vi "myRIO_BRig_RT_v0,72__PortC.vi"() -> ()   [LabVIEW 2014]
uses:
  <vilib>/Platform/TimedLoop/XDataNode/XDataNode.xnode
  <vilib>/Platform/TimedLoop/XDataNode/nitl_modes.ctl
  <vilib>/Platform/TimedLoop/XDataNode/XDNodeRunTimeDep.lvlib
  <vilib>/Platform/TimedLoop/XDataNode/wakeup.ctl
  <vilib>/Platform/TimedLoop/XDataNode/timing_clust.ctl
  <vilib>/rvi/interface/nirviReadWriteControl/nirviReadWriteControl.xnode
  <vilib>/rvi/interface/Simulation/niFpgaSimulationCallBeginRW.vi
  <vilib>/rvi/errors/niLvFpgaAdjustHostInterfaceError.vi
  <vilib>/rvi/interface/nirviCloseFPGA/nirviCloseFPGA.xnode
  <vilib>/myRIO/Instrument Drivers/Utilities/Utilities.lvlib
  <vilib>/rvi/interface/nirviOpenFPGA/nirviOpenFPGA.xnode
  myRIO_BRig_RT__Case_Exp_stateList.ctl
  <vilib>/WebDAVClient/Advanced/SessionHandle.ctl
  <vilib>/WebDAVClient/NI_WebDAV.lvlib
  myRIO_BRig_RT__Case_NonExp_stateList.ctl
  NiFpgaLv.dll
  <vilib>/Utility/error.llb/Error Cluster From Error Code.vi
  myRIO_BRig_FPGA_v3,60__PortC__build.lvbitx
  myRIO_BRig_FPGA_v3,60__PortC.vi
  <vilib>/FPGAPlugInAG/myRIO-1900/niLvFpga_Open_myRIO-1900.vi
  <vilib>/rvi/interface/common/dynamic/niFpgaDynamicAddResources.vi
  <vilib>/FPGAPlugInAG/Dynamic/niLvFpga_Close_Dynamic.vi
panel:
  in  "LC_Sel_All_Count":u16
  in  "LC_Sel_First_Count":u16
  in  "LC_Sel_All_Probability":u16
  in  "LC_Sel_All_Block":u16(slide) max=2 step=1 scale=0.0..2.0
  in  "LC_Sel_All_OnOff":bool
  in  "LC_Sel_First_Probability":u16
  in  "LC_Sel_First_Block":u16(slide) max=2 step=1 scale=0.0..2.0
  in  "LC_Sel_First_OnOff":bool
  in  "LC_Sel_All_Tdelay":u16
  in  "LC_Sel_First_Tdelay":u16
  out "I_connect_TCP":bool
  out "tempAI0":i16
  out "error out 5":errorcluster
  in  "get_countPerMS":bool
  in  "count_warmup_R_reset":bool
  in  "count_warmup_L_reset":bool
  out "count_warmup_R":u16
  out "count_warmup_L":u16
  out "SolenoidReward":bool
  in  "SolenoidProbability_L":u16=50 caption="Reward Time [ms]" min=1 max=1000 step=1
  in  "SolenoidProbability_R":u16=50 caption="Reward Time [ms]" min=1 max=1000 step=1
  out "output_PortA":dbl caption="LaserPower"
  out "error out 4":errorcluster
  in  "laser_power_step":dbl
  in  "laser_power_max":dbl
  in  "Recording":bool
  out "error out 3":errorcluster
  out "error out 2":errorcluster
  in  "laser_power_min":dbl
  in  "f_millisec2count":dbl=159.0
  in  "laser_Tshutter":dbl=2.0
  in  "laser_Freq":dbl=10.0
  in  "laser_Tpeak":dbl=2.0
  in  "laser_duration":u16
  out "error out":errorcluster
  in  "LC_Cue1_All_Count":u16
  in  "LC_Cue1_First_Count":u16
  in  "LC_Cue1_All_delayOpt":bool
  in  "LC_ENL1_All_delayOpt":bool
  in  "LC_ENL1_All_Count":u16
  in  "LC_ENL1_First_Count":u16
  in  "LC_Cue1_First_delayOpt":bool
  in  "LC_ENL1_First_delayOpt":bool
  in  "Tcycle_Cue_max":u16=1000 caption="Max" min=5 max=5000 step=5
  in  "Tcycle_Cue_min":u16=1000 caption="Min" min=5 max=5000 step=5
  in  "SendData":bool
  out "cSpout":enum16{"Left", "Right"}(ring) caption="Left or Right Spout"
  out "A4":u32 caption="LickCounter_Right"
  out "A2":u32 caption="LickCounter_Left"
  in  "laserResponse_wrong_LED":bool
  out "error_initTrial":errorcluster
  out "error_Selection_pre":errorcluster
  out "error_Selection":errorcluster
  out "SelectWrong":bool
  out "SelectReward":bool
  in  "Left(F)_or_Right(T)":bool
  in  "ignoreWrong":bool
  in  "SelectionState":bool
  in  "laserResponse_wrong":bool
  in  "laserResponse_reward":bool
  in  "laserResponse_reward_LED":bool
  out "nRewards_Right":u16 caption="# Rewards Total (Right)"
  out "nRewards_Left":u16 caption="# Rewards Total (Left)"
  out "nRewards_cur":u16 caption="# Rewards in Current Block"
  out "TpB_target":u16 caption="Target Trials Per Block"
  out "cState_NonExp":T1 caption="WarmUp State"
  out "iBlock":u16 caption="Current Block"
  out "cState":T2 caption="Experimental State"
  out "iTrial":u16 caption="Current Trial"
  in  "warmupType":u8(slide) max=2 step=1 scale=0.0..2.0
  in  "TestConnection":bool
  in  "warmup":bool caption="WarmUp"
  in  "Data Set Prefix":string="Exp1_TM2"
  out "Connected To Host?":bool
  in  "Host Password":string="sabalab"
  in  "Host UserName":string="Test2"
  in  "sp_RightSpout":u16(slide)=2 max=2 step=1 scale=0.0..2.0
  in  "sp_LeftSpout":u16(slide)=2 max=2 step=1 scale=0.0..2.0
  in  "BUR_max":u16 caption="Count Reward Structure  (0 = off)"
  in  "LC_Wrong_Probability":u16
  in  "LC_Wrong_Trial":u16(slide) max=2 step=1 scale=0.0..2.0
  in  "LC_Wrong_Block":u16(slide) max=2 step=1 scale=0.0..2.0
  in  "LC_Wrong_OnOff":bool
  in  "LC_Reward_Probability":u16
  in  "LC_Reward_Trial":u16(slide) max=2 step=1 scale=0.0..2.0
  in  "LC_Reward_Block":u16(slide) max=2 step=1 scale=0.0..2.0
  in  "LC_Reward_OnOff":bool
  in  "LC_Cue1_All_Probability":u16
  in  "LC_Cue1_All_Block":u16(slide) max=2 step=1 scale=0.0..2.0
  in  "LC_Cue1_All_OnOff":bool
  in  "LC_Cue1_First_Probability":u16
  in  "LC_Cue1_First_Block":u16(slide) max=2 step=1 scale=0.0..2.0
  in  "LC_Cue1_First_OnOff":bool
  in  "LC_ENL1_All_Probability":u16 max=100 step=1
  in  "LC_ENL1_All_Block":u16(slide) max=2 step=1 scale=0.0..2.0
  in  "LC_ENL1_All_OnOff":bool
  in  "LC_ENL1_First_Probability":u16 max=100 step=1
  in  "LC_ENL1_First_Block":u16(slide) max=2 step=1 scale=0.0..2.0
  in  "Tcycle_Timeout":u16=1000 caption="Timeout Time [ms]" min=10 max=10000 step=1
  in  "Tcycle_Wrong":u16=1000 caption="Wrong Time [ms]" min=10 max=10000 step=1
  in  "Tcycle_Selection":u16=1000 caption="Answer Time [ms]" min=1 max=10000 step=1
  in  "Tcycle_RewardPost":u16=1000 caption="Consumption Time [ms]" min=250 max=10000 step=250
  in  "Tcycle_Reward_L":u16=500 caption="Reward Time [ms]" min=1 max=1000 step=1
  in  "Tcycle_Reward_R":u16=500 caption="Reward Time [ms]" min=1 max=1000 step=1
  in  "TpB_Max_R":u16=4 caption="Max TrialsPerBlock" min=1 max=12 step=1
  in  "TpB_Min_R":u16=4 caption="Min TrialsPerBlock" min=1 max=12 step=1
  in  "TpB_Max_L":u16=4 caption="Max TrialsPerBlock" min=1 max=12 step=1
  in  "TpB_Min_L":u16=4 caption="Min TrialsPerBlock" min=1 max=12 step=1
  in  "BUR_min":u16 caption="Count Reward Structure\n(0 = off)"
  in  "TrialUntilReward":bool caption="Ignore Wrong Selection"
  in  "CueCycles":u16=1 caption="Cue Structure" min=1 max=1 step=1
  in  "MTrig_Laser_Tcycle":u16=10 caption="Time [ms]"
  in  "MTrig_Laser_trig":bool
  in  "MTrig_Audio_trig__R":bool caption="Trigger Audio"
  in  "MTrig_Audio_trig__L":bool caption="Trigger Audio"
  in  "RewCalib_Trig_R":bool caption="Calibrate_R"
  in  "RewCalib_Trig_L":bool caption="Calibrate_L"
  in  "MTrig_Solenoid_Tcycle__R":u16=300 caption="Time [ms]"
  in  "MTrig_Solenoid_Tcycle__L":u16=300 caption="Time [ms]"
  in  "MTrig_Solenoid_trig__R":bool caption="Solenoid"
  in  "MTrig_Solenoid_trig__L":bool caption="Solenoid"
  in  "STOP_abort":bool caption="Stop LabView\n(Stops myRio and FPGA)"
  in  "STOP_endBlock":bool caption="Stop Experiment\n@ End of Block"
  in  "STOP_endTrial":bool caption="Stop Experiment\n@ End of Trial"
  in  "START":bool caption="Start Experiment"
  in  "Tcycle_CuePenalty":u16=1000 caption="Penalty" min=1 max=10000 step=1
  in  "Audio_Amp__R":u16=100 caption="Amp"
  in  "Audio_Freq__R":u8=5 caption="Freq [kHz]" max=14 step=1
  in  "Audio_Amp__L":u16=100 caption="Amp"
  in  "Audio_Freq__L":u8=5 caption="Freq [kHz]" max=14 step=1
  in  "LC_Wrong_Tdelay":u16
  in  "LC_Cue1_All_Tdelay":u16
  in  "LC_ENL1_All_Tdelay":u16
  in  "LC_Reward_Tdelay":u16
  in  "LC_Cue1_First_Tdelay":u16
  in  "LC_ENL1_First_Tdelay":u16
  in  "LC_ENL1_First_OnOff":bool
  in  "Tcycle_ENLPenalty":u16=100 caption="Penalty" min=10 max=10000 step=10
  in  "Tcycle_ENL_max":u16=1000 caption="Max" min=250 max=10000 step=250
  in  "Tcycle_ENL_min":u16=1000 caption="Min" min=250 max=10000 step=250
  # "Experimental Run"
  # "Experiment Task Structure"
  # "Current State"
  # "Timing [ms]"
  # "Global Parameters\n \n   WarmUp State                                            Lick Counter"
  # "Min            Max            Penalty"
  # "(1) = Switching\n(2) = Two Choice"
  # "Enforced\nNonLick"
  # "Left                    Right"
  # "Cue"
  # "Experimental State"
  # "Communication (Host PC)"
  # "WarmUp"
  # "Selection\n \n \nReward\n    Dispense\n    Time\n \n    Dispense\n    Probability\n \n    Consumption\n    Time\n \nWrong Choice\n \n \nTimeout Penalty"
  # "Trial Parameters\n \n   Left/Right        Give Reward?        Laser Power [V]"
  # "Left                  Right"
  # "Min"
  # "Max"
  # "Block                   Trial            Target Trials       # Rewards \n                                                            Per Block             Current"
  # "Trial Per Block Structure \n               Left                        Right"
  # "Min"
  # "# Rewards Total\n                                                                  Left                    Right"
  # "Recording Rig"
  # "FPGA Conv."
  # "Cue then reward (no lick)\n \nLeft                    Right"
  # "Max"
  # "FPGA count per ms"
  # "Laser Control\n\n                               On/Off      Block        Probability [%]   Delay [ms]                              Count"
  # "Manual Control"
  # "Enforced\nNonLick\n      1"
  # "Solenoid\n \nLeft              Right"
  # "Speaker\n \nLeft                    Right"
  # "Laser"
  # "from end"
  # "Switch\nTrial"
  # "from start"
  # "from end"
  # "NonSwitch\nTrials"
  # "Time\n[ms]"
  # "Time\n[ms]"
  # "from start"
  # "Time = Cue Min"
  # "Cue 1"
  # "Power = Min"
  # "from end"
  # "Switch\nTrial"
  # "from start"
  # "Speaker Parameters"
  # "Laser Parameters"
  # "Left                  Right"
  # "from end"
  # "Frequency\n[Hz]"
  # "NonSwitch\nTrials"
  # "Frequency\n[kHz]"
  # "from start"
  # "Timing [ms]\n Duration     Peak Width   Shutter"
  # "Selection"
  # "Amp\n(0 - 32,000)"
  # "Switch\nTrial"
  # "Laser Power [V]\nMin          Max              Step"
  # "Speaker\nPattern\nDuring Cue"
  # "NonSwitch\nTrials"
  # "Selection Reward"
  # "Selection Wrong"
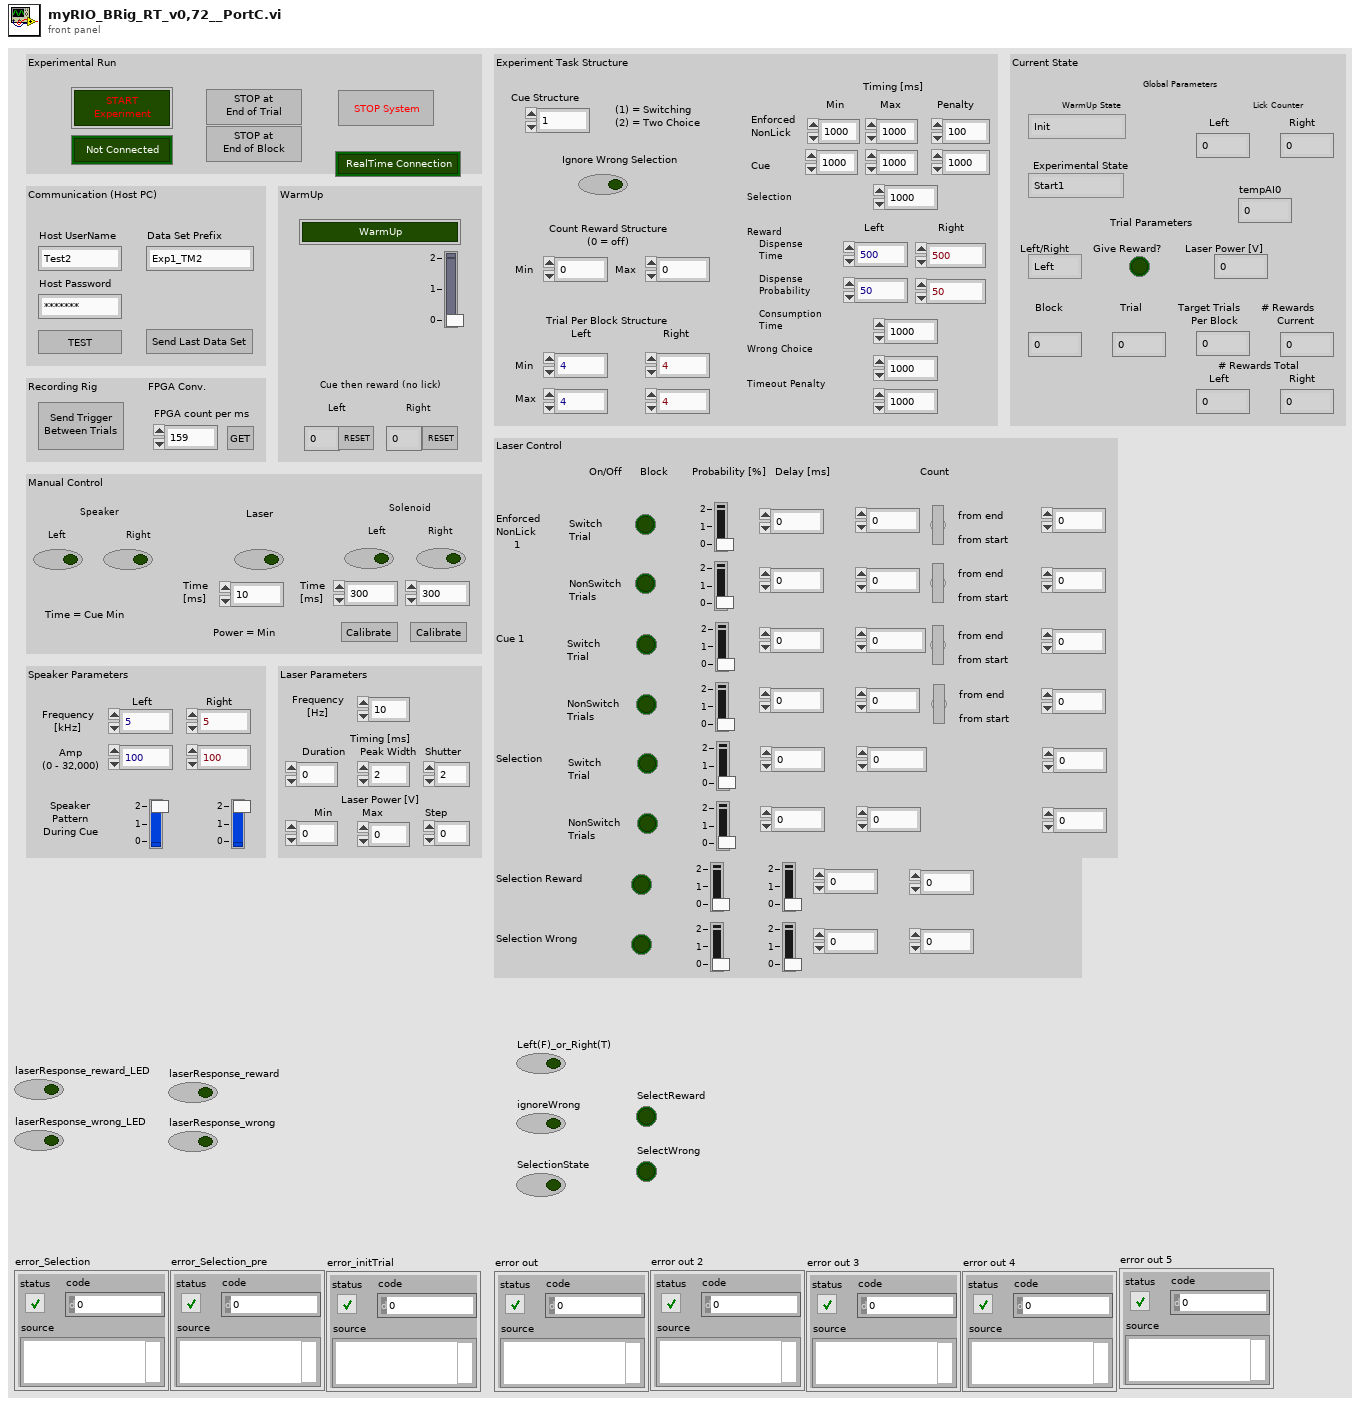
[diagram p1: front panel]
types:
  T1 = typedef "myRIO_BRig_RT__Case_NonExp_stateList.ctl" = enum16{"Init", "UploadSettings_pre", "UploadSettings_Read_dataExp", "UploadSettings_dataExp_1", "UploadSettings_Read_dataLC", "UploadSettings_dataLC_1", "UploadSettings_dataLC_2", "UploadSettings_Read_dataMTrig", "UploadSettings_dataMTrig_1", "UploadSettings_post", "Idle_pre", "IdleEmpty", "IdleEmpty2", "IdleEmpty3", "IdleEmpty4", "Idle", "Idle_2", "Idle_3", "Idle_4", "Idle_post", "Cue_pre__pre", "Cue_pre", "Cue", "Cue_post", "RewardCalibration_pre", "DispenseWater_pre__pre", "DispenseWater_pre", "DispenseWater", "DispenseWater_post", "TestConnection", "SendData", "Get_FPGA_count_per_ms", "End"}
  T2 = typedef "myRIO_BRig_RT__Case_Exp_stateList.ctl" = enum16{"Start1", "Start2", "Start3", "saveSettings1", "saveSettings2", "saveSettings3", "saveSettings4_LC_ENL", "saveSettings5_LC_Cue", "saveSettings6_LC_Other", "setSettings_Audio", "setSettings_Laser", "initBlock_pre", "initBlock", "initBlock2", "initBlock_post", "initTrial_pre", "initTrial", "initTrial2", "initTrial3", "initTrial4", "initTrial_LC_ENL1", "initTrial_LC_Cue1", "initTrial_LC_Sel", "initTrial_post", "ENL1_pre", "ENL1", "ENL1_post", "ENL1Penalty_pre", "ENL1Penalty", "ENL2_pre", "ENL2", "ENL2Penalty_pre", "ENL2Penalty", "Cue1_pre", "Cue1", "Cue1_post", "Cue1Penalty_pre", "Cue1Penalty", "Cue2_pre", "Cue2", "Cue2Penalty_pre", "Cue2Penalty", "Selection_pre", "Selection", "Select_post", "SelectReward_pre", "SelectReward", "SelectRewardPost_pre", "SelectRewardPost", "SelectWrong_pre", "SelectWrong", "SelectWrong_post", "SelectTimeout_pre", "SelectTimeout", "SelectTimeout_post", "endTrial_pre", "endTrial1", "endTrial2", "endTrial3", "endTrial_post", "endBlock_pre", "endBlock", "endBlock_post", "endExp", "commConnect", "commUpload_pre", "commUpload_dataBlock", "commUpload_dataCurrent", "commUpload_dataExp", "commUpload_dataLC", "commUpload_dataTrial", "commUpload_post", "saveData_pre", "saveData_dataBlock", "saveData_dataCurrent", "saveData_dataExp", "saveData_dataLC", "saveData_dataTrial", "saveData_post", "empty_endBlock1", "empty_endBlock2", "empty_endTrial1", "empty_endTrial2", "empty_endTrial3", "empty_endTrial4", "empty_endTrial5"}
  T3 = typedef "XDNodeRunTimeDep.lvlib/timing_clust.ctl" = cluster{"Expected End [f-1]":u64, "Actual End [f-1]":u64, "Finished Late? [f-1]":bool, "Expected End [i-1]":u64, "Actual End [i-1]":u64, "Finished Late? [i-1]":bool, "Expected Start [i]":u64, "Actual Start [i]":u64, "Expected Start [f]":u64, "Actual Start [f]":u64, "Source Name":string, "Structure Name":string, "Period":i64, "Deadline":i64, "Offset":i64, "Start":i64, "Priority":i32, "Timeout":i32, "Mode":T4, "Wakeup Reason":T5, "Error":errorcluster, "Source Type":string, "Secondary Source Type":string, "Global End Time":u64, "Global Start Time":u64, "Frame Duration":u64, "Iteration Duration":u64, "Assigned CPU":i32, "I/O Scan Engine Mode":u32}
  T4 = typedef "XDNodeRunTimeDep.lvlib/nitl_modes.ctl" = enum32{"No Change", "Process missed periods, maintain original phase", "Discard missed periods, maintain original phase", "Process missed periods, ignore original phase", "Discard missed periods, ignore original phase"}
  T5 = typedef "XDNodeRunTimeDep.lvlib/wakeup.ctl" = enum32{"Normal", "Aborted", "Asynchronous wakeup", "Timing source error", "Timed loop error", "Timeout"}
  T6 = typedef "NI_WebDAV.lvlib/SessionHandle.ctl" = refnum<k1>
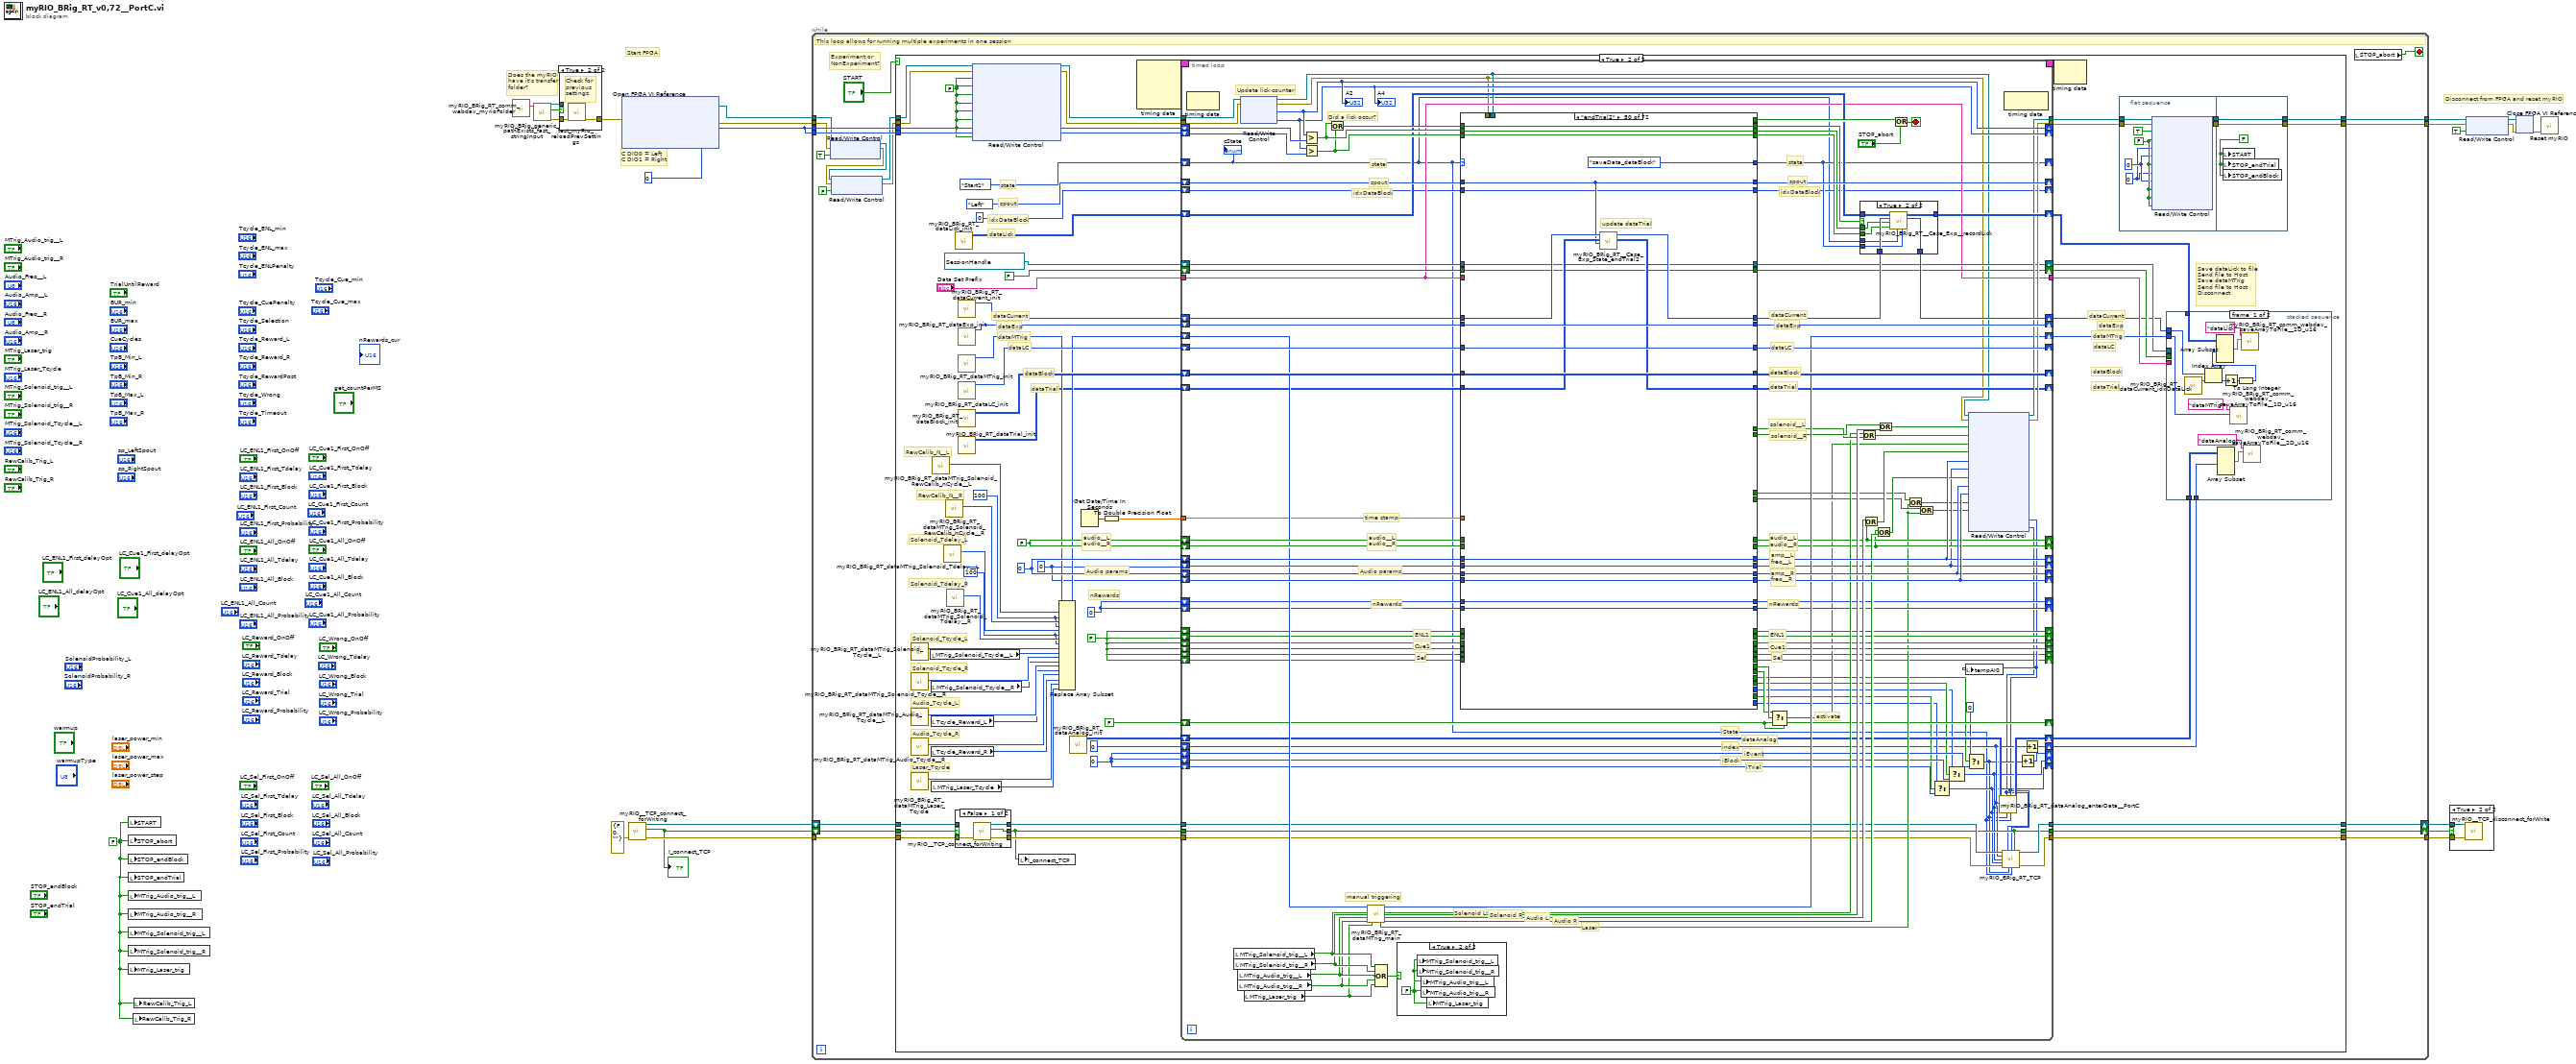
[diagram p0: block diagram]
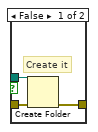
[diagram p3: hidden frame]
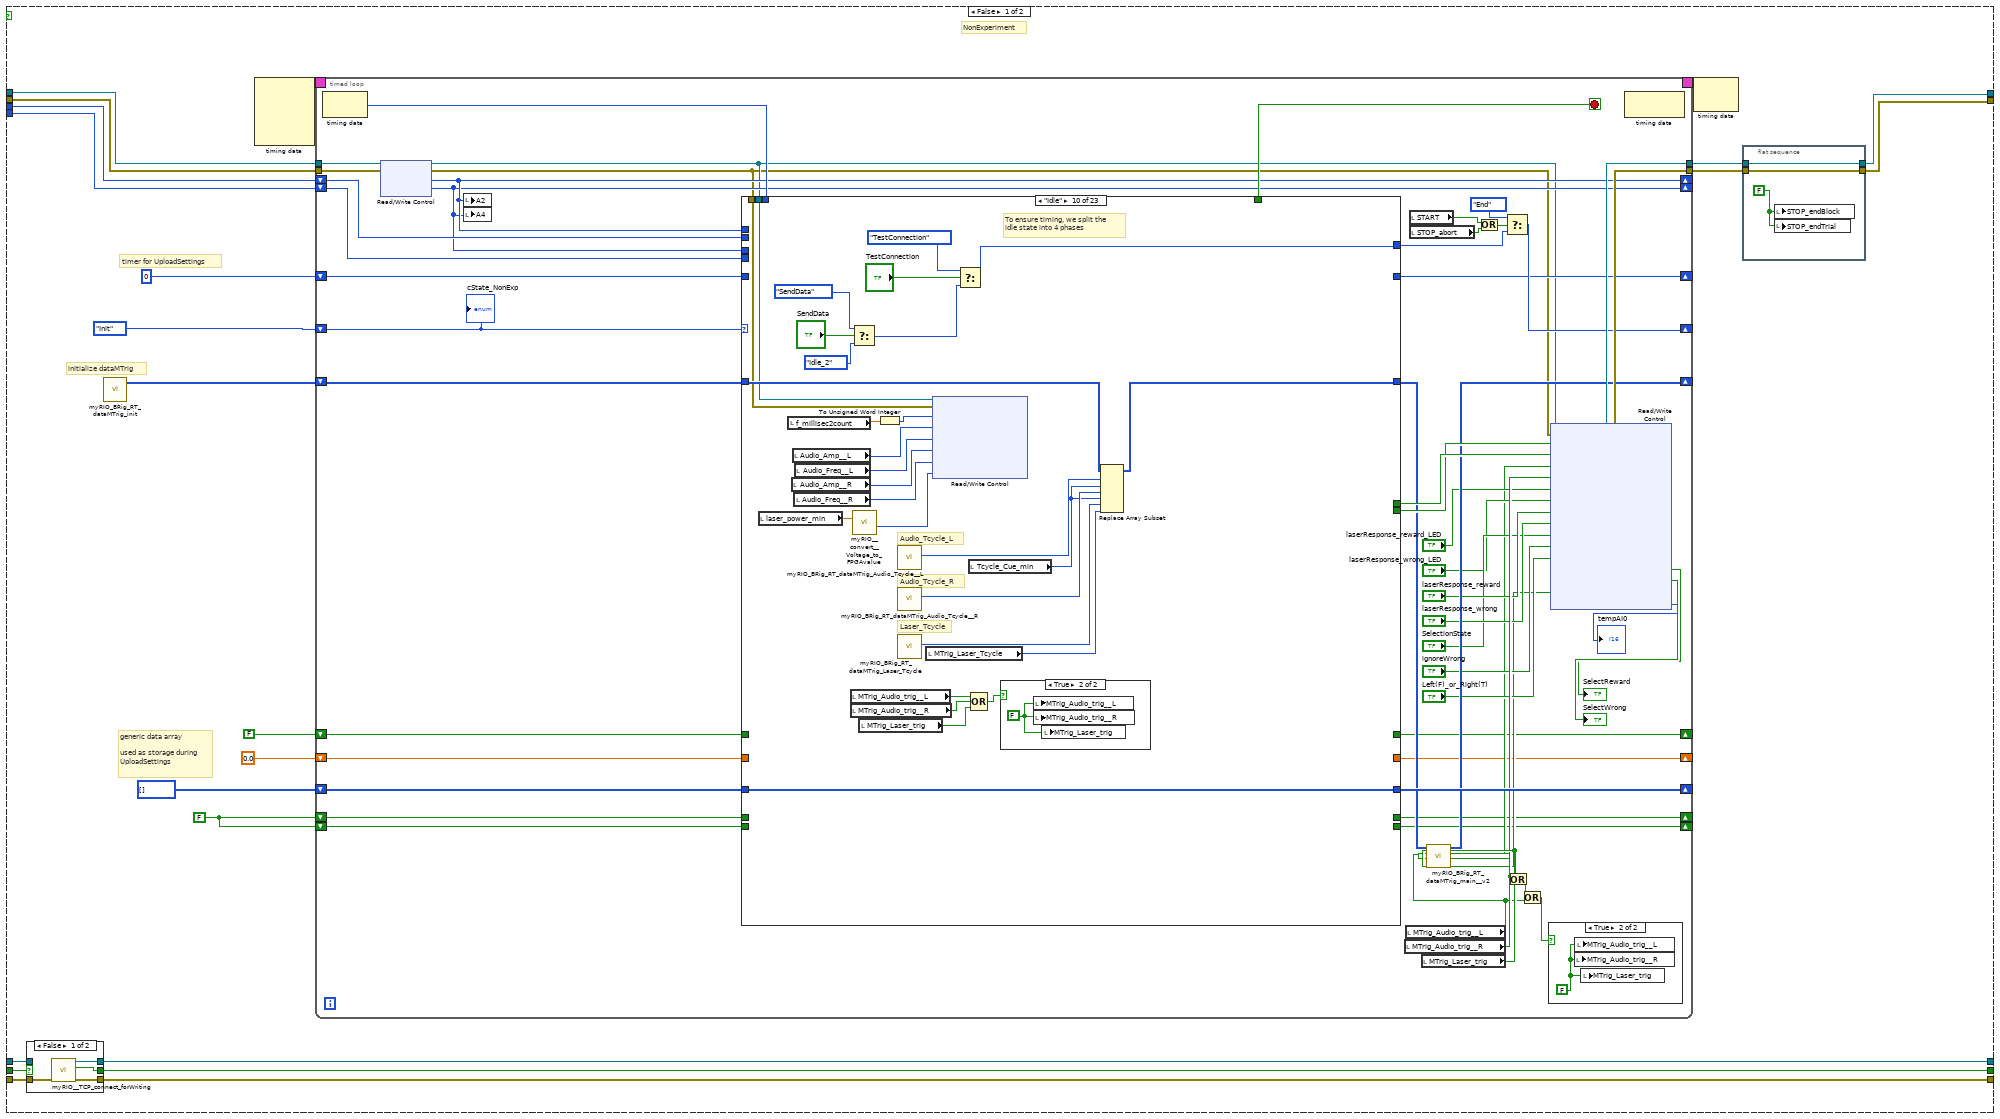
[diagram p4: hidden frame]
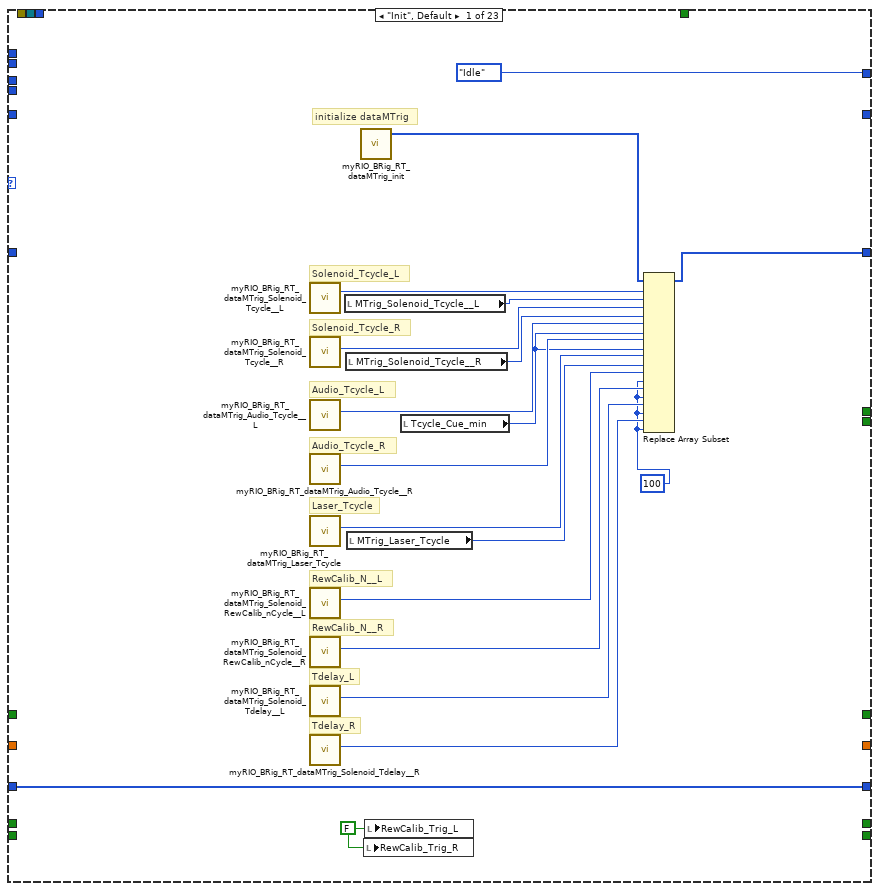
[diagram p7: hidden frame]
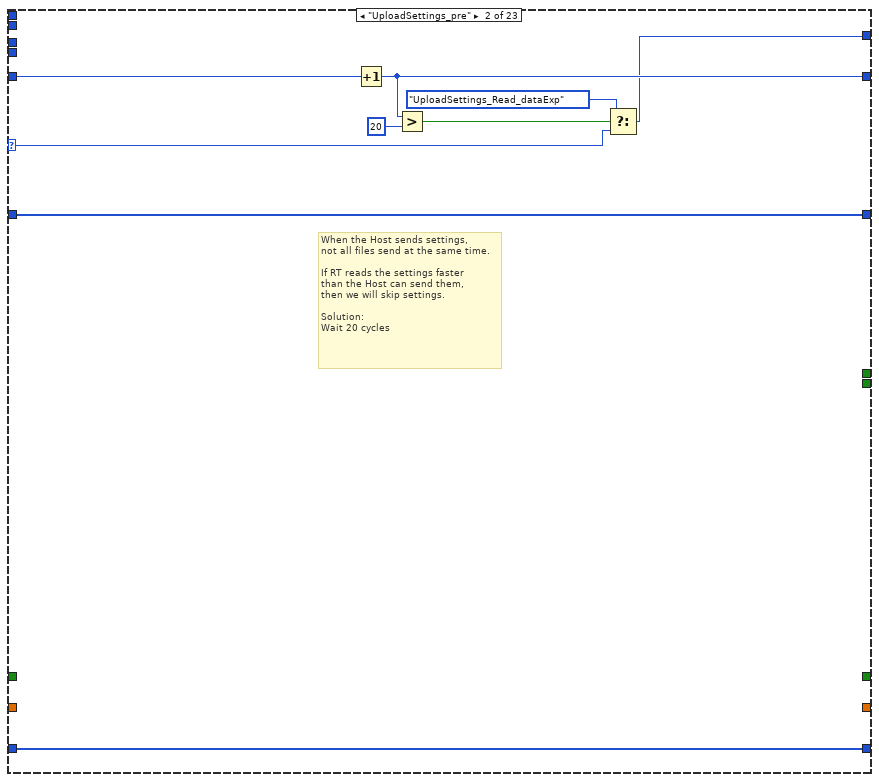
[diagram p8: hidden frame]
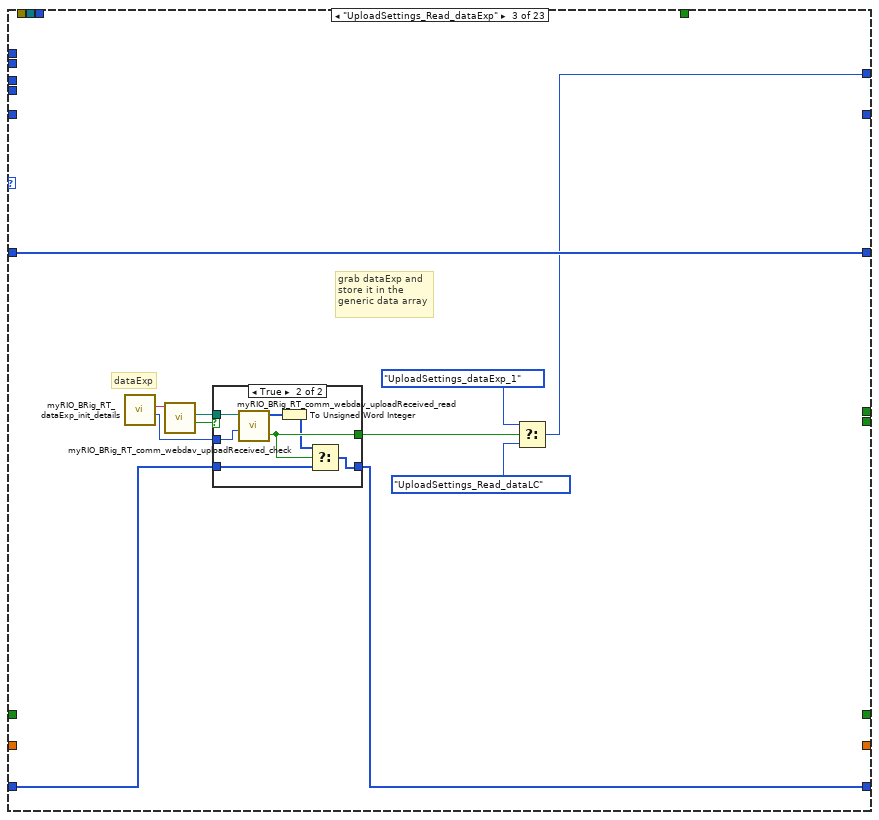
[diagram p9: hidden frame]
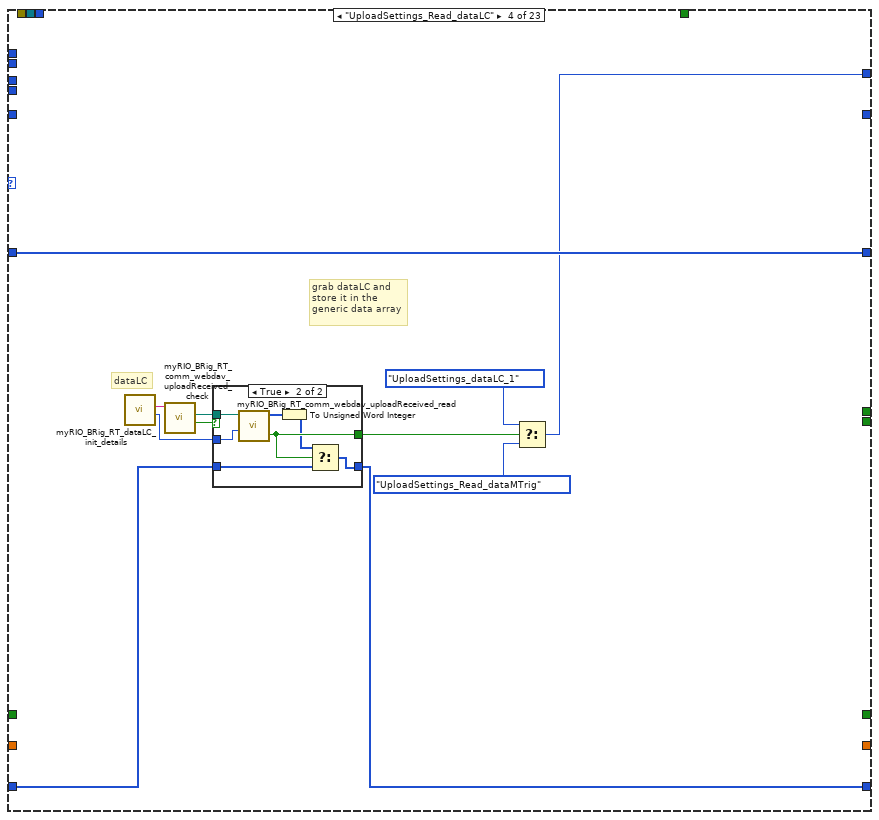
[diagram p11: hidden frame]
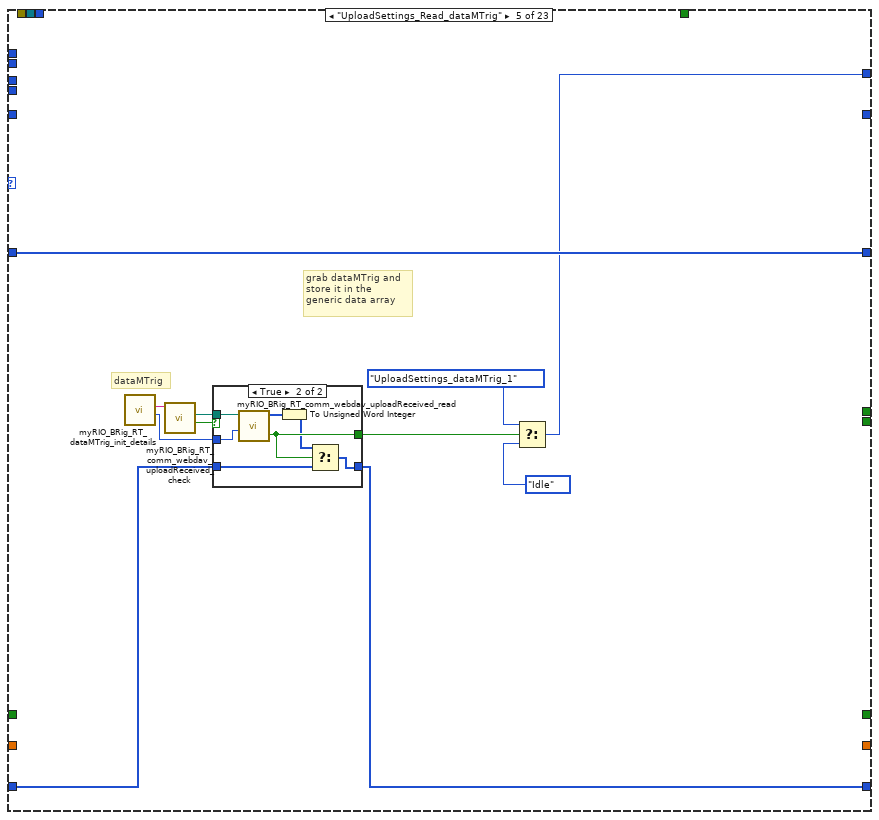
[diagram p13: hidden frame]
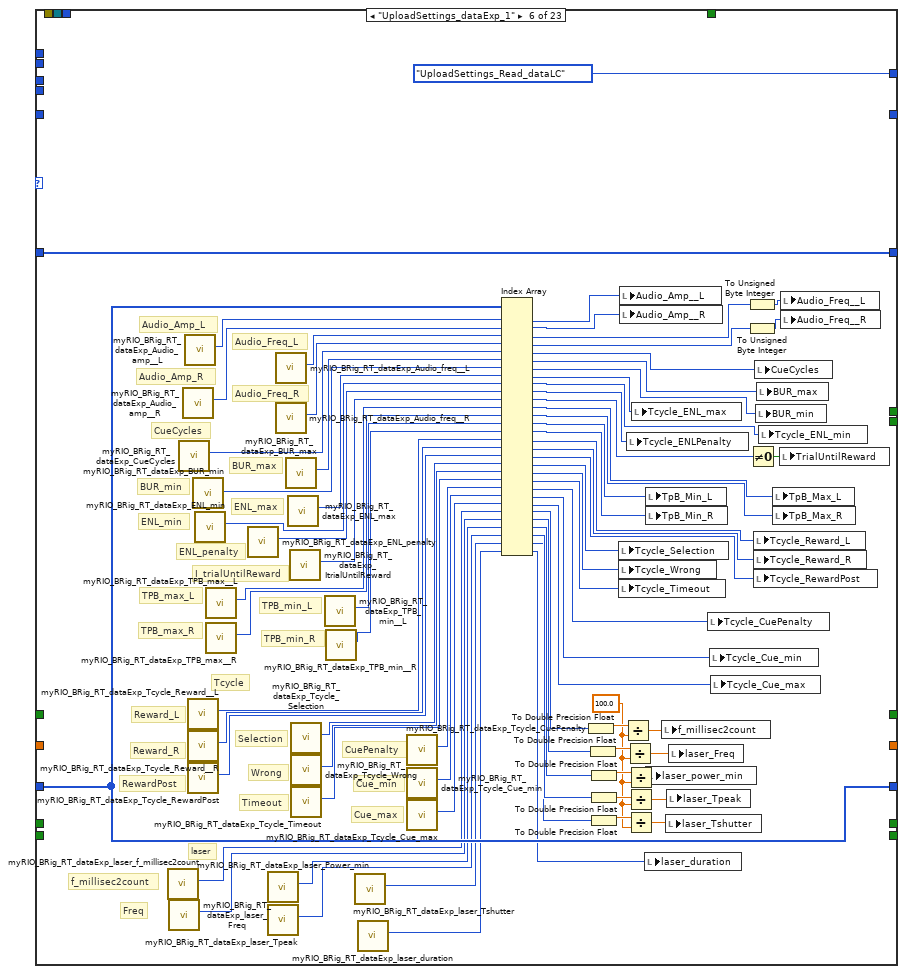
[diagram p15: hidden frame]
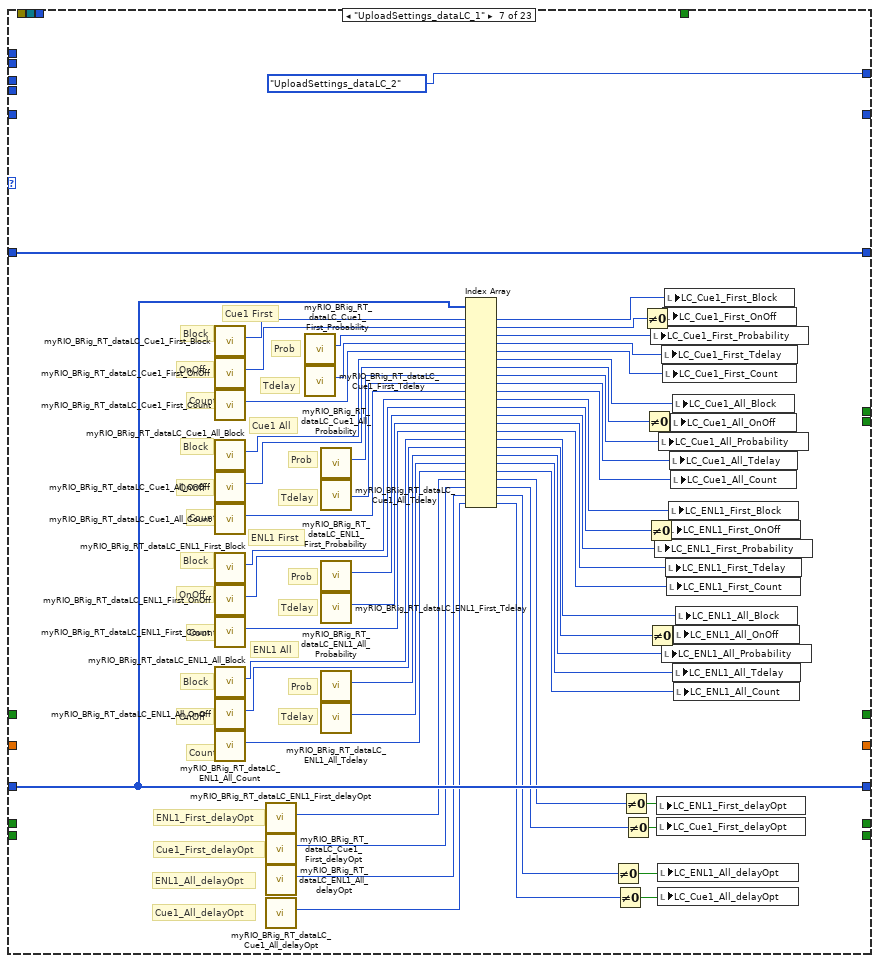
[diagram p16: hidden frame]
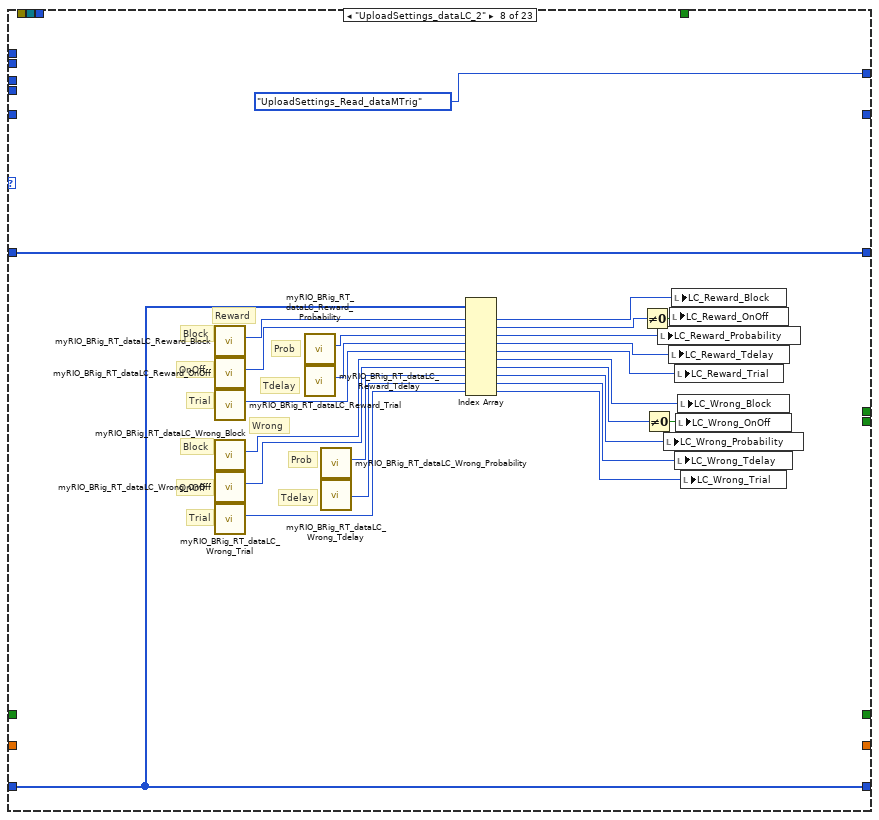
[diagram p17: hidden frame]
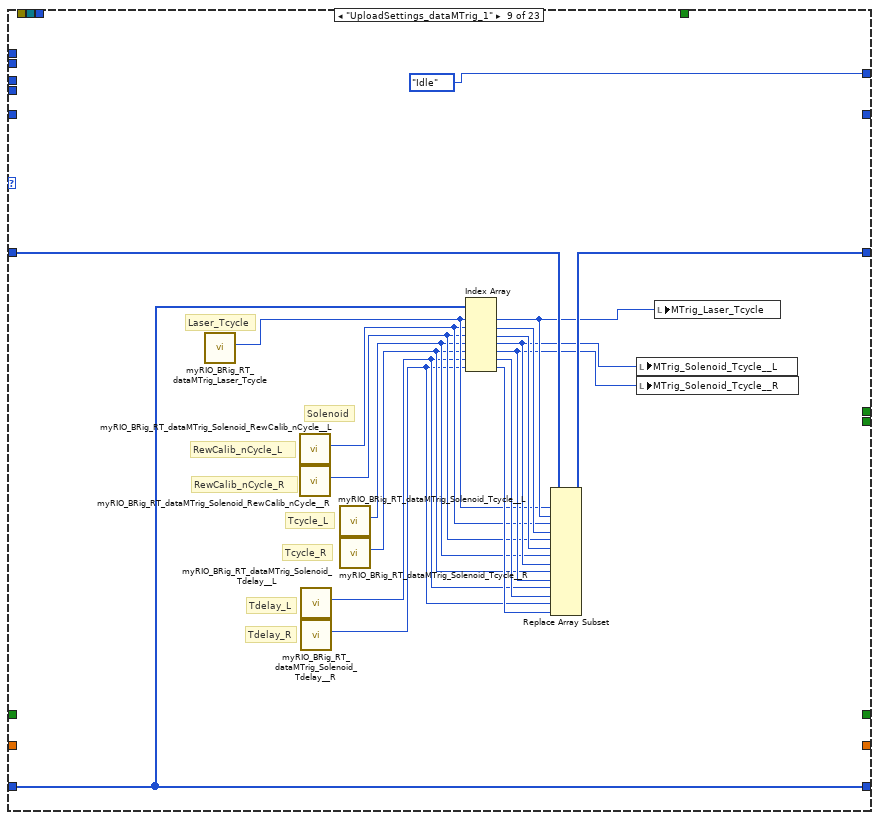
[diagram p18: hidden frame]
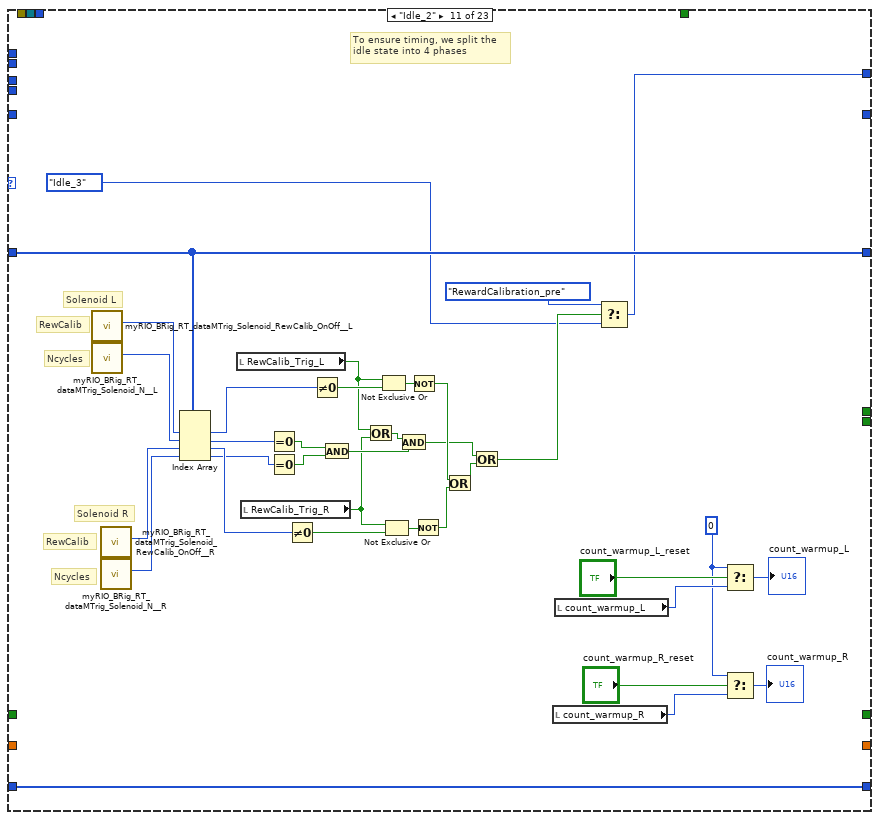
[diagram p20: hidden frame]
diagram:
  w16 = u32 0
  w13 = FALSE
  # "Does the myRIO\nhave it's transfer\nfolder?"
  # "C DIO0 = Left\nC DIO1 = Right"
  # "Start FPGA"
  # "Disconnect from FPGA and reset myRIO"
  n1 = local write "START"(w13) -> ()
  n2 = local write "STOP_abort"(w13) -> ()
  n3 = local write "STOP_endBlock"(w13) -> ()
  n4 = local write "STOP_endTrial"(w13) -> ()
  n5 = local write "MTrig_Audio_trig__L"(w13) -> ()
  n6 = local write "MTrig_Audio_trig__R"(w13) -> ()
  n7 = local write "MTrig_Solenoid_trig__L"(w13) -> ()
  n8 = local write "MTrig_Solenoid_trig__R"(w13) -> ()
  n9 = local write "MTrig_Laser_trig"(w13) -> ()
  n10 = local write "RewCalib_Trig_R"(w13) -> ()
  n11 = local write "RewCalib_Trig_L"(w13) -> ()
  n12 = call "myRIO_BRig_RT_comm_webdav_myrioFolder.vi"() -> ("output_myrioFolder"=w12:string)  [unwired: 11 in]
  n13 = call "myRIO_BRig_generic_pathExists_fast_stringInput.vi"("input_filePath"=w12) -> ("output_error"=w11:errorcluster, "output_Iexist"=w10:bool, "output_filePath"=w9:path)  [unwired: 8 in]
  n14 = case shown="True" w10 {
    tunnel: w9 -> [w25 _]
    tunnel: w11 -> [w24 w27]
    tunnel: [w23 w26] -> w7
    frame False {
      # "Create it"
      n15 = Create Folder(path (use dialog)=w25, error in=w24) -> (error out=w23:errorcluster)  [unwired: 1 in, 2 out]
    }
    frame True {
      # "Check for\nprevious\nsettings"
      n16 = call "test_myRio_reloadPrevSettings.vi"("input_error"=w27) -> ("output_error"=w26:errorcluster)  [unwired: 10 in]
    }
  }
  n17 = xnode "Open FPGA VI Reference"("error in"=w7) -> ("FPGA VI Reference Out"=w18:refnum<k20>, "error out"=w17:errorcluster)  [unwired: 1 in]
  n18 = call "myRIO__TCP_connect_forWriting.vi"("input_error"=errorcluster {"status"=FALSE, "code"=0, "source"=""}) -> ("output_error"=w5:errorcluster, "output_connected"=w4:bool, "output_hTCP"=w8:refnum<k5>)  [unwired: 8 in]
  "I_connect_TCP" <- w4
  n19 = while {
    tunnel: w18 -> [w37]
    tunnel: w17 -> [w42]
    tunnel: w16 -> [w45]
    tunnel: w16 -> [w44]
    tunnel: [w35] -> w15
    tunnel: [w34] -> w14
    shift-right: [w31] -> w3
    shift-left: w4 -> [w32]
    tunnel: w5 -> [w30]
    shift-right: [w29] -> w2
    shift-left: w8 -> [w33]
    tunnel: [w28] -> w1
    stop <- w43 stop-if-true
    # "Experiment or\nNonExperiment?"
    # "This loop allows for running multiple experiments in one session"
    n20 = xnode "Read/Write Control"("FPGA VI Reference In"=w37, "error in"=w42, "Counts_Reset"=TRUE) -> ("FPGA VI Reference Out"=w39:refnum<k20>, "error out"=w40:errorcluster)
    n21 = xnode "Read/Write Control"("FPGA VI Reference In"=w39, "error in"=w40, "Counts_Reset"=FALSE) -> ("FPGA VI Reference Out"=w36:refnum<k20>, "error out"=w38:errorcluster)
    n22 = case shown="True" "START" {
      tunnel: w45 -> [w66 w992]
      tunnel: w44 -> [w65 w991]
      tunnel: w38 -> [w63 w942]
      tunnel: w36 -> [w64 w941]
      tunnel: [w61 w988] -> w35
      tunnel: [w59 w983] -> w34
      tunnel: w33 -> [w52 w927]
      tunnel: [w50 w932] -> w29
      tunnel: w32 -> [w51 w930]
      tunnel: [w49 w931] -> w31
      tunnel: w30 -> [w53 w929]
      tunnel: [w48 w925] -> w28
      frame False {
        w56 = FALSE
        # "generic data array\n\nused as storage during\nUploadSettings"
        # "timer for UploadSettings"
        # "initialize dataMTrig"
        # "NonExperiment"
        n23 = case shown="False" w51 {
          selector: w51 -> [_ w75]
          tunnel: w53 -> [w72 w77]
          tunnel: [w73 w77] -> w48
          tunnel: w52 -> [_ w76]
          tunnel: [w74 w76] -> w50
          tunnel: [w71 w75] -> w49
          frame False {
            n24 = call "myRIO__TCP_connect_forWriting.vi"("input_error"=w72) -> ("output_error"=w73:errorcluster, "output_connected"=w71:bool, "output_hTCP"=w74:refnum<k5>)  [unwired: 8 in]
          }
          frame True {
          }
        }
        n25 = call "myRIO_BRig_RT_dataMTrig_init.vi"() -> ("output_dataMTrig"=w67:u16[])  [unwired: 5 in]
        n26 = node-c288() -> (w70:T3)  [unwired: 4 in]
        n27 = timed-loop {
          timing: w70 -> [_]
          timing-out: [_] -> w69
          shift-right: [w121] -> _
          shift-left: w67 -> [w133]
          shift-right: [w110] -> _
          shift-left: myRIO_BRig_RT__Case_NonExp_stateList."Init" ("Enum") -> [w127]
          shift-right: [w94] -> _
          shift-left: w66 -> [w95]
          shift-right: [w92] -> _
          shift-left: w65 -> [w93]
          tunnel: [w129] -> w62
          tunnel: [w128] -> w60
          tunnel: w63 -> [w131]
          tunnel: w64 -> [w130]
          shift-right: [w126] -> _
          shift-left: u16[] [] ("output_data") -> [w125]
          shift-right: [w96] -> _
          shift-left: u16 0 ("Audio_Amp__L") -> [w97]
          shift-right: [w89] -> _
          shift-left: w56 -> [w91]
          shift-right: [w88] -> _
          shift-left: w56 -> [w90]
          shift-right: [w84] -> _
          shift-left: FALSE -> [w85]
          shift-right: [w82] -> _
          shift-left: 0.0 -> [w83]
          stop <- w134 stop-if-true
          n28 = node-c288() -> (w132:i64)  [unwired: 1 in]
          n29 = xnode "Read/Write Control"("FPGA VI Reference In"=w130, "error in"=w131) -> ("FPGA VI Reference Out"=w87:refnum<k20>, "error out"=w86:errorcluster, "A2_LickL"=w94:u32, "A4_LickR"=w92:u32)
          n30 = local write "A2"(w94) -> ()
          n31 = local write "A4"(w92) -> ()
          n32 = case shown="\"Idle\"" w127 {
            selector: w127 -> [_ w159 _ _ _ _ _ _ _ _ _ _ _ _ w590 _ _ w798 _ _ _ w873 w917]
            tunnel: [myRIO_BRig_RT__Case_NonExp_stateList."Idle" ("Enum") w157 w164 w183 w202 myRIO_BRig_RT__Case_NonExp_stateList."UploadSettings_Read_dataLC" ("Enum") myRIO_BRig_RT__Case_NonExp_stateList."UploadSettings_dataLC_2" ("Enum") myRIO_BRig_RT__Case_NonExp_stateList."UploadSettings_Read_dataMTrig" ("f") myRIO_BRig_RT__Case_NonExp_stateList."Idle" ("Enum") w421 w438 w477 w558 myRIO_BRig_RT__Case_NonExp_stateList."Cue" ("t") w585 myRIO_BRig_RT__Case_NonExp_stateList."DispenseWater_pre" ("Enum") w743 w796 w819 myRIO_BRig_RT__Case_NonExp_stateList."Idle" ("Enum") myRIO_BRig_RT__Case_NonExp_stateList."Idle" ("Enum") w872 w917] -> w111
            tunnel: [w146 w156 w174 w193 w212 w297 w356 w381 w397 w425 w453 w482 w556 w574 w591 w653 w780 w803 w830 w865 w871 w884 w915] -> w122
            tunnel: [_ _ _ _ _ _ _ _ _ _ _ _ _ _ _ _ _ _ _ _ _ _ TRUE] -> w134
            tunnel: w133 -> [_ w156 w174 w193 w212 w297 w356 w381 w398 w424 w453 w483 w556 w575 w592 w639 w776 w804 w831 w865 w871 w884 w915]
            tunnel: w132 -> [_ _ _ _ _ _ _ _ _ _ _ _ _ _ _ _ _ w808 _ _ _ _ _]
            tunnel: [w139 w155 w165 w184 w203 w246 w312 w357 w382 w416 w437 w471 w555 w564 w599 w634 w728 w781 w812 w857 w869 w883 w914] -> w126
            tunnel: w125 -> [w139 w155 w166 w185 w204 w246 w312 w357 w382 w416 w437 w471 w555 w564 w599 w634 w728 w781 w812 w857 w869 w883 w914]
            tunnel: [_ _ _ _ _ _ _ _ _ _ _ _ _ _ _ _ _ w805 _ _ _ _ _] -> w124
            tunnel: [_ _ _ _ _ _ _ _ _ _ _ _ _ _ _ _ _ w787 _ _ _ _ _] -> w123
            tunnel: w97 -> [_ w163 _ _ _ _ _ _ _ _ _ _ _ _ _ _ _ _ _ _ _ _ _]
            tunnel: [_ w162 _ _ _ _ _ _ _ _ _ _ _ _ _ _ _ _ _ _ _ _ _] -> w96
            tunnel: w95 -> [_ _ _ _ _ _ _ _ _ _ _ _ _ _ w596 _ _ _ _ _ _ _ _]
            tunnel: w94 -> [_ _ _ _ _ _ _ _ _ _ _ _ _ _ w597 _ _ _ _ _ _ _ _]
            tunnel: w93 -> [_ _ _ _ _ _ _ _ _ _ _ _ _ _ w594 _ _ _ _ _ _ _ _]
            tunnel: w92 -> [_ _ _ _ _ _ _ _ _ _ _ _ _ _ w595 _ _ _ _ _ _ _ _]
            tunnel: w91 -> [_ _ _ _ _ _ _ _ _ _ _ _ _ _ w582 _ _ _ _ _ _ _ _]
            tunnel: w90 -> [_ _ _ _ _ _ _ _ _ _ _ _ _ _ w581 _ _ _ _ _ _ _ _]
            tunnel: [_ _ _ _ _ _ _ _ _ _ _ _ _ w563 w582 _ _ _ _ _ _ _ _] -> w89
            tunnel: [_ _ _ _ _ _ _ _ _ _ _ _ _ w562 w581 _ _ _ _ _ _ _ _] -> w88
            tunnel: w87 -> [_ _ _ _ _ _ _ _ _ w407 _ _ _ _ _ _ _ _ _ _ _ w878 _]
            tunnel: w86 -> [_ _ _ _ _ _ _ _ _ w406 _ _ _ _ _ _ _ _ _ _ _ w877 _]
            tunnel: w85 -> [_ _ _ _ _ _ _ _ _ _ _ _ _ _ _ _ _ _ _ _ _ w882 _]
            tunnel: [_ _ _ _ _ _ _ _ _ _ _ _ _ _ _ _ _ _ _ _ _ TRUE _] -> w84
            tunnel: w83 -> [_ _ _ _ _ _ _ _ _ _ _ _ _ _ _ _ _ _ _ _ _ w880 _]
            tunnel: [_ _ _ _ _ _ _ _ _ _ _ _ _ _ _ _ _ _ _ _ _ w879 _] -> w82
            frame "Init", Default {
              w140 = FALSE ("RewCalib_Trig_L")
              w136 = u16 100 ("new element/subarray")
              # "Tdelay_R"
              # "Tdelay_L"
              # "RewCalib_N__R"
              # "RewCalib_N__L"
              # "Solenoid_Tcycle_R"
              # "Solenoid_Tcycle_L"
              # "Laser_Tcycle"
              # "Audio_Tcycle_R"
              # "Audio_Tcycle_L"
              # "initialize dataMTrig"
              n33 = call "myRIO_BRig_RT_dataMTrig_Solenoid_Tcycle__L.vi"() -> ("output_Solenoid_Tcycle__L"=w148:i32)  [unwired: 11 in]
              n34 = call "myRIO_BRig_RT_dataMTrig_Solenoid_Tcycle__R.vi"() -> ("output_Solenoid_Tcycle__R"=w149:i32)  [unwired: 11 in]
              n35 = call "myRIO_BRig_RT_dataMTrig_Audio_Tcycle__L.vi"() -> ("output_Audio_Tcycle__L"=w150:i32)  [unwired: 11 in]
              n36 = call "myRIO_BRig_RT_dataMTrig_Audio_Tcycle__R.vi"() -> ("output_Audio_Tcycle__R"=w151:i32)  [unwired: 11 in]
              n37 = call "myRIO_BRig_RT_dataMTrig_Laser_Tcycle.vi"() -> ("output_Laser_Tcycle"=w152:i32)  [unwired: 11 in]
              n38 = call "myRIO_BRig_RT_dataMTrig_Solenoid_RewCalib_nCycle__L.vi"() -> ("output_Solenoid_RewCalib_nCycle__L"=w144:i32)  [unwired: 11 in]
              n39 = call "myRIO_BRig_RT_dataMTrig_Solenoid_RewCalib_nCycle__R.vi"() -> ("output_Solenoid_RewCalib_nCycle__R"=w143:i32)  [unwired: 11 in]
              n40 = call "myRIO_BRig_RT_dataMTrig_Solenoid_Tdelay__L.vi"() -> ("output_Solenoid_Tdelay__L"=w142:i32)  [unwired: 11 in]
              n41 = call "myRIO_BRig_RT_dataMTrig_Solenoid_Tdelay__R.vi"() -> ("output_Solenoid_Tdelay__R"=w141:i32)  [unwired: 11 in]
              n42 = local read "MTrig_Solenoid_Tcycle__L"() -> (w153:u16)
              n43 = local read "MTrig_Solenoid_Tcycle__R"() -> (w154:u16)
              n44 = local read "MTrig_Laser_Tcycle"() -> (w137:u16)
              n45 = call "myRIO_BRig_RT_dataMTrig_init.vi"() -> ("output_dataMTrig"=w147:u16[])  [unwired: 5 in]
              n46 = local write "RewCalib_Trig_R"(w140) -> ()
              n47 = local write "RewCalib_Trig_L"(w140) -> ()
              n48 = local read "Tcycle_Cue_min"() -> (w138:u16)
              n49 = Replace Array Subset(array=w147, new element #1=w153, index #1=w148, new element #2=w154, index #2=w149, new element #3=w138, index #3=w150, new element #4=w138, index #4=w151, new element #5=w137, index #5=w152, new element #6=w136, index #6=w144, new element #7=w136, index #7=w143, new element #8=w136, index #8=w142, new element #9=w136, index #9=w141) -> (w146:u16[])
            }
            frame "UploadSettings_pre" {
              # "When the Host sends settings,\nnot all files send at the same time.\n\nIf RT reads the settings faster\nthan the Host can send them,\nthen we will skip settings.\n\nSolution:\nWait 20 cycles"
              n50 = Increment(x=w163) -> (x+1=w162:u16)
              n51 = Greater?(x=w162, y=u16 20) -> (0:w160:bool)
              n52 = Select(t=myRIO_BRig_RT__Case_NonExp_stateList."UploadSettings_Read_dataExp", s=w160, f=w159) -> (s? t:f=w157:T1)
            }
            frame "UploadSettings_Read_dataExp" {
              # "grab dataExp and\nstore it in the\ngeneric data array"
              # "dataExp"
              n53 = call "myRIO_BRig_RT_dataExp_init_details.vi"() -> ("output_dataSize"=w170:i32, "output_dataName"=w173:string)  [unwired: 10 in]
              n54 = call "myRIO_BRig_RT_comm_webdav_uploadReceived_check.vi"("input_dataName"=w173) -> ("output_Iexist"=w172:bool, "output_dataPath"=w171:path)  [unwired: 9 in]
              n55 = case shown="True" w172 {
                tunnel: w171 -> [_ w182]
                tunnel: w170 -> [_ w181]
                tunnel: [_ w180] -> w169
                tunnel: w166 -> [w175 w179]
                tunnel: [w175 w176] -> w165
                frame False {
                }
                frame True {
                  n56 = call "myRIO_BRig_RT_comm_webdav_uploadReceived_read.vi"("input_dataSize"=w181, "input_filePath"=w182) -> ("output_Ivalid"=w180:bool, "output_data"=w178:i64[])  [unwired: 8 in]
                  n57 = To Unsigned Word Integer(number=w178) -> (unsigned 16bit integer=w177:u16[])
                  n58 = Select(t=w177, s=w180, f=w179) -> (s? t:f=w176:u16[])
                }
              }
              n59 = Select(t=myRIO_BRig_RT__Case_NonExp_stateList."UploadSettings_dataExp_1", s=w169, f=myRIO_BRig_RT__Case_NonExp_stateList."UploadSettings_Read_dataLC" ("t")) -> (s? t:f=w164:T1)
            }
            frame "UploadSettings_Read_dataLC" {
              # "grab dataLC and\nstore it in the\ngeneric data array"
              # "dataLC"
              n60 = call "myRIO_BRig_RT_dataLC_init_details.vi"() -> ("output_dataSize"=w189:i32, "output_dataName"=w192:string)  [unwired: 10 in]
              n61 = call "myRIO_BRig_RT_comm_webdav_uploadReceived_check.vi"("input_dataName"=w192) -> ("output_Iexist"=w191:bool, "output_dataPath"=w190:path)  [unwired: 9 in]
              n62 = case shown="True" w191 {
                tunnel: w190 -> [_ w201]
                tunnel: w189 -> [_ w200]
                tunnel: [_ w199] -> w188
                tunnel: w185 -> [w194 w198]
                tunnel: [w194 w195] -> w184
                frame False {
                }
                frame True {
                  n63 = call "myRIO_BRig_RT_comm_webdav_uploadReceived_read.vi"("input_dataSize"=w200, "input_filePath"=w201) -> ("output_Ivalid"=w199:bool, "output_data"=w197:i64[])  [unwired: 8 in]
                  n64 = To Unsigned Word Integer(number=w197) -> (unsigned 16bit integer=w196:u16[])
                  n65 = Select(t=w196, s=w199, f=w198) -> (s? t:f=w195:u16[])
                }
              }
              n66 = Select(t=myRIO_BRig_RT__Case_NonExp_stateList."UploadSettings_dataLC_1", s=w188, f=myRIO_BRig_RT__Case_NonExp_stateList."UploadSettings_Read_dataMTrig" ("t")) -> (s? t:f=w183:T1)
            }
            frame "UploadSettings_Read_dataMTrig" {
              # "grab dataMTrig and\nstore it in the\ngeneric data array"
              # "dataMTrig"
              n67 = call "myRIO_BRig_RT_dataMTrig_init_details.vi"() -> ("output_dataSize"=w208:i32, "output_dataName"=w211:string)  [unwired: 10 in]
              n68 = call "myRIO_BRig_RT_comm_webdav_uploadReceived_check.vi"("input_dataName"=w211) -> ("output_Iexist"=w210:bool, "output_dataPath"=w209:path)  [unwired: 9 in]
              n69 = case shown="True" w210 {
                tunnel: w209 -> [_ w220]
                tunnel: w208 -> [_ w219]
                tunnel: [_ w218] -> w207
                tunnel: w204 -> [w213 w217]
                tunnel: [w213 w214] -> w203
                frame False {
                }
                frame True {
                  n70 = call "myRIO_BRig_RT_comm_webdav_uploadReceived_read.vi"("input_dataSize"=w219, "input_filePath"=w220) -> ("output_Ivalid"=w218:bool, "output_data"=w216:i64[])  [unwired: 8 in]
                  n71 = To Unsigned Word Integer(number=w216) -> (unsigned 16bit integer=w215:u16[])
                  n72 = Select(t=w215, s=w218, f=w217) -> (s? t:f=w214:u16[])
                }
              }
              n73 = Select(t=myRIO_BRig_RT__Case_NonExp_stateList."UploadSettings_dataMTrig_1", s=w207, f=myRIO_BRig_RT__Case_NonExp_stateList."Idle" ("t")) -> (s? t:f=w202:T1)
            }
            frame "UploadSettings_dataExp_1" {
              w229 = 100.0 ("y")
              # "Freq"
              # "f_millisec2count"
              # "laser"
              # "Cue_max"
              # "Cue_min"
              # "CuePenalty"
              # "Timeout"
              # "Wrong"
              # "Selection"
              # "RewardPost"
              # "Reward_R"
              # "Reward_L"
              # "Tcycle"
              # "TPB_min_R"
              # "TPB_min_L"
              # "TPB_max_R"
              # "TPB_max_L"
              # "I_trialUntilReward"
              # "ENL_penalty"
              # "ENL_min"
              # "ENL_max"
              # "BUR_max"
              # "BUR_min"
              # "CueCycles"
              # "Audio_Freq_R"
              # "Audio_Freq_L"
              # "Audio_Amp_R"
              # "Audio_Amp_L"
              n74 = call "myRIO_BRig_RT_dataExp_laser_f_millisec2count.vi"() -> ("output_laser_f_millisec2count"=w243:i32)  [unwired: 11 in]
              n75 = call "myRIO_BRig_RT_dataExp_laser_Freq.vi"() -> ("output_laser_Freq"=w242:i32)  [unwired: 11 in]
              n76 = call "myRIO_BRig_RT_dataExp_CueCycles.vi"() -> ("output_CueCycles"=w289:i32)  [unwired: 11 in]
              n77 = call "myRIO_BRig_RT_dataExp_Audio_amp__R.vi"() -> ("output_Audio_amp__R"=w293:i32)  [unwired: 11 in]
              n78 = call "myRIO_BRig_RT_dataExp_Audio_amp__L.vi"() -> ("output_Audio_amp__L"=w295:i32)  [unwired: 11 in]
              n79 = call "myRIO_BRig_RT_dataExp_Tcycle_Reward__L.vi"() -> ("output_Tcycle_Reward__L"=w266:i32)  [unwired: 11 in]
              n80 = call "myRIO_BRig_RT_dataExp_Tcycle_Reward__R.vi"() -> ("output_Tcycle_Reward__R"=w265:i32)  [unwired: 11 in]
              n81 = call "myRIO_BRig_RT_dataExp_Tcycle_RewardPost.vi"() -> ("output_Tcycle_RewardPost"=w264:i32)  [unwired: 11 in]
              n82 = call "myRIO_BRig_RT_dataExp_BUR_min.vi"() -> ("output_BUR_min"=w286:i32)  [unwired: 11 in]
              n83 = call "myRIO_BRig_RT_dataExp_ENL_min.vi"() -> ("output_ENL_min"=w282:i32)  [unwired: 11 in]
              n84 = call "myRIO_BRig_RT_dataExp_TPB_max__L.vi"() -> ("output_TPB_max__L"=w274:i32)  [unwired: 11 in]
              n85 = call "myRIO_BRig_RT_dataExp_TPB_max__R.vi"() -> ("output_TPB_max__R"=w273:i32)  [unwired: 11 in]
              n86 = call "myRIO_BRig_RT_dataExp_ENL_penalty.vi"() -> ("output_ENL_penalty"=w281:i32)  [unwired: 11 in]
              n87 = call "myRIO_BRig_RT_dataExp_laser_Power_min.vi"() -> ("output_laser_Power_min"=w241:i32)  [unwired: 11 in]
              n88 = call "myRIO_BRig_RT_dataExp_laser_Tpeak.vi"() -> ("output_laser_Tpeak"=w240:i32)  [unwired: 11 in]
              n89 = call "myRIO_BRig_RT_dataExp_Audio_freq__L.vi"() -> ("output_Audio_freq__L"=w291:i32)  [unwired: 11 in]
              n90 = call "myRIO_BRig_RT_dataExp_Audio_freq__R.vi"() -> ("output_Audio_freq__R"=w290:i32)  [unwired: 11 in]
              n91 = call "myRIO_BRig_RT_dataExp_BUR_max.vi"() -> ("output_BUR_max"=w287:i32)  [unwired: 11 in]
              n92 = call "myRIO_BRig_RT_dataExp_ENL_max.vi"() -> ("output_ENL_max"=w283:i32)  [unwired: 11 in]
              n93 = call "myRIO_BRig_RT_dataExp_ItrialUntilReward.vi"() -> ("output_I_trialUntilReward"=w277:i32)  [unwired: 11 in]
              n94 = call "myRIO_BRig_RT_dataExp_Tcycle_Selection.vi"() -> ("output_Tcycle_Selection"=w263:i32)  [unwired: 11 in]
              n95 = call "myRIO_BRig_RT_dataExp_Tcycle_Wrong.vi"() -> ("output_Tcycle_Wrong"=w262:i32)  [unwired: 11 in]
              n96 = call "myRIO_BRig_RT_dataExp_Tcycle_Timeout.vi"() -> ("output_Tcycle_Timeout"=w261:i32)  [unwired: 11 in]
              n97 = call "myRIO_BRig_RT_dataExp_TPB_min__L.vi"() -> ("output_TPB_min__L"=w272:i32)  [unwired: 11 in]
              n98 = call "myRIO_BRig_RT_dataExp_TPB_min__R.vi"() -> ("output_TPB_min__R"=w271:i32)  [unwired: 11 in]
              n99 = call "myRIO_BRig_RT_dataExp_laser_Tshutter.vi"() -> ("output_laser_Tshutter"=w239:i32)  [unwired: 11 in]
              n100 = call "myRIO_BRig_RT_dataExp_laser_duration.vi"() -> ("output_laser_duration"=w238:i32)  [unwired: 11 in]
              n101 = call "myRIO_BRig_RT_dataExp_Tcycle_CuePenalty.vi"() -> ("output_Tcycle_CuePenalty"=w254:i32)  [unwired: 11 in]
              n102 = call "myRIO_BRig_RT_dataExp_Tcycle_Cue_min.vi"() -> ("output_Tcycle_Cue_min"=w253:i32)  [unwired: 11 in]
              n103 = call "myRIO_BRig_RT_dataExp_Tcycle_Cue_max.vi"() -> ("output_Tcycle_Cue_max"=w252:i32)  [unwired: 11 in]
              n104 = Index Array(array=w246, index #1=w295, index #2=w293, index #3=w291, index #4=w290, index #5=w289, index #6=w287, index #7=w286, index #8=w283, index #9=w282, index #10=w281, index #11=w277, index #12=w274, index #13=w273, index #14=w272, index #15=w271, index #16=w266, index #17=w265, index #18=w264, index #19=w263, index #20=w262, index #21=w261, index #22=w254, index #23=w253, index #24=w252, index #25=w243, index #26=w242, index #27=w241, index #28=w240, index #29=w239, index #30=w238) -> (element #1=w294:u16, element #2=w292:u16, element #3=w249:u16, element #4=w248:u16, element #5=w288:u16, element #6=w285:u16, element #7=w284:u16, element #8=w280:u16, element #9=w279:u16, element #10=w278:u16, element #11=w275:u16, element #12=w270:u16, element #13=w269:u16, element #14=w268:u16, element #15=w267:u16, element #16=w260:u16, element #17=w259:u16, element #18=w258:u16, element #19=w257:u16, element #20=w256:u16, element #21=w255:u16, element #22=w251:u16, element #23=w245:u16, element #24=w244:u16, element #25=w237:u16, element #26=w228:u16, element #27=w227:u16, element #28=w226:u16, element #29=w225:u16, element #30=w221:u16)
              n105 = To Double Precision Float(number=w237) -> (double precision float=w236:dbl)
              n106 = To Double Precision Float(number=w228) -> (double precision float=w234:dbl)
              n107 = To Double Precision Float(number=w227) -> (double precision float=w232:dbl)
              n108 = To Double Precision Float(number=w226) -> (double precision float=w231:dbl)
              n109 = To Double Precision Float(number=w225) -> (double precision float=w230:dbl)
              n110 = local write "Tcycle_Selection"(w257) -> ()
              n111 = local write "Tcycle_Wrong"(w256) -> ()
              n112 = local write "Tcycle_Timeout"(w255) -> ()
              n113 = local write "Audio_Amp__L"(w294) -> ()
              n114 = local write "Audio_Amp__R"(w292) -> ()
              n115 = Divide(x=w236, y=w229) -> (x/y=w235:dbl)
              n116 = Divide(x=w234, y=w229) -> (x/y=w233:dbl)
              n117 = Divide(x=w232, y=w229) -> (x/y=w224:dbl)
              n118 = Divide(x=w231, y=w229) -> (x/y=w223:dbl)
              n119 = Divide(x=w230, y=w229) -> (x/y=w222:dbl)
              n120 = local write "Tcycle_ENLPenalty"(w278) -> ()
              n121 = local write "Tcycle_ENL_max"(w280) -> ()
              n122 = local write "laser_duration"(w221) -> ()
              n123 = local write "TpB_Min_L"(w268) -> ()
              n124 = local write "TpB_Min_R"(w267) -> ()
              n125 = local write "laser_power_min"(w224) -> ()
              n126 = local write "f_millisec2count"(w235) -> ()
              n127 = local write "laser_Tshutter"(w222) -> ()
              n128 = local write "laser_Tpeak"(w223) -> ()
              n129 = local write "laser_Freq"(w233) -> ()
              n130 = local write "Tcycle_CuePenalty"(w251) -> ()
              n131 = local write "Tcycle_Cue_min"(w245) -> ()
              n132 = local write "Tcycle_Cue_max"(w244) -> ()
              n133 = To Unsigned Byte Integer(number=w249) -> (unsigned 8bit integer=w250:u8)
              n134 = To Unsigned Byte Integer(number=w248) -> (unsigned 8bit integer=w247:u8)
              n135 = Not Equal To 0?(x=w275) -> (x != 0?=w276:bool)
              n136 = local write "Tcycle_Reward_L"(w260) -> ()
              n137 = local write "Tcycle_Reward_R"(w259) -> ()
              n138 = local write "Tcycle_RewardPost"(w258) -> ()
              n139 = local write "CueCycles"(w288) -> ()
              n140 = local write "BUR_min"(w284) -> ()
              n141 = local write "BUR_max"(w285) -> ()
              n142 = local write "Tcycle_ENL_min"(w279) -> ()
              n143 = local write "TpB_Max_L"(w270) -> ()
              n144 = local write "TpB_Max_R"(w269) -> ()
              n145 = local write "TrialUntilReward"(w276) -> ()
              n146 = local write "Audio_Freq__L"(w250) -> ()
              n147 = local write "Audio_Freq__R"(w247) -> ()
            }
            frame "UploadSettings_dataLC_1" {
              # "Cue1_All_delayOpt"
              # "ENL1_All_delayOpt"
              # "Cue1_First_delayOpt"
              # "ENL1_First_delayOpt"
              # "ENL1 First"
              # "Cue1 All"
              # "Cue1 First"
              # "Count"
              # "Tdelay"
              # "Prob"
              # "OnOff"
              # "Block"
              # "ENL1 All"
              # "Count"
              # "Tdelay"
              # "Prob"
              # "OnOff"
              # "Block"
              # "Count"
              # "Tdelay"
              # "Prob"
              # "Block"
              # "OnOff"
              # "Count"
              # "Tdelay"
              # "Prob"
              # "OnOff"
              # "Block"
              n148 = call "myRIO_BRig_RT_dataLC_Cue1_First_Block.vi"() -> ("output_Cue1_First_Block"=w354:i32)  [unwired: 11 in]
              n149 = call "myRIO_BRig_RT_dataLC_Cue1_First_OnOff.vi"() -> ("output_Cue1_First_OnOff"=w352:i32)  [unwired: 11 in]
              n150 = call "myRIO_BRig_RT_dataLC_Cue1_First_Count.vi"() -> ("output_Cue1_First_Count"=w349:i32)  [unwired: 11 in]
              n151 = call "myRIO_BRig_RT_dataLC_Cue1_All_Block.vi"() -> ("output_Cue1_All_Block"=w336:i32)  [unwired: 11 in]
              n152 = call "myRIO_BRig_RT_dataLC_Cue1_All_OnOff.vi"() -> ("output_Cue1_All_OnOff"=w335:i32)  [unwired: 11 in]
              n153 = call "myRIO_BRig_RT_dataLC_Cue1_All_Count.vi"() -> ("output_Cue1_All_Count"=w346:i32)  [unwired: 11 in]
              n154 = call "myRIO_BRig_RT_dataLC_ENL1_First_Block.vi"() -> ("output_ENL1_First_Block"=w334:i32)  [unwired: 11 in]
              n155 = call "myRIO_BRig_RT_dataLC_ENL1_First_OnOff.vi"() -> ("output_ENL1_First_OnOff"=w345:i32)  [unwired: 11 in]
              n156 = call "myRIO_BRig_RT_dataLC_ENL1_First_Count.vi"() -> ("output_ENL1_First_Count"=w342:i32)  [unwired: 11 in]
              n157 = call "myRIO_BRig_RT_dataLC_ENL1_All_Block.vi"() -> ("output_ENL1_All_Block"=w341:i32)  [unwired: 11 in]
              n158 = call "myRIO_BRig_RT_dataLC_ENL1_All_OnOff.vi"() -> ("output_ENL1_All_OnOff"=w340:i32)  [unwired: 11 in]
              n159 = call "myRIO_BRig_RT_dataLC_ENL1_All_Count.vi"() -> ("output_ENL1_All_Count"=w337:i32)  [unwired: 11 in]
              n160 = call "myRIO_BRig_RT_dataLC_ENL1_First_delayOpt.vi"() -> ("output_ENL1_First_delayOpt"=w311:i32)  [unwired: 11 in]
              n161 = call "myRIO_BRig_RT_dataLC_Cue1_First_delayOpt.vi"() -> ("output_Cue1_First_delayOpt"=w310:i32)  [unwired: 11 in]
              n162 = call "myRIO_BRig_RT_dataLC_ENL1_All_delayOpt.vi"() -> ("output_ENL1_All_delayOpt"=w303:i32)  [unwired: 11 in]
              n163 = call "myRIO_BRig_RT_dataLC_Cue1_All_delayOpt.vi"() -> ("output_Cue1_All_delayOpt"=w302:i32)  [unwired: 11 in]
              n164 = call "myRIO_BRig_RT_dataLC_Cue1_First_Probability.vi"() -> ("output_Cue1_First_Probability"=w351:i32)  [unwired: 11 in]
              n165 = call "myRIO_BRig_RT_dataLC_Cue1_First_Tdelay.vi"() -> ("output_Cue1_First_Tdelay"=w350:i32)  [unwired: 11 in]
              n166 = call "myRIO_BRig_RT_dataLC_Cue1_All_Probability.vi"() -> ("output_Cue1_All_Probability"=w348:i32)  [unwired: 11 in]
              n167 = call "myRIO_BRig_RT_dataLC_Cue1_All_Tdelay.vi"() -> ("output_Cue1_All_Tdelay"=w347:i32)  [unwired: 11 in]
              n168 = call "myRIO_BRig_RT_dataLC_ENL1_First_Probability.vi"() -> ("output_ENL1_First_Probability"=w344:i32)  [unwired: 11 in]
              n169 = call "myRIO_BRig_RT_dataLC_ENL1_First_Tdelay.vi"() -> ("output_ENL1_First_Tdelay"=w343:i32)  [unwired: 11 in]
              n170 = call "myRIO_BRig_RT_dataLC_ENL1_All_Probability.vi"() -> ("output_ENL1_All_Probability"=w339:i32)  [unwired: 11 in]
              n171 = call "myRIO_BRig_RT_dataLC_ENL1_All_Tdelay.vi"() -> ("output_ENL1_All_Tdelay"=w338:i32)  [unwired: 11 in]
              n172 = Index Array(array=w312, index #1=w354, index #2=w352, index #3=w351, index #4=w350, index #5=w349, index #6=w336, index #7=w335, index #8=w348, index #9=w347, index #10=w346, index #11=w334, index #12=w345, index #13=w344, index #14=w343, index #15=w342, index #16=w341, index #17=w340, index #18=w339, index #19=w338, index #20=w337, index #21=w311, index #22=w310, index #23=w303, index #24=w302) -> (element #1=w353:u16, element #2=w332:u16, element #3=w331:u16, element #4=w330:u16, element #5=w329:u16, element #6=w325:u16, element #7=w324:u16, element #8=w323:u16, element #9=w322:u16, element #10=w321:u16, element #11=w320:u16, element #12=w319:u16, element #13=w318:u16, element #14=w317:u16, element #15=w304:u16, element #16=w316:u16, element #17=w315:u16, element #18=w314:u16, element #19=w313:u16, element #20=w305:u16, element #21=w308:u16, element #22=w306:u16, element #23=w299:u16, element #24=w298:u16)
              n173 = Not Equal To 0?(x=w299) -> (x != 0?=w301:bool)
              n174 = Not Equal To 0?(x=w298) -> (x != 0?=w300:bool)
              n175 = Not Equal To 0?(x=w308) -> (x != 0?=w309:bool)
              n176 = Not Equal To 0?(x=w306) -> (x != 0?=w307:bool)
              n177 = Not Equal To 0?(x=w332) -> (x != 0?=w333:bool)
              n178 = Not Equal To 0?(x=w324) -> (x != 0?=w328:bool)
              n179 = Not Equal To 0?(x=w319) -> (x != 0?=w327:bool)
              n180 = Not Equal To 0?(x=w315) -> (x != 0?=w326:bool)
              n181 = local write "LC_Cue1_First_Probability"(w331) -> ()
              n182 = local write "LC_ENL1_First_Probability"(w318) -> ()
              n183 = local write "LC_ENL1_First_delayOpt"(w309) -> ()
              n184 = local write "LC_Cue1_First_delayOpt"(w307) -> ()
              n185 = local write "LC_ENL1_All_delayOpt"(w301) -> ()
              n186 = local write "LC_Cue1_All_delayOpt"(w300) -> ()
              n187 = local write "LC_Cue1_All_Probability"(w323) -> ()
              n188 = local write "LC_Cue1_First_Tdelay"(w330) -> ()
              n189 = local write "LC_ENL1_All_Probability"(w314) -> ()
              n190 = local write "LC_Cue1_First_OnOff"(w333) -> ()
              n191 = local write "LC_Cue1_First_Count"(w329) -> ()
              n192 = local write "LC_Cue1_First_Block"(w353) -> ()
              n193 = local write "LC_ENL1_First_Tdelay"(w317) -> ()
              n194 = local write "LC_ENL1_First_OnOff"(w327) -> ()
              n195 = local write "LC_ENL1_First_Count"(w304) -> ()
              n196 = local write "LC_ENL1_First_Block"(w320) -> ()
              n197 = local write "LC_Cue1_All_Tdelay"(w322) -> ()
              n198 = local write "LC_Cue1_All_OnOff"(w328) -> ()
              n199 = local write "LC_Cue1_All_Count"(w321) -> ()
              n200 = local write "LC_Cue1_All_Block"(w325) -> ()
              n201 = local write "LC_ENL1_All_Tdelay"(w313) -> ()
              n202 = local write "LC_ENL1_All_OnOff"(w326) -> ()
              n203 = local write "LC_ENL1_All_Count"(w305) -> ()
              n204 = local write "LC_ENL1_All_Block"(w316) -> ()
            }
            frame "UploadSettings_dataLC_2" {
              # "Wrong"
              # "Reward"
              # "Trial"
              # "Tdelay"
              # "Prob"
              # "Block"
              # "OnOff"
              # "Trial"
              # "Tdelay"
              # "Prob"
              # "OnOff"
              # "Block"
              n205 = call "myRIO_BRig_RT_dataLC_Reward_Block.vi"() -> ("output_Reward_Block"=w379:i32)  [unwired: 11 in]
              n206 = call "myRIO_BRig_RT_dataLC_Reward_OnOff.vi"() -> ("output_Reward_OnOff"=w377:i32)  [unwired: 11 in]
              n207 = call "myRIO_BRig_RT_dataLC_Reward_Trial.vi"() -> ("output_Reward_Trial"=w374:i32)  [unwired: 11 in]
              n208 = call "myRIO_BRig_RT_dataLC_Wrong_Block.vi"() -> ("output_Wrong_Block"=w370:i32)  [unwired: 11 in]
              n209 = call "myRIO_BRig_RT_dataLC_Wrong_OnOff.vi"() -> ("output_Wrong_OnOff"=w369:i32)  [unwired: 11 in]
              n210 = call "myRIO_BRig_RT_dataLC_Wrong_Trial.vi"() -> ("output_Wrong_Trial"=w371:i32)  [unwired: 11 in]
              n211 = call "myRIO_BRig_RT_dataLC_Reward_Probability.vi"() -> ("output_Reward_Probability"=w376:i32)  [unwired: 11 in]
              n212 = call "myRIO_BRig_RT_dataLC_Reward_Tdelay.vi"() -> ("output_Reward_Tdelay"=w375:i32)  [unwired: 11 in]
              n213 = call "myRIO_BRig_RT_dataLC_Wrong_Probability.vi"() -> ("output_Wrong_Probability"=w373:i32)  [unwired: 11 in]
              n214 = call "myRIO_BRig_RT_dataLC_Wrong_Tdelay.vi"() -> ("output_Wrong_Tdelay"=w372:i32)  [unwired: 11 in]
              n215 = Index Array(array=w357, index #1=w379, index #2=w377, index #3=w376, index #4=w375, index #5=w374, index #6=w370, index #7=w369, index #8=w373, index #9=w372, index #10=w371) -> (element #1=w378:u16, element #2=w367:u16, element #3=w366:u16, element #4=w365:u16, element #5=w364:u16, element #6=w362:u16, element #7=w361:u16, element #8=w360:u16, element #9=w359:u16, element #10=w358:u16)
              n216 = Not Equal To 0?(x=w367) -> (x != 0?=w368:bool)
              n217 = Not Equal To 0?(x=w361) -> (x != 0?=w363:bool)
              n218 = local write "LC_Reward_Probability"(w366) -> ()
              n219 = local write "LC_Wrong_Probability"(w360) -> ()
              n220 = local write "LC_Reward_Tdelay"(w365) -> ()
              n221 = local write "LC_Reward_OnOff"(w368) -> ()
              n222 = local write "LC_Reward_Block"(w378) -> ()
              n223 = local write "LC_Reward_Trial"(w364) -> ()
              n224 = local write "LC_Wrong_Tdelay"(w359) -> ()
              n225 = local write "LC_Wrong_OnOff"(w363) -> ()
              n226 = local write "LC_Wrong_Block"(w362) -> ()
              n227 = local write "LC_Wrong_Trial"(w358) -> ()
            }
            frame "UploadSettings_dataMTrig_1" {
              # "Tdelay_R"
              # "Tdelay_L"
              # "Tcycle_R"
              # "Tcycle_L"
              # "RewCalib_nCycle_R"
              # "RewCalib_nCycle_L"
              # "Solenoid"
              # "Laser_Tcycle"
              n228 = call "myRIO_BRig_RT_dataMTrig_Laser_Tcycle.vi"() -> ("output_Laser_Tcycle"=w389:i32)  [unwired: 11 in]
              n229 = call "myRIO_BRig_RT_dataMTrig_Solenoid_RewCalib_nCycle__L.vi"() -> ("output_Solenoid_RewCalib_nCycle__L"=w388:i32)  [unwired: 11 in]
              n230 = call "myRIO_BRig_RT_dataMTrig_Solenoid_RewCalib_nCycle__R.vi"() -> ("output_Solenoid_RewCalib_nCycle__R"=w387:i32)  [unwired: 11 in]
              n231 = call "myRIO_BRig_RT_dataMTrig_Solenoid_Tdelay__L.vi"() -> ("output_Solenoid_Tdelay__L"=w384:i32)  [unwired: 11 in]
              n232 = call "myRIO_BRig_RT_dataMTrig_Solenoid_Tdelay__R.vi"() -> ("output_Solenoid_Tdelay__R"=w383:i32)  [unwired: 11 in]
              n233 = call "myRIO_BRig_RT_dataMTrig_Solenoid_Tcycle__L.vi"() -> ("output_Solenoid_Tcycle__L"=w386:i32)  [unwired: 11 in]
              n234 = call "myRIO_BRig_RT_dataMTrig_Solenoid_Tcycle__R.vi"() -> ("output_Solenoid_Tcycle__R"=w385:i32)  [unwired: 11 in]
              n235 = Index Array(array=w382, index #1=w389, index #2=w388, index #3=w387, index #4=w386, index #5=w385, index #6=w384, index #7=w383) -> (element #1=w396:u16, element #2=w395:u16, element #3=w394:u16, element #4=w393:u16, element #5=w392:u16, element #6=w391:u16, element #7=w390:u16)
              n236 = Replace Array Subset(array=w398, new element #1=w396, index #1=w389, new element #2=w395, index #2=w388, new element #3=w394, index #3=w387, new element #4=w393, index #4=w386, new element #5=w392, index #5=w385, new element #6=w391, index #6=w384, new element #7=w390, index #7=w383) -> (w397:u16[])
              n237 = local write "MTrig_Solenoid_Tcycle__L"(w393) -> ()
              n238 = local write "MTrig_Solenoid_Tcycle__R"(w392) -> ()
              n239 = local write "MTrig_Laser_Tcycle"(w396) -> ()
            }
            frame "Idle" {
              # "To ensure timing, we split the\nidle state into 4 phases"
              # "Laser_Tcycle"
              # "Audio_Tcycle_R"
              # "Audio_Tcycle_L"
              n240 = local read "laser_power_min"() -> (w401:dbl)
              n241 = local read "f_millisec2count"() -> (w409:dbl)
              n242 = local read "Audio_Amp__R"() -> (w403:u16)
              n243 = local read "Audio_Amp__L"() -> (w405:u16)
              n244 = local read "Audio_Freq__R"() -> (w402:u8)
              n245 = local read "Audio_Freq__L"() -> (w404:u8)
              n246 = local read "MTrig_Audio_trig__L"() -> (w417:bool)
              n247 = local read "MTrig_Audio_trig__R"() -> (w419:bool)
              n248 = Select(t=myRIO_BRig_RT__Case_NonExp_stateList."SendData" ("Enum"), s="SendData", f=myRIO_BRig_RT__Case_NonExp_stateList."Idle_2" ("Enum")) -> (s? t:f=w412:T1)
              n249 = call "myRIO__convert__Voltage_to_FPGAvalue.vi"("input_voltage"=w401) -> ("output_PortC"=w400:i16)  [unwired: 9 in, 1 out]
              n250 = local read "MTrig_Laser_trig"() -> (w418:bool)
              n251 = To Unsigned Word Integer(number=w409) -> (unsigned 16bit integer=w408:u16)
              n252 = call "myRIO_BRig_RT_dataMTrig_Audio_Tcycle__L.vi"() -> ("output_Audio_Tcycle__L"=w428:i32)  [unwired: 11 in]
              n253 = call "myRIO_BRig_RT_dataMTrig_Audio_Tcycle__R.vi"() -> ("output_Audio_Tcycle__R"=w427:i32)  [unwired: 11 in]
              n254 = call "myRIO_BRig_RT_dataMTrig_Laser_Tcycle.vi"() -> ("output_Laser_Tcycle"=w426:i32)  [unwired: 11 in]
              n255 = local read "MTrig_Laser_Tcycle"() -> (w410:u16)
              n256 = xnode "Read/Write Control"("FPGA VI Reference In"=w407, "error in"=w406, "k1__counter_per_ms"=w408, "audioAmp_L"=w405, "audioFreq_L_kHz"=w404, "audioAmp_R"=w403, "audioFreq_R_kHz"=w402, "AnaOut_0"=w400) -> ()  [unwired: 2 out]
              n257 = Select(t=myRIO_BRig_RT__Case_NonExp_stateList."TestConnection" ("Enum"), s="TestConnection", f=w412) -> (s? t:f=w421:T1)
              n258 = local read "Tcycle_Cue_min"() -> (w411:u16)
              n259 = Compound Arithmetic op=OR(w417, w419, w418) -> (w420:bool)
              n260 = case shown="True" w420 {
                frame False {
                }
                frame True {
                  w429 = FALSE
                  n261 = local write "MTrig_Audio_trig__L"(w429) -> ()
                  n262 = local write "MTrig_Audio_trig__R"(w429) -> ()
                  n263 = local write "MTrig_Laser_trig"(w429) -> ()
                }
              }
              n264 = Replace Array Subset(array=w424, new element #1=w411, index #1=w428, new element #2=w411, index #2=w427, new element #3=w410, index #3=w426) -> (w425:u16[])
            }
            frame "Idle_2" {
              w431 = u16 0 ("t")
              # "To ensure timing, we split the\nidle state into 4 phases"
              # "Ncycles"
              # "Ncycles"
              # "RewCalib"
              # "RewCalib"
              # "Solenoid R"
              # "Solenoid L"
              n265 = call "myRIO_BRig_RT_dataMTrig_Solenoid_RewCalib_OnOff__L.vi"() -> ("output_Solenoid_RewCalib_OnOff__L"=w462:i32)  [unwired: 11 in]
              n266 = call "myRIO_BRig_RT_dataMTrig_Solenoid_N__L.vi"() -> ("output_Solenoid_N__L"=w450:i32)  [unwired: 11 in]
              n267 = call "myRIO_BRig_RT_dataMTrig_Solenoid_RewCalib_OnOff__R.vi"() -> ("output_Solenoid_RewCalib_OnOff__R"=w447:i32)  [unwired: 11 in]
              n268 = call "myRIO_BRig_RT_dataMTrig_Solenoid_N__R.vi"() -> ("output_Solenoid_N__R"=w446:i32)  [unwired: 11 in]
              n269 = Index Array(array=w453, index #1=w462, index #2=w450, index #3=w447, index #4=w446) -> (element #1=w449:u16, element #2=w444:u16, element #3=w445:u16, element #4=w443:u16)
              n270 = local read "RewCalib_Trig_L"() -> (w442:bool)
              n271 = local read "RewCalib_Trig_R"() -> (w441:bool)
              n272 = Equal To 0?(x=w444) -> (x = 0?=w452:bool)
              n273 = Equal To 0?(x=w443) -> (x = 0?=w451:bool)
              n274 = Not Equal To 0?(x=w445) -> (x != 0?=w463:bool)
              n275 = Not Equal To 0?(x=w449) -> (x != 0?=w464:bool)
              n276 = And(x=w452, y=w451) -> (x .and. y?=w456:bool)
              n277 = Or(x=w442, y=w441) -> (x .or. y?=w457:bool)
              n278 = Not Exclusive Or(1:w464, 2:w442) -> (0:w459:bool)
              n279 = Not Exclusive Or(1:w463, 2:w441) -> (0:w461:bool)
              n280 = And(x=w457, y=w456) -> (x .and. y?=w439:bool)
              n281 = Not(x=w459) -> (.not. x?=w458:bool)
              n282 = Not(x=w461) -> (.not. x?=w460:bool)
              n283 = Or(x=w458, y=w460) -> (x .or. y?=w440:bool)
              n284 = Or(x=w439, y=w440) -> (x .or. y?=w455:bool)
              n285 = local read "count_warmup_R"() -> (w430:u16)
              n286 = local read "count_warmup_L"() -> (w435:u16)
              n287 = Select(t=myRIO_BRig_RT__Case_NonExp_stateList."RewardCalibration_pre" ("Enum"), s=w455, f=myRIO_BRig_RT__Case_NonExp_stateList."Idle_3" ("Enum")) -> (s? t:f=w438:T1)
              n288 = Select(t=w431, s="count_warmup_L_reset", f=w435) -> (s? t:f=→"count_warmup_L":u16)
              n289 = Select(t=w431, s="count_warmup_R_reset", f=w430) -> (s? t:f=→"count_warmup_R":u16)
            }
            frame "Idle_3" {
              w487 = u8 0 ("f")
              # "To ensure timing, we split the\nidle state into 4 phases"
              n290 = local read "MTrig_Solenoid_trig__L"() -> (w478:bool)
              n291 = local read "MTrig_Solenoid_trig__R"() -> (w488:bool)
              n292 = local read "warmupType"() -> (w470:u8)
              n293 = local read "warmup"() -> (w480:bool)
              n294 = Not Equal To 0?(x=w470) -> (x != 0?=w469:bool)
              n295 = Not(x=w469) -> (.not. x?=w481:bool)
              n296 = Select(t=u8 1, s=w478, f=w487) -> (s? t:f=w486:u8)
              n297 = Select(t=u8 2, s=w488, f=w487) -> (s? t:f=w485:u8)
              n298 = And(x=w480, y=w481) -> (x .and. y?=w479:bool)
              n299 = And(x=w480, y=w469) -> (x .and. y?=w474:bool)
              n300 = Add(x=w486, y=w485) -> (x+y=w484:u8)
              n301 = case shown="3" w484 {
                tunnel: w483 -> [w491 w495 w513 w531]
                tunnel: [w491 w494 w512 w530] -> w482
                tunnel: w479 -> [_ w493 w511 w529]
                tunnel: [_ TRUE TRUE TRUE] -> w476
                frame 0, Default {
                }
                frame 1 {
                  n302 = case shown="True" w493 {
                    tunnel: w495 -> [w504 w509]
                    tunnel: [w503 w508] -> w494
                    frame True {
                      # "Audio_L"
                      # "Solenoid_L"
                      n303 = call "myRIO_BRig_RT_dataMTrig_Solenoid_N__L.vi"() -> ("output_Solenoid_N__L"=w500:i32)  [unwired: 11 in]
                      n304 = call "myRIO_BRig_RT_dataMTrig_Audio_N__L.vi"() -> ("output_Audio_N__L"=w498:i32)  [unwired: 11 in]
                      n305 = Index Array(array=w504, index #1=w500, index #2=w498) -> (element #1=w502:u16, element #2=w501:u16)
                      n306 = Increment(x=w502) -> (x+1=w499:u16)
                      n307 = Increment(x=w501) -> (x+1=w497:u16)
                      n308 = Replace Array Subset(array=w504, new element #1=w499, index #1=w500, new element #2=w497, index #2=w498) -> (w503:u16[])
                    }
                    frame False {
                      # "Solenoid_L"
                      n309 = call "myRIO_BRig_RT_dataMTrig_Solenoid_N__L.vi"() -> ("output_Solenoid_N__L"=w506:i32)  [unwired: 11 in]
                      n310 = Index Array(array=w509, index=w506) -> (element=w507:u16)
                      n311 = Increment(x=w507) -> (x+1=w505:u16)
                      n312 = Replace Array Subset(array=w509, new element=w505, index=w506) -> (w508:u16[])
                    }
                  }
                  n313 = local write "MTrig_Solenoid_trig__L"(FALSE) -> ()
                }
                frame 2 {
                  n314 = case shown="True" w511 {
                    tunnel: w513 -> [w522 w527]
                    tunnel: [w521 w526] -> w512
                    frame True {
                      # "Audio_R"
                      # "Solenoid_R"
                      n315 = call "myRIO_BRig_RT_dataMTrig_Solenoid_N__R.vi"() -> ("output_Solenoid_N__R"=w518:i32)  [unwired: 11 in]
                      n316 = call "myRIO_BRig_RT_dataMTrig_Audio_N__R.vi"() -> ("output_Audio_N__R"=w517:i32)  [unwired: 11 in]
                      n317 = Index Array(array=w522, index #1=w518, index #2=w517) -> (element #1=w520:u16, element #2=w519:u16)
                      n318 = Increment(x=w519) -> (x+1=w515:u16)
                      n319 = Increment(x=w520) -> (x+1=w516:u16)
                      n320 = Replace Array Subset(array=w522, new element #1=w516, index #1=w518, new element #2=w515, index #2=w517) -> (w521:u16[])
                    }
                    frame False {
                      # "Solenoid_R"
                      n321 = call "myRIO_BRig_RT_dataMTrig_Solenoid_N__R.vi"() -> ("output_Solenoid_N__R"=w523:i32)  [unwired: 11 in]
                      n322 = Index Array(array=w527, index=w523) -> (element=w525:u16)
                      n323 = Increment(x=w525) -> (x+1=w524:u16)
                      n324 = Replace Array Subset(array=w527, new element=w524, index=w523) -> (w526:u16[])
                    }
                  }
                  n325 = local write "MTrig_Solenoid_trig__R"(FALSE) -> ()
                }
                frame 3 {
                  w532 = FALSE
                  n326 = case shown="True" w529 {
                    tunnel: w531 -> [w546 w554]
                    tunnel: [w545 w553] -> w530
                    frame True {
                      # "Audio_R"
                      # "Solenoid_R"
                      # "Audio_L"
                      # "Solenoid_L"
                      n327 = call "myRIO_BRig_RT_dataMTrig_Solenoid_N__L.vi"() -> ("output_Solenoid_N__L"=w540:i32)  [unwired: 11 in]
                      n328 = call "myRIO_BRig_RT_dataMTrig_Audio_N__L.vi"() -> ("output_Audio_N__L"=w538:i32)  [unwired: 11 in]
                      n329 = call "myRIO_BRig_RT_dataMTrig_Solenoid_N__R.vi"() -> ("output_Solenoid_N__R"=w536:i32)  [unwired: 11 in]
                      n330 = call "myRIO_BRig_RT_dataMTrig_Audio_N__R.vi"() -> ("output_Audio_N__R"=w535:i32)  [unwired: 11 in]
                      n331 = Index Array(array=w546, index #1=w540, index #2=w538, index #3=w536, index #4=w535) -> (element #1=w544:u16, element #2=w543:u16, element #3=w542:u16, element #4=w541:u16)
                      n332 = Increment(x=w541) -> (x+1=w533:u16)
                      n333 = Increment(x=w544) -> (x+1=w539:u16)
                      n334 = Increment(x=w543) -> (x+1=w537:u16)
                      n335 = Increment(x=w542) -> (x+1=w534:u16)
                      n336 = Replace Array Subset(array=w546, new element #1=w539, index #1=w540, new element #2=w537, index #2=w538, new element #3=w534, index #3=w536, new element #4=w533, index #4=w535) -> (w545:u16[])
                    }
                    frame False {
                      # "Solenoid_R"
                      # "Solenoid_L"
                      n337 = call "myRIO_BRig_RT_dataMTrig_Solenoid_N__L.vi"() -> ("output_Solenoid_N__L"=w550:i32)  [unwired: 11 in]
                      n338 = call "myRIO_BRig_RT_dataMTrig_Solenoid_N__R.vi"() -> ("output_Solenoid_N__R"=w547:i32)  [unwired: 11 in]
                      n339 = Index Array(array=w554, index #1=w550, index #2=w547) -> (element #1=w552:u16, element #2=w551:u16)
                      n340 = Increment(x=w552) -> (x+1=w549:u16)
                      n341 = Increment(x=w551) -> (x+1=w548:u16)
                      n342 = Replace Array Subset(array=w554, new element #1=w549, index #1=w550, new element #2=w548, index #2=w547) -> (w553:u16[])
                    }
                  }
                  n343 = local write "MTrig_Solenoid_trig__L"(w532) -> ()
                  n344 = local write "MTrig_Solenoid_trig__R"(w532) -> ()
                }
              }
              n345 = local read "get_countPerMS"() -> (w468:bool)
              n346 = Select(t=myRIO_BRig_RT__Case_NonExp_stateList."Get_FPGA_count_per_ms" ("Enum"), s=w468, f=myRIO_BRig_RT__Case_NonExp_stateList."Idle_4" ("Enum")) -> (s? t:f=w466:T1)
              n347 = Select(t=myRIO_BRig_RT__Case_NonExp_stateList."Cue_pre", s=w474, f=myRIO_BRig_RT__Case_NonExp_stateList."DispenseWater_pre" ("Enum")) -> (s? t:f=w472:T1)
              n348 = Select(t=w472, s=w476, f=w466) -> (s? t:f=w477:T1)
            }
            frame "Idle_4" {
              # "use dataMTrig as it is one of the last to transfer"
              # "To ensure timing, we split the\nidle state into 4 phases"
              n349 = call "myRIO_BRig_RT_comm_webdav_uploadReceived_check_v2,0.vi"("input_dataName"="dataMTrig") -> ("output_Iexist"=w560:bool)  [unwired: 9 in, 1 out]
              n350 = Select(t=myRIO_BRig_RT__Case_NonExp_stateList."UploadSettings_pre" ("Enum"), s=w560, f=myRIO_BRig_RT__Case_NonExp_stateList."Idle") -> (s? t:f=w558:T1)
            }
            frame "Cue_pre" {
              w570 = u16 1 ("t")
              w569 = u16 0 ("new element/subarray")
              w566 = u16 0 ("new element/subarray")
              # "Ncycle"
              # "count"
              # "Audio_R"
              # "Solenoid_R"
              # "Solenoid_L"
              # "Ncycle"
              # "count"
              # "Audio_L"
              n351 = call "myRIO_BRig_RT_dataMTrig_Solenoid_N__L.vi"() -> ("output_Solenoid_N__L"=w579:i32)  [unwired: 11 in]
              n352 = call "myRIO_BRig_RT_dataMTrig_Solenoid_N__R.vi"() -> ("output_Solenoid_N__R"=w578:i32)  [unwired: 11 in]
              n353 = Index Array(array=w575, index #1=w579, index #2=w578) -> (element #1=w577:u16, element #2=w576:u16)
              n354 = Not Equal To 0?(x=w576) -> (x != 0?=w562:bool)
              n355 = Not Equal To 0?(x=w577) -> (x != 0?=w563:bool)
              n356 = Select(t=w570, s=w563, f=w569) -> (s? t:f=w571:u16)
              n357 = Select(t=w570, s=w562, f=w569) -> (s? t:f=w565:u16)
              n358 = call "myRIO_BRig_RT_dataMTrig_Audio_c__L.vi"() -> ("output_Audio_c__L"=w573:i32)  [unwired: 11 in]
              n359 = call "myRIO_BRig_RT_dataMTrig_Audio_N__L.vi"() -> ("output_Audio_N__L"=w572:i32)  [unwired: 11 in]
              n360 = call "myRIO_BRig_RT_dataMTrig_Audio_c__R.vi"() -> ("output_Audio_c__R"=w568:i32)  [unwired: 11 in]
              n361 = call "myRIO_BRig_RT_dataMTrig_Audio_N__R.vi"() -> ("output_Audio_N__R"=w567:i32)  [unwired: 11 in]
              n362 = Replace Array Subset(array=w575, new element #1=w566, index #1=w573, new element #2=w571, index #2=w572, new element #3=w566, index #3=w568, new element #4=w565, index #4=w567) -> (w574:u16[])
            }
            frame "Cue" {
              # "lick did not occur or warmupType==1"
              # "lick occurred?"
              # "Ncycle"
              # "Audio_R"
              # "Ncycle"
              # "Audio_L"
              n363 = local read "warmupType"() -> (w589:u8)
              n364 = Greater?(x=w595, y=w594) -> (0:w598:bool)
              n365 = Greater?(x=w597, y=w596) -> (0:w593:bool)
              n366 = Or(x=w593, y=w598) -> (x .or. y?=w587:bool)
              n367 = Equal?(x=w589, y=u8 1) -> (x = y?=w583:bool)
              n368 = Not(x=w587) -> (.not. x?=w586:bool)
              n369 = call "myRIO_BRig_RT_dataMTrig_Audio_N__L.vi"() -> ("output_Audio_N__L"=w601:i32)  [unwired: 11 in]
              n370 = call "myRIO_BRig_RT_dataMTrig_Audio_N__R.vi"() -> ("output_Audio_N__R"=w600:i32)  [unwired: 11 in]
              n371 = Or(x=w586, y=w583) -> (x .or. y?=w584:bool)
              n372 = case shown="True" w584 {
                tunnel: w601 -> [w607 w625]
                tunnel: w600 -> [w606 w624]
                tunnel: w592 -> [w609 w619]
                tunnel: [w608 w619] -> w591
                tunnel: w590 -> [_ w617]
                tunnel: [myRIO_BRig_RT__Case_NonExp_stateList."Idle" ("t") w616] -> w585
                tunnel: w583 -> [_ w615]
                tunnel: w582 -> [_ w611]
                tunnel: w581 -> [_ w610]
                frame False {
                  w602 = u16 0 ("new element/subarray")
                  # "lick occurred and warmupType==2"
                  n373 = call "myRIO_BRig_RT_dataMTrig_Solenoid_N__R.vi"() -> ("output_Solenoid_N__R"=w603:i32)  [unwired: 11 in]
                  n374 = call "myRIO_BRig_RT_dataMTrig_Solenoid_N__L.vi"() -> ("output_Solenoid_N__L"=w604:i32)  [unwired: 11 in]
                  n375 = Replace Array Subset(array=w609, new element #1=w602, index #1=w607, new element #2=w602, index #2=w606, new element #3=w602, index #3=w604, new element #4=w602, index #4=w603) -> (w608:u16[])
                }
                frame True {
                  n376 = Not(x=w615) -> (.not. x?=w614:bool)
                  n377 = Index Array(array=w619, index #1=w625, index #2=w624) -> (element #1=w623:u16, element #2=w622:u16)
                  n378 = Equal To 0?(x=w623) -> (x = 0?=w621:bool)
                  n379 = Equal To 0?(x=w622) -> (x = 0?=w620:bool)
                  n380 = And(x=w621, y=w620) -> (x .and. y?=w613:bool)
                  n381 = And(x=w613, y=w614) -> (x .and. y?=w612:bool)
                  n382 = case shown="True" w612 {
                    tunnel: w611 -> [_ w633]
                    tunnel: w610 -> [_ w628]
                    frame False {
                    }
                    frame True {
                      n383 = local read "count_warmup_R"() -> (w626:u16)
                      n384 = local read "count_warmup_L"() -> (w631:u16)
                      n385 = Increment(x=w626) -> (x+1=w629:u16)
                      n386 = Increment(x=w631) -> (x+1=w632:u16)
                      n387 = Select(t=w629, s=w628, f=w626) -> (s? t:f=w627:u16)
                      n388 = Select(t=w632, s=w633, f=w631) -> (s? t:f=w630:u16)
                      n389 = local write "count_warmup_R"(w627) -> ()
                      n390 = local write "count_warmup_L"(w630) -> ()
                    }
                  }
                  n391 = Select(t=myRIO_BRig_RT__Case_NonExp_stateList."DispenseWater_pre", s=w613, f=w617) -> (s? t:f=w616:T1)
                }
              }
            }
            frame "RewardCalibration_pre" {
              (unwired) FALSE
              w635 = FALSE
              w646 = u8 0
              w662 = u8 0
              # "Are we starting a RewardCalibration?\nOr are we stopping a RewardCalibration?\nOr is a RewardCalibration over?"
              # "RewCalib\nOnOff"
              # "N"
              # "Solenoid R"
              # "RewCalib\nOnOff"
              # "N"
              # "Solenoid L"
              n392 = local read "RewCalib_Trig_L"() -> (w669:bool)
              n393 = local read "RewCalib_Trig_R"() -> (w638:bool)
              n394 = call "myRIO_BRig_RT_dataMTrig_Solenoid_N__R.vi"() -> ("output_Solenoid_N__R"=w640:i32)  [unwired: 11 in]
              n395 = call "myRIO_BRig_RT_dataMTrig_Solenoid_RewCalib_OnOff__R.vi"() -> ("output_Solenoid_RewCalib_OnOff__R"=w637:i32)  [unwired: 11 in]
              n396 = call "myRIO_BRig_RT_dataMTrig_Solenoid_N__L.vi"() -> ("output_Solenoid_N__L"=w655:i32)  [unwired: 11 in]
              n397 = call "myRIO_BRig_RT_dataMTrig_Solenoid_RewCalib_OnOff__L.vi"() -> ("output_Solenoid_RewCalib_OnOff__L"=w656:i32)  [unwired: 11 in]
              n398 = Index Array(array=w639, index #1=w640, index #2=w637) -> (element #1=w650:u16, element #2=w645:u16)
              n399 = Index Array(array=w639, index #1=w655, index #2=w656) -> (element #1=w666:u16, element #2=w661:u16)
              n400 = Equal To 0?(x=w650) -> (x = 0?=w651:bool)
              n401 = Not Equal To 0?(x=w645) -> (x != 0?=w648:bool)
              n402 = Equal To 0?(x=w666) -> (x = 0?=w667:bool)
              n403 = Not Equal To 0?(x=w661) -> (x != 0?=w664:bool)
              n404 = local write "MTrig_Solenoid_trig__L"(w635) -> ()
              n405 = local write "MTrig_Solenoid_trig__R"(w635) -> ()
              n406 = Select(t=u8 1, s=w638, f=w646) -> (s? t:f=w642:u8)
              n407 = Select(t=u8 1, s=w669, f=w662) -> (s? t:f=w658:u8)
              n408 = Select(t=u8 2, s=w651, f=w646) -> (s? t:f=w643:u8)
              n409 = Select(t=u8 4, s=w648, f=w646) -> (s? t:f=w644:u8)
              n410 = Select(t=u8 2, s=w667, f=w662) -> (s? t:f=w659:u8)
              n411 = Select(t=u8 4, s=w664, f=w662) -> (s? t:f=w660:u8)
              n412 = Compound Arithmetic op=ADD(w642, w643, w644) -> (w641:u8)
              n413 = Compound Arithmetic op=ADD(w658, w659, w660) -> (w657:u8)
              n414 = case shown="7" w657 {
                tunnel: w639 -> [w699 w704 w706 w711 w716 w718 w721 w726]
                tunnel: [w699 w705 w706 w712 w717 w718 w722 w727] -> w654
                tunnel: w656 -> [_ w702 _ w709 w714 _ w720 w725]
                tunnel: w655 -> [_ w703 _ w710 w715 _ _ _]
                frame 0, Default {
                }
                frame 1 {
                  n415 = Replace Array Subset(array=w704, new element #1=u16 100 ("new element/subarray"), index #1=w703, new element #2=u16 1 ("new element/subarray"), index #2=w702) -> (w705:u16[])
                }
                frame 2 {
                }
                frame 3 {
                  n416 = Replace Array Subset(array=w711, new element #1=u16 100 ("new element/subarray"), index #1=w710, new element #2=u16 1 ("new element/subarray"), index #2=w709) -> (w712:u16[])
                }
                frame 4 {
                  w713 = u16 0 ("new element/subarray")
                  n417 = Replace Array Subset(array=w716, new element #1=w713, index #1=w715, new element #2=w713, index #2=w714) -> (w717:u16[])
                }
                frame 5 {
                }
                frame 6 {
                  n418 = Replace Array Subset(array=w721, new element=u16 0 ("new element/subarray"), index=w720) -> (w722:u16[])
                }
                frame 7 {
                  n419 = local write "RewCalib_Trig_L"(FALSE ("RewCalib_Trig_L")) -> ()
                  n420 = Replace Array Subset(array=w726, new element=u16 0 ("new element/subarray"), index=w725) -> (w727:u16[])
                }
              }
              n421 = case shown="7" w641 {
                tunnel: w654 -> [w670 w675 w677 w682 w687 w689 w692 w697]
                tunnel: [w670 w676 w677 w683 w688 w689 w693 w698] -> w653
                tunnel: w637 -> [_ w673 _ w680 w685 _ w691 w696]
                tunnel: w640 -> [_ w674 _ w681 w686 _ _ _]
                frame 0, Default {
                }
                frame 1 {
                  n422 = Replace Array Subset(array=w675, new element #1=u16 100 ("new element/subarray"), index #1=w674, new element #2=u16 1 ("new element/subarray"), index #2=w673) -> (w676:u16[])
                }
                frame 2 {
                }
                frame 3 {
                  n423 = Replace Array Subset(array=w682, new element #1=u16 100 ("new element/subarray"), index #1=w681, new element #2=u16 1 ("new element/subarray"), index #2=w680) -> (w683:u16[])
                }
                frame 4 {
                  w684 = u16 0 ("new element/subarray")
                  n424 = Replace Array Subset(array=w687, new element #1=w684, index #1=w686, new element #2=w684, index #2=w685) -> (w688:u16[])
                }
                frame 5 {
                }
                frame 6 {
                  n425 = Replace Array Subset(array=w692, new element=u16 0 ("new element/subarray"), index=w691) -> (w693:u16[])
                }
                frame 7 {
                  n426 = local write "RewCalib_Trig_R"(FALSE ("RewCalib_Trig_L")) -> ()
                  n427 = Replace Array Subset(array=w697, new element=u16 0 ("new element/subarray"), index=w696) -> (w698:u16[])
                }
              }
            }
            frame "DispenseWater_pre" {
              w734 = u16 0 ("t")
              w777 = u16 0 ("new element/subarray")
              # "just trust me on this one"
              # "RewCalib\nOnOff"
              # "RewCalib\nOnOff"
              # "nCycle"
              # "Solenoid__R"
              # "Tdelay"
              # "delay"
              # "nCycle"
              # "Solenoid__L"
              # "Tdelay"
              # "delay"
              # "Solenoid__R"
              # "count"
              # "Solenoid_Tcycle_R"
              # "Solenoid_Tcycle_L"
              # "Solenoid__L"
              # "count"
              n428 = call "myRIO_BRig_RT_dataMTrig_Solenoid_RewCalib_OnOff__L.vi"() -> ("output_Solenoid_RewCalib_OnOff__L"=w741:i32)  [unwired: 11 in]
              n429 = call "myRIO_BRig_RT_dataMTrig_Solenoid_N__L.vi"() -> ("output_Solenoid_N__L"=w732:i32)  [unwired: 11 in]
              n430 = call "myRIO_BRig_RT_dataMTrig_Solenoid_delay__L.vi"() -> ("output_Solenoid_delay__L"=w775:i32)  [unwired: 11 in]
              n431 = call "myRIO_BRig_RT_dataMTrig_Solenoid_Tdelay__L.vi"() -> ("output_Solenoid_Tdelay__L"=w774:i32)  [unwired: 11 in]
              n432 = call "myRIO_BRig_RT_dataMTrig_Solenoid_N__R.vi"() -> ("output_Solenoid_N__R"=w730:i32)  [unwired: 11 in]
              n433 = call "myRIO_BRig_RT_dataMTrig_Solenoid_delay__R.vi"() -> ("output_Solenoid_delay__R"=w764:i32)  [unwired: 11 in]
              n434 = call "myRIO_BRig_RT_dataMTrig_Solenoid_Tdelay__R.vi"() -> ("output_Solenoid_Tdelay__R"=w763:i32)  [unwired: 11 in]
              n435 = call "myRIO_BRig_RT_dataMTrig_Solenoid_RewCalib_OnOff__R.vi"() -> ("output_Solenoid_RewCalib_OnOff__R"=w737:i32)  [unwired: 11 in]
              n436 = Index Array(array=w776, index #1=w732, index #2=w775, index #3=w774, index #4=w730, index #5=w764, index #6=w763, index #7=w741, index #8=w737) -> (element #1=w733:u16, element #2=w773:u16, element #3=w768:u16, element #4=w736:u16, element #5=w758:u16, element #6=w757:u16, element #7=w742:u16, element #8=w739:u16)
              n437 = Equal To 0?(x=w773) -> (x = 0?=w772:bool)
              n438 = Equal To 0?(x=w758) -> (x = 0?=w762:bool)
              n439 = local read "RewCalib_Trig_L"() -> (w753:bool)
              n440 = local read "RewCalib_Trig_R"() -> (w748:bool)
              n441 = Not Equal To 0?(x=w733) -> (x != 0?=w771:bool)
              n442 = Not Equal To 0?(x=w736) -> (x != 0?=w761:bool)
              n443 = local read "MTrig_Solenoid_Tcycle__L"() -> (w770:u16)
              n444 = local read "MTrig_Solenoid_Tcycle__R"() -> (w756:u16)
              n445 = Not Equal To 0?(x=w742) -> (x != 0?=w752:bool)
              n446 = Not Equal To 0?(x=w739) -> (x != 0?=w750:bool)
              n447 = Not(x=w753) -> (.not. x?=w751:bool)
              n448 = Not(x=w748) -> (.not. x?=w749:bool)
              n449 = And(x=w752, y=w751) -> (x .and. y?=w747:bool)
              n450 = And(x=w750, y=w749) -> (x .and. y?=w746:bool)
              n451 = call "myRIO_BRig_RT_dataMTrig_Solenoid_c__L.vi"() -> ("output_Solenoid_c__L"=w779:i32)  [unwired: 11 in]
              n452 = call "myRIO_BRig_RT_dataMTrig_Solenoid_c__R.vi"() -> ("output_Solenoid_c__R"=w778:i32)  [unwired: 11 in]
              n453 = Select(t=w770, s=w771, f=u16 0) -> (s? t:f=w767:u16)
              n454 = Or(x=w747, y=w746) -> (x .or. y?=w735:bool)
              n455 = Select(t=w756, s=w761, f=u16 0) -> (s? t:f=w759:u16)
              n456 = Select(t=w767, s=w772, f=w768) -> (s? t:f=w765:u16)
              n457 = Select(t=w759, s=w762, f=w757) -> (s? t:f=w754:u16)
              n458 = call "myRIO_BRig_RT_dataMTrig_Solenoid_Tcycle__L.vi"() -> ("output_Solenoid_Tcycle__L"=w766:i32)  [unwired: 11 in]
              n459 = call "myRIO_BRig_RT_dataMTrig_Solenoid_Tcycle__R.vi"() -> ("output_Solenoid_Tcycle__R"=w755:i32)  [unwired: 11 in]
              n460 = Select(t=w734, s=w735, f=w733) -> (s? t:f=w731:u16)
              n461 = Select(t=w734, s=w735, f=w736) -> (s? t:f=w729:u16)
              n462 = Select(t=myRIO_BRig_RT__Case_NonExp_stateList."Idle" ("Enum"), s=w735, f=myRIO_BRig_RT__Case_NonExp_stateList."DispenseWater" ("Enum")) -> (s? t:f=w743:T1)
              n463 = Select(t=w734, s=w735, f=w742) -> (s? t:f=w740:u16)
              n464 = Select(t=w734, s=w735, f=w739) -> (s? t:f=w738:u16)
              n465 = Replace Array Subset(array=w776, new element #1=w777, index #1=w779, new element #2=w777, index #2=w778, new element #3=w765, index #3=w766, new element #4=w754, index #4=w755, new element #5=w740, index #5=w741, new element #6=w738, index #6=w737, new element #7=w731, index #7=w732, new element #8=w729, index #8=w730) -> (w780:u16[])
            }
            frame "DispenseWater" {
              # "D"
              # "C"
              # "B"
              # "A"
              # "(A) Add COUNT and INCREMENT\n(B) Is (A) smaller than Tcycle?\n(C) Are we dispensing water or in the delay phase?\n(D) If (A) is smaller than Tcycle   AND   if we are dispensing water\n      then send TRUE to solenoid"
              # "delay"
              # "Tcycle"
              # "Solenoid__R"
              # "count"
              # "delay"
              # "Tcycle"
              # "Solenoid__L"
              # "count"
              n466 = To Unsigned Word Integer(number=w808) -> (unsigned 16bit integer=w790:u16)
              n467 = call "myRIO_BRig_RT_dataMTrig_Solenoid_delay__R.vi"() -> ("output_Solenoid_delay__R"=w794:i32)  [unwired: 11 in]
              n468 = call "myRIO_BRig_RT_dataMTrig_Solenoid_c__R.vi"() -> ("output_Solenoid_c__R"=w793:i32)  [unwired: 11 in]
              n469 = call "myRIO_BRig_RT_dataMTrig_Solenoid_Tcycle__R.vi"() -> ("output_Solenoid_Tcycle__R"=w795:i32)  [unwired: 11 in]
              n470 = call "myRIO_BRig_RT_dataMTrig_Solenoid_delay__L.vi"() -> ("output_Solenoid_delay__L"=w810:i32)  [unwired: 11 in]
              n471 = call "myRIO_BRig_RT_dataMTrig_Solenoid_c__L.vi"() -> ("output_Solenoid_c__L"=w802:i32)  [unwired: 11 in]
              n472 = call "myRIO_BRig_RT_dataMTrig_Solenoid_Tcycle__L.vi"() -> ("output_Solenoid_Tcycle__L"=w811:i32)  [unwired: 11 in]
              n473 = Index Array(array=w804, index #1=w802, index #2=w811, index #3=w810, index #4=w793, index #5=w795, index #6=w794) -> (element #1=w809:u16, element #2=w799:u16, element #3=w807:u16, element #4=w789:u16, element #5=w786:u16, element #6=w785:u16)
              n474 = Add(x=w809, y=w790) -> (x+y=w800:u16)
              n475 = Add(x=w789, y=w790) -> (x+y=w791:u16)
              n476 = Less?(x=w800, y=w799) -> (x < y?=w783:bool)
              n477 = Equal To 0?(x=w807) -> (x = 0?=w806:bool)
              n478 = Less?(x=w791, y=w786) -> (x < y?=w784:bool)
              n479 = Equal To 0?(x=w785) -> (x = 0?=w792:bool)
              n480 = And(x=w783, y=w806) -> (x .and. y?=w805:bool)
              n481 = Or(x=w783, y=w784) -> (x .or. y?=w782:bool)
              n482 = And(x=w784, y=w792) -> (x .and. y?=w787:bool)
              n483 = Select(t=w800, s=w783, f=w799) -> (s? t:f=w801:u16)
              n484 = Select(t=w791, s=w784, f=w786) -> (s? t:f=w788:u16)
              n485 = Replace Array Subset(array=w804, new element #1=w801, index #1=w802, new element #2=w788, index #2=w793) -> (w803:u16[])
              n486 = Select(t=w798, s=w782, f=myRIO_BRig_RT__Case_NonExp_stateList."DispenseWater_post" ("Enum")) -> (s? t:f=w796:T1)
            }
            frame "DispenseWater_post" {
              # "nCycle"
              # "delay"
              # "Solenoid__R"
              # "nCycle"
              # "delay"
              # "Solenoid__L"
              n487 = call "myRIO_BRig_RT_dataMTrig_Solenoid_N__L.vi"() -> ("output_Solenoid_N__L"=w829:i32)  [unwired: 11 in]
              n488 = call "myRIO_BRig_RT_dataMTrig_Solenoid_delay__L.vi"() -> ("output_Solenoid_delay__L"=w828:i32)  [unwired: 11 in]
              n489 = call "myRIO_BRig_RT_dataMTrig_Solenoid_N__R.vi"() -> ("output_Solenoid_N__R"=w825:i32)  [unwired: 11 in]
              n490 = call "myRIO_BRig_RT_dataMTrig_Solenoid_delay__R.vi"() -> ("output_Solenoid_delay__R"=w824:i32)  [unwired: 11 in]
              n491 = Index Array(array=w831, index #1=w829, index #2=w828, index #3=w825, index #4=w824) -> (element #1=w833:u16, element #2=w832:u16, element #3=w816:u16, element #4=w818:u16)
              n492 = Not Equal To 0?(x=w833) -> (x != 0?=w834:bool)
              n493 = Not Equal To 0?(x=w816) -> (x != 0?=w817:bool)
              n494 = case shown="True" w817 {
                selector: w817 -> [_ w838]
                tunnel: w816 -> [w836 w844]
                tunnel: w818 -> [_ w845]
                tunnel: [w836 w842] -> w815
                tunnel: [u16 0 w841] -> w814
                tunnel: [_ w838] -> w813
                frame False {
                }
                frame True {
                  n495 = Equal To 0?(x=w845) -> (x = 0?=w837:bool)
                  n496 = Decrement(x=w844) -> (x-1=w843:u16)
                  n497 = Select(t=w843, s=w837, f=w844) -> (s? t:f=w842:u16)
                  n498 = Select(t=u16 1, s=w837, f=u16 0) -> (s? t:f=w841:u16)
                }
              }
              n499 = case shown="True" w834 {
                selector: w834 -> [_ w849]
                tunnel: w833 -> [w847 w855]
                tunnel: w832 -> [_ w856]
                tunnel: [w847 w853] -> w827
                tunnel: [u16 0 w852] -> w826
                tunnel: [_ w849] -> w823
                frame False {
                }
                frame True {
                  n500 = Equal To 0?(x=w856) -> (x = 0?=w848:bool)
                  n501 = Decrement(x=w855) -> (x-1=w854:u16)
                  n502 = Select(t=w854, s=w848, f=w855) -> (s? t:f=w853:u16)
                  n503 = Select(t=u16 1, s=w848, f=u16 0) -> (s? t:f=w852:u16)
                }
              }
              n504 = Or(x=w823, y=w813) -> (x .or. y?=w822:bool)
              n505 = Replace Array Subset(array=w831, new element #1=w827, index #1=w829, new element #2=w826, index #2=w828, new element #3=w815, index #3=w825, new element #4=w814, index #4=w824) -> (w830:u16[])
              n506 = Select(t=myRIO_BRig_RT__Case_NonExp_stateList."DispenseWater_pre" ("Enum"), s=w822, f=myRIO_BRig_RT__Case_NonExp_stateList."Idle" ("Enum")) -> (s? t:f=w819:T1)
            }
            frame "TestConnection" {
              n507 = local read "Host Password"() -> (w863:string)
              n508 = local read "Host UserName"() -> (w864:string)
              n509 = call "myRIO_BRig_RT_comm_webdav_testConnect.vi"("input_password"=w863, "input_username"=w864) -> ("output_Iconnected"=w861:bool)  [unwired: 9 in]
              n510 = Select(t="Connection accepted!" ("message"), s=w861, f="Error!") -> (s? t:f=w859:string)
              n511 = One Button Dialog(message=w859) -> ()  [unwired: 1 in, 1 out]
            }
            frame "SendData" {
              n512 = local read "Data Set Prefix"() -> (w866:string)
              n513 = local read "Host Password"() -> (w867:string)
              n514 = local read "Host UserName"() -> (w868:string)
              n515 = call "myRIO_BRig_RT_comm_webdav_sendData_all.vi"("Host Filename Prefix"=w866, "Host Password"=w867, "Host UserName"=w868) -> ()  [unwired: 9 in]
            }
            frame "Get_FPGA_count_per_ms" {
              n516 = case shown="False" w882 {
                selector: w882 -> [w885 _]
                tunnel: w880 -> [_ w898]
                tunnel: [w889 w898] -> w879
                tunnel: w878 -> [w888 w896]
                tunnel: w877 -> [w887 w895]
                tunnel: [w886 w893] -> w876
                tunnel: [w885 w892] -> w875
                frame False {
                  n517 = Get Date/Time In Seconds() -> (seconds since 1Jan1904=w890:timestamp)
                  n518 = xnode "Read/Write Control"("FPGA VI Reference In"=w888, "error in"=w887, "timeTrial"=TRUE) -> ("error out"=w886:errorcluster)  [unwired: 1 out]
                  n519 = To Double Precision Float(number=w890) -> (double precision float=w889:dbl)
                  n520 = local write "get_countPerMS"(w885) -> ()
                }
                frame True {
                  w894 = 1.0
                  n521 = Get Date/Time In Seconds() -> (seconds since 1Jan1904=w899:timestamp)
                  n522 = To Double Precision Float(number=w899) -> (double precision float=w900:dbl)
                  n523 = Subtract(x=w900, y=w898) -> (x-y=w897:dbl)
                  n524 = Less Or Equal?(x=w894, y=w897) -> (x <= y?=w892:bool)
                  n525 = case shown="True" w892 {
                    tunnel: w896 -> [_ w913]
                    tunnel: w895 -> [w901 w912]
                    tunnel: w894 -> [_ w903]
                    tunnel: [w901 w902] -> w893
                    frame False {
                    }
                    frame True {
                      n526 = xnode "Read/Write Control"("FPGA VI Reference In"=w913, "error in"=w912) -> ("FPGA VI Reference Out"=w910:refnum<k20>, "error out"=w909:errorcluster, "count_timeTrial"=w904:u32)
                      n527 = Multiply(x=w903, y=1000.0) -> (x*y=w907:dbl)
                      n528 = To Double Precision Float(number=w904) -> (double precision float=w906:dbl)
                      n529 = Divide(x=w906, y=w907) -> (x/y=w908:dbl)
                      n530 = local write "f_millisec2count"(w908) -> ()
                      n531 = xnode "Read/Write Control"("FPGA VI Reference In"=w910, "error in"=w909, "timeTrial"=FALSE) -> ("error out"=w902:errorcluster)  [unwired: 1 out]
                    }
                  }
                }
              }
              "error out 5" <- w876
              n532 = Select(t=myRIO_BRig_RT__Case_NonExp_stateList."Idle" ("Enum"), s=w875, f=w873) -> (s? t:f=w872:T1)
            }
            frame "End" {
            }
          }
          n533 = local read "MTrig_Audio_trig__R"() -> (w119:bool)
          n534 = local read "MTrig_Audio_trig__L"() -> (w118:bool)
          n535 = local read "START"() -> (w114:bool)
          n536 = local read "STOP_abort"() -> (w113:bool)
          n537 = local read "MTrig_Laser_trig"() -> (w120:bool)
          n538 = call "myRIO_BRig_RT_dataMTrig_main__v2.vi"("input_dataMTrig"=w122, "input_Audio_trig_L"=w118, "input_Audio_trig_R"=w119, "input_Laser_trig"=w120) -> ("output_dataMTrig"=w121:u16[], "output_Audio_L"=w98:bool, "output_Audio_R"=w109:bool, "output_Laser"=w101:bool)  [unwired: 12 in]
          n539 = Or(x=w114, y=w113) -> (x .or. y?=w112:bool)
          n540 = Select(t=myRIO_BRig_RT__Case_NonExp_stateList."End" ("Enum"), s=w112, f=w111) -> (s? t:f=w110:T1)
          n541 = Or(x=w119, y=w120) -> (x .or. y?=w117:bool)
          n542 = Or(x=w117, y=w118) -> (x .or. y?=w116:bool)
          n543 = case shown="True" w116 {
            frame False {
            }
            frame True {
              w135 = FALSE
              n544 = local write "MTrig_Audio_trig__R"(w135) -> ()
              n545 = local write "MTrig_Audio_trig__L"(w135) -> ()
              n546 = local write "MTrig_Laser_trig"(w135) -> ()
            }
          }
          n547 = xnode "Read/Write Control"("FPGA VI Reference In"=w87, "error in"=w86, "A1_SR"=w123, "A3_SL"=w124, "audioTrigger_L"=w98, "audioTrigger_R"=w109, "laserResponse_reward_LED"="laserResponse_reward_LED", "laserResponse_wrong_LED"="laserResponse_wrong_LED", "laserResponse_reward"="laserResponse_reward", "laserResponse_wrong"="laserResponse_wrong", "SelectionState"="SelectionState", "ignoreWrong"="ignoreWrong", "Left(F)_or_Right(T)"="Left(F)_or_Right(T)", "laserMTrig"=w101) -> ("FPGA VI Reference Out"=w129:refnum<k20>, "error out"=w128:errorcluster, "SelectReward"=→"SelectReward":bool, "SelectWrong"=→"SelectWrong":bool, "AnaIn_0"=→"tempAI0":i16)
          n548 = node-c288() -> ()  [unwired: 1 in, 1 out]
          "cState_NonExp" <- w127
        }
        n549 = node-c288(w69) -> ()  [unwired: 1 out]
        n550 = flat-sequence {
          tunnel: w62 -> [w80]
          tunnel: [w80] -> w61
          tunnel: w60 -> [w79]
          tunnel: [w79] -> w59
          frame #0 {
            w78 = FALSE
            n551 = local write "STOP_endBlock"(w78) -> ()
            n552 = local write "STOP_endTrial"(w78) -> ()
          }
        }
      }
      frame True {
        w936 = u16 0
        w939 = u8 0
        w940 = FALSE ("SelectionState")
        w945 = u16 0 ("idxDataBlock")
        w947 = u16 100 ("new element/subarray")
        w948 = u16 100 ("new element/subarray")
        w968 = T6 refnum items=["Session NI_WebDAV"] ("output_hSession")
        w977 = FALSE
        w978 = u16 0
        w923 = FALSE
        # "audio__L\naudio__R"
        # "Audio params"
        # "nRewards"
        # "idxDataBlock"
        # "Solenoid_Tdelay_R"
        # "Solenoid_Tdelay_L"
        # "RewCalib_N__R"
        # "RewCalib_N__L"
        # "Save dataLick to file\nSend file to Host\nSave dataMTrig\nSend file to Host\nDisconnect"
        # "dataTrial"
        # "dataTrial"
        # "Solenoid_Tcycle_R"
        # "Solenoid_Tcycle_L"
        # "Laser_Tcycle"
        # "Audio_Tcycle_R"
        # "Audio_Tcycle_L"
        # "dataLick"
        # "dataLC"
        # "dataLC"
        # "dataBlock"
        # "dataBlock"
        # "dataMTrig"
        # "dataMTrig"
        # "dataExp"
        # "dataCurrent"
        # "dataExp"
        # "dataCurrent"
        # "spout"
        # "state"
        n553 = call "myRIO_BRig_RT_dataMTrig_Solenoid_Tcycle__L.vi"() -> ("output_Solenoid_Tcycle__L"=w974:i32)  [unwired: 11 in]
        n554 = call "myRIO_BRig_RT_dataMTrig_Solenoid_Tcycle__R.vi"() -> ("output_Solenoid_Tcycle__R"=w973:i32)  [unwired: 11 in]
        n555 = call "myRIO_BRig_RT_dataMTrig_Audio_Tcycle__L.vi"() -> ("output_Audio_Tcycle__L"=w972:i32)  [unwired: 11 in]
        n556 = call "myRIO_BRig_RT_dataMTrig_Audio_Tcycle__R.vi"() -> ("output_Audio_Tcycle__R"=w971:i32)  [unwired: 11 in]
        n557 = call "myRIO_BRig_RT_dataMTrig_Laser_Tcycle.vi"() -> ("output_Laser_Tcycle"=w970:i32)  [unwired: 11 in]
        n558 = local read "MTrig_Solenoid_Tcycle__L"() -> (w953:u16)
        n559 = local read "MTrig_Solenoid_Tcycle__R"() -> (w952:u16)
        n560 = local read "Tcycle_Reward_L"() -> (w949:u16)
        n561 = local read "Tcycle_Reward_R"() -> (w950:u16)
        n562 = local read "MTrig_Laser_Tcycle"() -> (w951:u16)
        n563 = call "myRIO_BRig_RT_dataMTrig_Solenoid_RewCalib_nCycle__L.vi"() -> ("output_Solenoid_RewCalib_nCycle__L"=w956:i32)  [unwired: 11 in]
        n564 = call "myRIO_BRig_RT_dataMTrig_Solenoid_Tdelay__L.vi"() -> ("output_Solenoid_Tdelay__L"=w958:i32)  [unwired: 11 in]
        n565 = call "myRIO_BRig_RT_dataMTrig_Solenoid_RewCalib_nCycle__R.vi"() -> ("output_Solenoid_RewCalib_nCycle__R"=w957:i32)  [unwired: 11 in]
        n566 = call "myRIO_BRig_RT_dataMTrig_Solenoid_Tdelay__R.vi"() -> ("output_Solenoid_Tdelay__R"=w959:i32)  [unwired: 11 in]
        n567 = case shown="False" w930 {
          selector: w930 -> [_ w1000]
          tunnel: w929 -> [w997 w1002]
          tunnel: [w998 w1002] -> w928
          tunnel: w927 -> [_ w1001]
          tunnel: [w999 w1001] -> w926
          tunnel: [w996 w1000] -> w924
          frame False {
            n568 = call "myRIO__TCP_connect_forWriting.vi"("input_error"=w997) -> ("output_error"=w998:errorcluster, "output_connected"=w996:bool, "output_hTCP"=w999:refnum<k5>)  [unwired: 8 in]
          }
          frame True {
          }
        }
        n569 = call "myRIO_BRig_RT_dataLick_init.vi"() -> ("output_dataLick"=w980:u16[][])  [unwired: 11 in]
        n570 = call "myRIO_BRig_RT_dataCurrent_init.vi"() -> ("output_dataCurrent"=w987:u16[])  [unwired: 11 in]
        n571 = call "myRIO_BRig_RT_dataExp_init.vi"() -> ("output_dataExp"=w986:u16[])  [unwired: 11 in]
        n572 = call "myRIO_BRig_RT_dataMTrig_init.vi"() -> ("output_dataMTrig"=w976:u16[])  [unwired: 5 in]
        n573 = call "myRIO_BRig_RT_dataLC_init.vi"() -> ("output_dataLC"=w984:u16[])  [unwired: 11 in]
        n574 = call "myRIO_BRig_RT_dataBlock_init.vi"() -> ("output_dataBlock"=w985:u16[][])  [unwired: 11 in]
        n575 = call "myRIO_BRig_RT_dataTrial_init.vi"() -> ("output_dataTrial"=w969:u16[][])  [unwired: 11 in]
        n576 = xnode "Read/Write Control"("FPGA VI Reference In"=w941, "error in"=w942, "SelectionState"=w940, "laserResponse_reward"=w940, "laserResponse_wrong"=w940, "laserResponse_reward_LED"=w940, "laserResponse_wrong_LED"=w940, "Left(F)_or_Right(T)"=w940, "ignoreWrong"=w940, "SelectionState"=w940) -> ("FPGA VI Reference Out"=w943:refnum<k20>, "error out"=w944:errorcluster)
        n577 = local write "I_connect_TCP"(w924) -> ()
        n578 = Replace Array Subset(array=w976, new element #1=w948, index #1=w956, new element #2=w948, index #2=w957, new element #3=w947, index #3=w958, new element #4=w947, index #4=w959, new element #5=w953, index #5=w974, new element #6=w952, index #6=w973, new element #7=w949, index #7=w972, new element #8=w950, index #8=w971, new element #9=w951, index #9=w970) -> (w975:u16[])
        n579 = call "myRIO_BRig_RT_dataAnalog_init.vi"() -> ("output_dataAnalog"=w935:u16[][])  [unwired: 11 in]
        n580 = Get Date/Time In Seconds() -> (seconds since 1Jan1904=w955:timestamp)
        n581 = To Double Precision Float(number=w955) -> (double precision float=w954:dbl)
        n582 = node-c288() -> (w995:T3)  [unwired: 4 in]
        n583 = timed-loop {
          timing: w995 -> [_]
          timing-out: [_] -> w994
          shift-right: [w1114] -> _
          shift-left: myRIO_BRig_RT__Case_Exp_stateList."Start1" ("Enum") -> [w1050]
          shift-right: [w1164] -> _
          shift-left: enum16{"Left", "Right"}."Left" -> [w1166]
          tunnel: w943 -> [w1163]
          tunnel: w944 -> [w1162]
          shift-right: [w1157] -> _
          shift-left: w992 -> [w1161]
          shift-right: [w1156] -> _
          shift-left: w991 -> [w1160]
          tunnel: [w1139] -> w989
          tunnel: [w1140] -> w990
          shift-right: [w1141] -> w960
          shift-left: w987 -> [w1106]
          shift-right: [w1155] -> _
          shift-left: w986 -> [w1101]
          shift-right: [w1128] -> w964
          shift-left: w975 -> [w1129]
          shift-right: [w1153] -> _
          shift-left: w985 -> [w1154]
          shift-right: [w1151] -> _
          shift-left: w984 -> [w1152]
          shift-right: [w1143] -> w966
          shift-left: w980 -> [w1144]
          shift-right: [w1130] -> _
          shift-left: w978 -> [w1138]
          shift-right: [w1098] -> _
          shift-left: w939 -> [w1137]
          shift-right: [w1131] -> _
          shift-left: w978 -> [w1136]
          shift-right: [w1132] -> _
          shift-left: w939 -> [w1135]
          shift-right: [w1099] -> _
          shift-left: w977 -> [w1133]
          shift-right: [w1100] -> _
          shift-left: w977 -> [w1134]
          shift-right: [w1112] -> _
          shift-left: w969 -> [w1113]
          shift-right: [w1111] -> w962
          shift-left: w968 -> [w1109]
          shift-right: [w1110] -> w963
          shift-left: FALSE ("output_Iconnected") -> [w1108]
          tunnel: "Data Set Prefix" -> [w1107]
          tunnel: [w1107] -> w961
          shift-right: [w1083] -> _
          shift-left: w923 -> [w1105]
          tunnel: w954 -> [w1102]
          shift-right: [w1096] -> _
          shift-left: 0 ("idxDataBlock") -> [w1097]
          shift-right: [w1093] -> _
          shift-left: w945 -> [w1095]
          shift-right: [w1092] -> _
          shift-left: w945 -> [w1094]
          shift-right: [w1082] -> _
          shift-left: w923 -> [w1088]
          shift-right: [w1085] -> _
          shift-left: w923 -> [w1087]
          shift-right: [w1084] -> _
          shift-left: w923 -> [w1086]
          shift-right: [w1070] -> w933
          shift-left: 0 -> [w1054]
          shift-right: [w1053] -> _
          shift-left: w936 -> [w1065]
          shift-right: [w1052] -> _
          shift-left: w936 -> [w1061]
          shift-right: [w1074] -> _
          shift-left: FALSE -> [w1074]
          shift-right: [w1060] -> _
          shift-left: w936 -> [w1068]
          shift-right: [w1071] -> w934
          shift-left: w935 -> [w1072]
          tunnel: w926 -> [w1059]
          tunnel: [w1058] -> w932
          tunnel: w924 -> [w1055]
          tunnel: [w1055] -> w931
          tunnel: w928 -> [w1057]
          tunnel: [w1056] -> w925
          shift-right: [w1046] -> _
          shift-left: w923 -> [w1047]
          shift-right: [w1044] -> _
          shift-left: w923 -> [w1045]
          stop <- w1150 stop-if-true
          # "Sel"
          # "Sel"
          # "Cue1"
          # "Cue1"
          # "ENL1"
          # "ENL1"
          # "iState"
          # "dataAnalog"
          # "index"
          # "iEvent"
          # "iBlock"
          # "iTrial"
          # "Laser"
          # "Audio R"
          # "Audio L"
          # "Solenoid R"
          # "Solenoid L"
          # "manual triggering"
          # "dataTrial"
          # "dataBlock"
          # "nRewards"
          # "dataExp"
          # "dataCurrent"
          # "audio__L\naudio__R"
          # "time stamp"
          # "Audio params"
          # "nRewards"
          # "idxDataBlock"
          # "idxDataBlock"
          # "activate"
          # "audio__L\naudio__R"
          # "amp__R\nfreq__R"
          # "amp__L\nfreq__L"
          # "dataLC"
          # "solenoid__R"
          # "solenoid__L"
          # "Did a lick occur?"
          # "Update lick counter"
          # "spout"
          # "spout"
          # "state"
          # "state"
          n584 = node-c288() -> ()  [unwired: 1 in, 1 out]
          n585 = local read "MTrig_Solenoid_trig__L"() -> (w1126:bool)
          n586 = local read "MTrig_Solenoid_trig__R"() -> (w1125:bool)
          n587 = local read "MTrig_Audio_trig__L"() -> (w1124:bool)
          n588 = local read "MTrig_Audio_trig__R"() -> (w1123:bool)
          n589 = xnode "Read/Write Control"("FPGA VI Reference In"=w1163, "error in"=w1162) -> ("FPGA VI Reference Out"=w1091:refnum<k20>, "error out"=w1090:errorcluster, "A2_LickL"=w1157:u32, "A4_LickR"=w1156:u32)
          "A2" <- w1157
          "A4" <- w1156
          n590 = local read "MTrig_Laser_trig"() -> (w1122:bool)
          n591 = Greater?(x=w1157, y=w1161) -> (0:w1159:bool)
          n592 = Greater?(x=w1156, y=w1160) -> (0:w1158:bool)
          n593 = Or(x=w1159, y=w1158) -> (x .or. y?=w1165:bool)
          n594 = call "myRIO_BRig_RT_dataMTrig_main.vi"("input_dataMTrig"=w1129, "input_Solenoid_trig_L"=w1126, "input_Solenoid_trig_R"=w1125, "input_Audio_trig_L"=w1124, "input_Audio_trig_R"=w1123, "input_Laser_trig"=w1122) -> ("output_Laser"=w1080:bool, "output_dataMTrig"=w1128:u16[], "output_Solenoid_L"=w1116:bool, "output_Solenoid_R"=w1118:bool, "output_Audio_L"=w1120:bool, "output_Audio_R"=w1121:bool)  [unwired: 8 in]
          n595 = Compound Arithmetic op=OR(w1126, w1125, w1124, w1123, w1122) -> (w1127:bool)
          n596 = case shown="True" w1127 {
            frame False {
            }
            frame True {
              w1167 = FALSE
              n597 = local write "MTrig_Solenoid_trig__L"(w1167) -> ()
              n598 = local write "MTrig_Solenoid_trig__R"(w1167) -> ()
              n599 = local write "MTrig_Audio_trig__L"(w1167) -> ()
              n600 = local write "MTrig_Audio_trig__R"(w1167) -> ()
              n601 = local write "MTrig_Laser_trig"(w1167) -> ()
            }
          }
          n602 = case shown="\"endTrial2\"" w1050 {
            selector: w1050 -> [_ _ _ _ _ _ _ _ _ _ _ _ _ _ _ _ _ _ _ _ _ w1960 _ w2025 _ _ _ _ _ w2166 _ w2243 _ _ _ _ _ w2398 _ w2472 _ w2536 _ w2580 _ _ w2650 _ _ _ _ _ w2821 _ _ _ _ _ _ _ _ _ _ _ _ _ _ _ _ _ _ _]
            tunnel: [myRIO_BRig_RT__Case_Exp_stateList."Start2" ("Enum") myRIO_BRig_RT__Case_Exp_stateList."Start3" ("Enum") myRIO_BRig_RT__Case_Exp_stateList."saveSettings1" ("Enum") myRIO_BRig_RT__Case_Exp_stateList."saveSettings2" ("Enum") myRIO_BRig_RT__Case_Exp_stateList."saveSettings3" ("Enum") myRIO_BRig_RT__Case_Exp_stateList."saveSettings4_LC_ENL" ("Enum") myRIO_BRig_RT__Case_Exp_stateList."saveSettings5_LC_Cue" ("Enum") myRIO_BRig_RT__Case_Exp_stateList."saveSettings6_LC_Other" ("Enum") myRIO_BRig_RT__Case_Exp_stateList."setSettings_Audio" ("Enum") myRIO_BRig_RT__Case_Exp_stateList."setSettings_Laser" ("Enum") myRIO_BRig_RT__Case_Exp_stateList."commConnect" ("Enum") w1690 myRIO_BRig_RT__Case_Exp_stateList."initTrial" ("Enum") w1735 myRIO_BRig_RT__Case_Exp_stateList."initTrial3" ("Enum") myRIO_BRig_RT__Case_Exp_stateList."initTrial_LC_ENL1" ("Enum") myRIO_BRig_RT__Case_Exp_stateList."ENL1_pre" ("Enum") myRIO_BRig_RT__Case_Exp_stateList."initTrial_LC_Cue1" ("Enum") myRIO_BRig_RT__Case_Exp_stateList."initTrial_LC_Sel" ("Enum") myRIO_BRig_RT__Case_Exp_stateList."initTrial4" ("Enum") w1920 w1957 myRIO_BRig_RT__Case_Exp_stateList."ENL1Penalty" ("Enum") w2026 myRIO_BRig_RT__Case_Exp_stateList."endExp" ("Enum") myRIO_BRig_RT__Case_Exp_stateList."endExp" ("Enum") myRIO_BRig_RT__Case_Exp_stateList."endExp" ("Enum") myRIO_BRig_RT__Case_Exp_stateList."endExp" ("Enum") w2121 w2165 myRIO_BRig_RT__Case_Exp_stateList."Cue1Penalty" ("Enum") w2241 myRIO_BRig_RT__Case_Exp_stateList."endExp" ("Enum") myRIO_BRig_RT__Case_Exp_stateList."endExp" ("Enum") myRIO_BRig_RT__Case_Exp_stateList."endExp" ("Enum") myRIO_BRig_RT__Case_Exp_stateList."endExp" ("Enum") w2338 w2404 myRIO_BRig_RT__Case_Exp_stateList."SelectReward" ("Enum") w2473 myRIO_BRig_RT__Case_Exp_stateList."SelectRewardPost" ("Enum") w2537 myRIO_BRig_RT__Case_Exp_stateList."SelectWrong" ("Enum") w2576 myRIO_BRig_RT__Case_Exp_stateList."endTrial1" ("Enum") myRIO_BRig_RT__Case_Exp_stateList."SelectTimeout" ("Enum") w2652 myRIO_BRig_RT__Case_Exp_stateList."endTrial1" ("Enum") myRIO_BRig_RT__Case_Exp_stateList."endTrial2" ("Enum") myRIO_BRig_RT__Case_Exp_stateList."saveData_dataBlock" ("Enum") w2734 w2804 w2821 myRIO_BRig_RT__Case_Exp_stateList."initBlock" ("Enum") w2848 myRIO_BRig_RT__Case_Exp_stateList."commUpload_dataCurrent" ("Enum") myRIO_BRig_RT__Case_Exp_stateList."commUpload_dataExp" ("Enum") myRIO_BRig_RT__Case_Exp_stateList."commUpload_dataLC" ("Enum") myRIO_BRig_RT__Case_Exp_stateList."commUpload_dataTrial" ("Enum") myRIO_BRig_RT__Case_Exp_stateList."endTrial3" ("Enum") myRIO_BRig_RT__Case_Exp_stateList."saveData_dataCurrent" ("Enum") myRIO_BRig_RT__Case_Exp_stateList."saveData_dataExp" ("Enum") myRIO_BRig_RT__Case_Exp_stateList."saveData_dataLC" ("Enum") myRIO_BRig_RT__Case_Exp_stateList."saveData_dataTrial" ("Enum") myRIO_BRig_RT__Case_Exp_stateList."commUpload_pre" ("Enum") myRIO_BRig_RT__Case_Exp_stateList."initBlock" ("Enum") myRIO_BRig_RT__Case_Exp_stateList."initBlock" ("Enum") myRIO_BRig_RT__Case_Exp_stateList."empty_endTrial2" ("Enum") myRIO_BRig_RT__Case_Exp_stateList."empty_endTrial3" ("Enum") myRIO_BRig_RT__Case_Exp_stateList."empty_endTrial4" ("Enum") myRIO_BRig_RT__Case_Exp_stateList."initTrial" ("Enum") myRIO_BRig_RT__Case_Exp_stateList."initTrial" ("Enum")] -> w1114
            tunnel: [w1193 w1212 w1234 w1289 w1337 w1404 w1468 w1532 w1576 w1602 w1661 w1667 w1698 w1717 w1751 w1781 w1816 w1840 w1866 w1895 w1936 w1973 w2003 w2030 w2046 w2068 w2087 w2106 w2140 w2187 w2212 w2240 w2261 w2282 w2301 w2320 w2349 w2422 w2447 w2470 w2484 w2534 w2558 w2590 w2611 w2631 w2662 w2685 w2697 w2716 w2758 w2777 w2820 w2837 w2851 w2885 w2906 w2927 w2948 w2969 w2997 w3017 w3044 w3064 w3089 w3108 w3127 w3146 w3165 w3184 w3203 w3222] -> w1164
            tunnel: w1166 -> [w1193 w1212 w1234 w1289 w1337 w1404 w1468 w1532 w1576 w1602 w1661 w1689 w1698 w1717 w1751 w1781 w1816 w1840 w1866 w1895 w1936 w1973 w2003 w2030 w2046 w2068 w2087 w2106 w2140 w2187 w2212 w2240 w2261 w2282 w2301 w2320 w2349 w2422 w2447 w2470 w2484 w2534 w2558 w2590 w2611 w2631 w2662 w2685 w2697 w2716 w2758 w2777 w2820 w2837 w2851 w2885 w2906 w2927 w2948 w2969 w2997 w3017 w3044 w3064 w3089 w3108 w3127 w3146 w3165 w3184 w3203 w3222]
            tunnel: w1165 -> [w1196 w1215 w1231 w1292 w1340 w1407 w1471 w1535 w1579 w1605 w1664 w1683 w1709 w1736 w1769 w1797 w1830 w1853 w1879 w1908 w1923 w1954 w2006 w2033 w2052 w2071 w2090 w2109 w2120 w2164 w2220 w2247 w2266 w2285 w2304 w2323 w2347 w2420 w2457 w2480 w2515 w2542 w2569 w2593 w2610 w2643 w2667 w2682 w2705 w2715 w2769 w2803 w2824 w2834 w2860 w2888 w2909 w2930 w2951 w2972 w3000 w3020 w3047 w3067 w3092 w3111 w3130 w3149 w3168 w3187 w3206 w3225]
            tunnel: w1159 -> [w1195 w1214 w1232 w1291 w1339 w1406 w1470 w1534 w1578 w1604 w1663 w1682 w1708 w1737 w1768 w1798 w1831 w1854 w1880 w1909 w1946 w1975 w2005 w2032 w2051 w2070 w2089 w2108 w2154 w2188 w2219 w2246 w2265 w2284 w2303 w2322 w2348 w2419 w2456 w2479 w2514 w2541 w2568 w2592 w2609 w2642 w2666 w2683 w2706 w2714 w2768 w2802 w2823 w2835 w2861 w2887 w2908 w2929 w2950 w2971 w2999 w3019 w3046 w3066 w3091 w3110 w3129 w3148 w3167 w3186 w3205 w3224]
            tunnel: w1158 -> [w1194 w1213 w1233 w1290 w1338 w1405 w1469 w1533 w1577 w1603 w1662 w1681 w1707 w1738 w1767 w1799 w1832 w1855 w1881 w1910 w1945 w1974 w2004 w2031 w2050 w2069 w2088 w2107 w2153 w2189 w2218 w2245 w2264 w2283 w2302 w2321 w2366 w2423 w2455 w2478 w2513 w2540 w2567 w2591 w2608 w2641 w2665 w2684 w2707 w2713 w2767 w2801 w2822 w2836 w2862 w2886 w2907 w2928 w2949 w2970 w2998 w3018 w3045 w3065 w3090 w3109 w3128 w3147 w3166 w3185 w3204 w3223]
            tunnel: [w1196 w1215 w1231 w1292 w1340 w1407 w1471 w1535 w1579 w1605 w1664 w1683 w1709 w1736 w1769 w1797 w1830 w1853 w1879 w1908 w1923 w1954 w2006 w2033 w2052 w2071 w2090 w2109 w2120 w2164 w2220 w2247 w2266 w2285 w2304 w2323 w2347 w2420 w2457 w2480 w2515 w2542 w2569 w2593 w2610 w2643 w2667 w2682 w2705 w2715 w2769 w2803 w2824 w2834 w2860 w2888 w2909 w2930 w2951 w2972 w3000 w3020 w3047 w3067 w3092 w3111 w3130 w3149 w3168 w3187 w3206 w3225] -> w1147
            tunnel: [w1195 w1214 w1232 w1291 w1339 w1406 w1470 w1534 w1578 w1604 w1663 w1682 w1708 w1737 w1768 w1798 w1831 w1854 w1880 w1909 w1946 w1975 w2005 w2032 w2051 w2070 w2089 w2108 w2154 w2188 w2219 w2246 w2265 w2284 w2303 w2322 w2348 w2419 w2456 w2479 w2514 w2541 w2568 w2592 w2609 w2642 w2666 w2683 w2706 w2714 w2768 w2802 w2823 w2835 w2861 w2887 w2908 w2929 w2950 w2971 w2999 w3019 w3046 w3066 w3091 w3110 w3129 w3148 w3167 w3186 w3205 w3224] -> w1146
            tunnel: [w1194 w1213 w1233 w1290 w1338 w1405 w1469 w1533 w1577 w1603 w1662 w1681 w1707 w1738 w1767 w1799 w1832 w1855 w1881 w1910 w1945 w1974 w2004 w2031 w2050 w2069 w2088 w2107 w2153 w2189 w2218 w2245 w2264 w2283 w2302 w2321 w2366 w2423 w2455 w2478 w2513 w2540 w2567 w2591 w2608 w2641 w2665 w2684 w2707 w2713 w2767 w2801 w2822 w2836 w2862 w2886 w2907 w2928 w2949 w2970 w2998 w3018 w3045 w3065 w3090 w3109 w3128 w3147 w3166 w3185 w3204 w3223] -> w1145
            tunnel: w1106 -> [w1192 w1211 w1230 w1256 w1313 w1381 w1467 w1531 w1575 w1600 w1621 w1688 w1697 w1734 w1740 w1782 w1811 w1837 w1865 w1894 w1935 w1959 w1997 w2029 w2047 w2067 w2086 w2105 w2124 w2184 w2211 w2244 w2262 w2281 w2300 w2319 w2333 w2400 w2439 w2475 w2486 w2539 w2559 w2589 w2607 w2632 w2664 w2681 w2694 w2718 w2738 w2775 w2819 w2838 w2863 w2882 w2903 w2924 w2945 w2956 w2986 w3005 w3029 w3061 w3078 w3098 w3117 w3136 w3155 w3174 w3193 w3212]
            tunnel: w1101 -> [w1191 w1210 w1229 w1287 w1335 w1401 w1465 w1529 w1573 w1593 w1657 w1687 w1706 w1733 w1748 w1780 w1818 w1843 w1869 w1898 w1938 w1972 w1996 w2027 w2049 w2066 w2085 w2104 w2142 w2186 w2209 w2239 w2263 w2280 w2299 w2318 w2359 w2421 w2453 w2477 w2507 w2535 w2560 w2587 w2606 w2634 w2661 w2680 w2704 w2721 w2737 w2794 w2818 w2839 w2864 w2881 w2902 w2923 w2944 w2957 w2994 w3014 w3025 w3060 w3086 w3105 w3124 w3143 w3162 w3181 w3200 w3219]
            tunnel: [w1192 w1211 w1230 w1256 w1313 w1380 w1467 w1531 w1575 w1600 w1643 w1672 w1697 w1722 w1740 w1782 w1811 w1836 w1864 w1893 w1939 w1958 w1998 w2028 w2047 w2067 w2086 w2105 w2149 w2183 w2210 w2242 w2262 w2281 w2300 w2319 w2360 w2397 w2454 w2474 w2508 w2538 w2561 w2588 w2607 w2635 w2663 w2681 w2693 w2717 w2738 w2773 w2819 w2838 w2863 w2882 w2903 w2924 w2945 w2956 w2986 w3005 w3029 w3061 w3078 w3098 w3117 w3136 w3155 w3174 w3193 w3212] -> w1142
            tunnel: [w1191 w1210 w1229 w1286 w1334 w1396 w1465 w1529 w1573 w1593 w1657 w1686 w1706 w1732 w1748 w1780 w1818 w1843 w1869 w1898 w1938 w1972 w1996 w2027 w2049 w2066 w2085 w2104 w2142 w2186 w2209 w2239 w2263 w2280 w2299 w2318 w2359 w2421 w2453 w2477 w2507 w2535 w2560 w2587 w2606 w2634 w2661 w2680 w2704 w2721 w2737 w2794 w2818 w2839 w2864 w2881 w2902 w2923 w2944 w2957 w2994 w3014 w3028 w3060 w3086 w3105 w3124 w3143 w3162 w3181 w3200 w3219] -> w1155
            tunnel: [_ _ _ _ _ _ _ _ _ _ _ _ _ _ _ _ _ _ _ _ _ _ _ _ _ _ _ _ _ _ _ _ _ _ _ _ _ _ _ w2468 _ _ _ _ _ _ _ _ _ _ _ _ _ _ _ _ _ _ _ _ _ _ _ _ _ _ _ _ _ _ _ _] -> w1117
            tunnel: [_ _ _ _ _ _ _ _ _ _ _ _ _ _ _ _ _ _ _ _ _ _ _ _ _ _ _ _ _ _ _ _ _ _ _ _ _ _ _ w2469 _ _ _ _ _ _ _ _ _ _ _ _ _ _ _ _ _ _ _ _ _ _ _ _ _ _ _ _ _ _ _ _] -> w1119
            tunnel: w1154 -> [w1189 w1208 w1227 w1258 w1315 w1402 w1466 w1530 w1574 w1598 w1658 w1684 w1699 w1730 w1760 w1795 w1828 w1833 w1861 w1890 w1937 w1971 w1993 w2023 w2048 w2064 w2083 w2102 w2148 w2185 w2208 w2237 w2259 w2278 w2297 w2316 w2358 w2417 w2445 w2476 w2488 w2532 w2557 w2585 w2604 w2633 w2660 w2678 w2696 w2723 w2765 w2786 w2816 w2841 w2866 w2879 w2900 w2921 w2942 w2966 w2980 w3007 w3035 w3054 w3080 w3099 w3118 w3137 w3156 w3175 w3194 w3213]
            tunnel: [w1189 w1208 w1227 w1258 w1315 w1402 w1466 w1530 w1574 w1598 w1658 w1684 w1696 w1730 w1760 w1795 w1828 w1833 w1861 w1890 w1937 w1971 w1993 w2023 w2048 w2064 w2083 w2102 w2148 w2185 w2208 w2237 w2259 w2278 w2297 w2316 w2358 w2417 w2445 w2476 w2487 w2532 w2557 w2585 w2604 w2633 w2660 w2678 w2695 w2723 w2765 w2786 w2816 w2841 w2866 w2879 w2900 w2921 w2942 w2966 w2980 w3007 w3035 w3054 w3080 w3099 w3118 w3137 w3156 w3175 w3194 w3213] -> w1153
            tunnel: w1152 -> [w1190 w1209 w1228 w1257 w1314 w1403 w1463 w1527 w1571 w1599 w1659 w1685 w1705 w1731 w1739 w1796 w1829 w1841 w1867 w1896 w1934 w1953 w1994 w2024 w2045 w2065 w2084 w2103 w2147 w2163 w2207 w2238 w2260 w2279 w2298 w2317 w2357 w2418 w2446 w2471 w2505 w2533 w2556 w2586 w2605 w2630 w2659 w2679 w2703 w2722 w2766 w2793 w2817 w2840 w2865 w2880 w2901 w2922 w2943 w2967 w2993 w3013 w3041 w3052 w3085 w3104 w3123 w3142 w3161 w3180 w3199 w3218]
            tunnel: [w1190 w1209 w1228 w1257 w1314 w1403 w1464 w1528 w1572 w1599 w1659 w1685 w1705 w1731 w1739 w1796 w1829 w1841 w1867 w1896 w1934 w1953 w1994 w2024 w2045 w2065 w2084 w2103 w2147 w2163 w2207 w2238 w2260 w2279 w2298 w2317 w2357 w2418 w2446 w2471 w2505 w2533 w2556 w2586 w2605 w2630 w2659 w2679 w2703 w2722 w2766 w2793 w2817 w2840 w2865 w2880 w2901 w2922 w2943 w2967 w2993 w3013 w3041 w3052 w3085 w3104 w3123 w3142 w3161 w3180 w3199 w3218] -> w1151
            tunnel: [_ _ _ _ _ _ _ _ _ _ _ _ _ _ _ _ _ _ _ _ _ _ _ _ _ _ _ _ _ _ _ _ _ _ _ _ _ _ _ _ _ _ _ _ _ _ _ _ _ _ _ _ TRUE _ _ _ _ _ _ _ _ _ _ _ _ _ _ _ _ _ _ _] -> w1148
            tunnel: w1138 -> [w1187 w1206 w1225 w1248 w1308 w1391 w1450 w1514 w1543 _ w1649 w1680 w1704 w1729 w1759 w1794 w1827 w1852 w1878 w1907 w1933 w1970 w1991 w2022 w2043 w2062 w2081 w2100 w2146 w2180 w2205 w2236 w2257 w2276 w2295 w2314 w2356 w2416 w2435 w2467 w2503 w2531 w2554 w2584 w2603 w2628 w2658 w2677 w2701 w2727 w2764 w2790 w2814 w2832 w2859 w2877 w2898 w2919 w2940 w2964 w2991 w3011 w3039 w3058 w3084 w3103 w3122 w3141 w3160 w3179 w3198 w3217]
            tunnel: w1137 -> [w1186 w1205 w1224 w1247 w1307 w1390 w1449 w1513 w1544 _ w1648 w1679 w1703 w1728 w1758 w1793 w1826 w1851 w1877 w1906 w1932 w1969 w1990 w2021 w2042 w2061 w2080 w2099 w2145 w2179 w2204 w2235 w2256 w2275 w2294 w2313 w2355 w2415 w2434 w2466 w2502 w2530 w2553 w2583 w2602 w2627 w2657 w2676 w2700 w2726 w2763 w2789 w2813 w2831 w2858 w2876 w2897 w2918 w2939 w2963 w2990 w3010 w3038 w3057 w3083 w3102 w3121 w3140 w3159 w3178 w3197 w3216]
            tunnel: w1136 -> [w1185 w1204 w1223 w1246 w1306 w1389 w1448 w1512 w1545 _ w1647 w1678 w1702 w1727 w1757 w1792 w1825 w1850 w1876 w1905 w1931 w1968 w1989 w2020 w2041 w2060 w2079 w2098 w2144 w2178 w2203 w2234 w2255 w2274 w2293 w2312 w2354 w2414 w2433 w2465 w2501 w2529 w2552 w2582 w2601 w2626 w2656 w2675 w2699 w2725 w2762 w2788 w2812 w2830 w2857 w2875 w2896 w2917 w2938 w2962 w2989 w3009 w3037 w3056 w3082 w3101 w3120 w3139 w3158 w3177 w3196 w3215]
            tunnel: w1135 -> [w1184 w1203 w1222 w1245 w1305 w1388 w1447 w1511 w1546 _ w1646 w1677 w1701 w1726 w1756 w1791 w1824 w1849 w1875 w1904 w1930 w1967 w1988 w2019 w2040 w2059 w2078 w2097 w2143 w2177 w2202 w2233 w2254 w2273 w2292 w2311 w2353 w2413 w2432 w2464 w2500 w2528 w2551 w2581 w2600 w2625 w2655 w2674 w2698 w2724 w2761 w2787 w2811 w2829 w2856 w2874 w2895 w2916 w2937 w2961 w2988 w3008 w3036 w3055 w3081 w3100 w3119 w3138 w3157 w3176 w3195 w3214]
            tunnel: w1134 -> [_ _ _ _ _ _ _ _ _ _ _ _ _ _ _ _ _ _ _ _ _ _ _ _ _ _ _ _ _ w2182 _ _ _ _ _ _ _ _ _ _ _ _ _ _ _ _ _ _ _ _ _ _ _ _ _ _ _ _ _ _ _ _ _ _ _ _ _ _ _ _ _ _]
            tunnel: w1133 -> [_ _ _ _ _ _ _ _ _ _ _ _ _ _ _ _ _ _ _ _ _ _ _ _ _ _ _ _ _ w2181 _ _ _ _ _ _ _ _ _ _ _ _ _ _ _ _ _ _ _ _ _ _ _ _ _ _ _ _ _ _ _ _ _ _ _ _ _ _ _ _ _ _]
            tunnel: [w1187 w1206 w1225 w1248 w1308 w1391 w1450 w1514 w1543 w1592 w1649 w1680 w1704 w1729 w1759 w1794 w1827 w1852 w1878 w1907 w1933 w1970 w1991 w2022 w2043 w2062 w2081 w2100 w2146 w2180 w2205 w2236 w2257 w2276 w2295 w2314 w2356 w2416 w2435 w2467 w2503 w2531 w2554 w2584 w2603 w2628 w2658 w2677 w2701 w2727 w2764 w2790 w2814 w2832 w2859 w2877 w2898 w2919 w2940 w2964 w2991 w3011 w3039 w3058 w3084 w3103 w3122 w3141 w3160 w3179 w3198 w3217] -> w1130
            tunnel: [w1186 w1205 w1224 w1247 w1307 w1390 w1449 w1513 w1544 w1583 w1648 w1679 w1703 w1728 w1758 w1793 w1826 w1851 w1877 w1906 w1932 w1969 w1990 w2021 w2042 w2061 w2080 w2099 w2145 w2179 w2204 w2235 w2256 w2275 w2294 w2313 w2355 w2415 w2434 w2466 w2502 w2530 w2553 w2583 w2602 w2627 w2657 w2676 w2700 w2726 w2763 w2789 w2813 w2831 w2858 w2876 w2897 w2918 w2939 w2963 w2990 w3010 w3038 w3057 w3083 w3102 w3121 w3140 w3159 w3178 w3197 w3216] -> w1098
            tunnel: [w1185 w1204 w1223 w1246 w1306 w1389 w1448 w1512 w1545 w1591 w1647 w1678 w1702 w1727 w1757 w1792 w1825 w1850 w1876 w1905 w1931 w1968 w1989 w2020 w2041 w2060 w2079 w2098 w2144 w2178 w2203 w2234 w2255 w2274 w2293 w2312 w2354 w2414 w2433 w2465 w2501 w2529 w2552 w2582 w2601 w2626 w2656 w2675 w2699 w2725 w2762 w2788 w2812 w2830 w2857 w2875 w2896 w2917 w2938 w2962 w2989 w3009 w3037 w3056 w3082 w3101 w3120 w3139 w3158 w3177 w3196 w3215] -> w1131
            tunnel: [w1184 w1203 w1222 w1245 w1305 w1388 w1447 w1511 w1546 w1581 w1646 w1677 w1701 w1726 w1756 w1791 w1824 w1849 w1875 w1904 w1930 w1967 w1988 w2019 w2040 w2059 w2078 w2097 w2143 w2177 w2202 w2233 w2254 w2273 w2292 w2311 w2353 w2413 w2432 w2464 w2500 w2528 w2551 w2581 w2600 w2625 w2655 w2674 w2698 w2724 w2761 w2787 w2811 w2829 w2856 w2874 w2895 w2916 w2937 w2961 w2988 w3008 w3036 w3055 w3081 w3100 w3119 w3138 w3157 w3176 w3195 w3214] -> w1132
            tunnel: [_ _ _ _ _ _ _ _ _ _ _ _ _ _ _ _ _ _ _ _ _ _ _ _ _ _ _ _ w2133 w2182 _ _ _ _ _ _ _ _ _ _ _ _ _ _ _ _ _ _ _ _ _ _ _ _ _ _ _ _ _ _ _ _ _ _ _ _ _ _ _ _ _ _] -> w1100
            tunnel: [_ _ _ _ _ _ _ _ _ _ _ _ _ _ _ _ _ _ _ _ _ _ _ _ _ _ _ _ w2132 w2181 _ _ _ _ _ _ _ _ _ _ _ _ _ _ _ _ _ _ _ _ _ _ _ _ _ _ _ _ _ _ _ _ _ _ _ _ _ _ _ _ _ _] -> w1099
            tunnel: w1113 -> [w1183 w1202 w1221 w1244 w1304 w1387 w1446 w1510 w1542 w1590 w1656 w1676 w1700 w1725 w1742 w1784 w1810 w1835 w1863 w1892 w1929 w1966 w1987 w2018 w2039 w2058 w2077 w2096 w2131 w2176 w2201 w2232 w2253 w2272 w2291 w2310 w2352 w2412 w2429 w2463 w2499 w2527 w2548 w2575 w2599 w2622 w2649 w2673 w2692 w2720 w2754 w2785 w2810 w2842 w2867 w2878 w2899 w2920 w2941 w2965 w2992 w3012 w3040 w3059 w3075 w3097 w3116 w3135 w3154 w3173 w3192 w3211]
            tunnel: [w1183 w1202 w1221 w1244 w1304 w1387 w1446 w1510 w1542 w1590 w1656 w1676 w1700 w1725 w1741 w1783 w1803 w1834 w1862 w1891 w1929 w1966 w1987 w2018 w2039 w2058 w2077 w2096 w2131 w2176 w2201 w2232 w2253 w2272 w2291 w2310 w2352 w2412 w2429 w2463 w2499 w2527 w2548 w2575 w2599 w2622 w2649 w2673 w2692 w2719 w2754 w2785 w2810 w2842 w2867 w2878 w2899 w2920 w2941 w2965 w2992 w3012 w3040 w3059 w3075 w3097 w3116 w3135 w3154 w3173 w3192 w3211] -> w1112
            tunnel: [w1182 w1201 w1220 w1243 w1303 w1386 w1445 w1509 w1541 w1589 w1655 w1675 w1711 w1724 w1762 w1790 w1823 w1848 w1874 w1903 w1928 w1965 w1986 w2017 w2038 w2057 w2076 w2095 w2130 w2175 w2200 w2231 w2252 w2271 w2290 w2309 w2351 w2411 w2428 w2462 w2498 w2526 w2547 w2574 w2598 w2621 w2648 w2672 w2691 w2712 w2760 w2784 w2808 w2843 w2853 w2873 w2894 w2915 w2936 w2960 w2996 w3016 w3043 w3063 w3088 w3107 w3126 w3145 w3164 w3183 w3202 w3221] -> w1111
            tunnel: [w1181 w1200 w1219 w1242 w1302 w1385 w1444 w1508 w1540 w1588 w1654 w1674 w1710 w1723 w1761 w1789 w1822 w1847 w1873 w1902 w1927 w1964 w1985 w2016 w2037 w2056 w2075 w2094 w2129 w2174 w2199 w2230 w2251 w2270 w2289 w2308 w2350 w2410 w2427 w2461 w2497 w2525 w2546 w2573 w2597 w2620 w2647 w2671 w2690 w2711 w2759 w2783 w2809 w2825 w2850 w2883 w2904 w2925 w2946 w2968 w2995 w3015 w3042 w3062 w3087 w3106 w3125 w3144 w3163 w3182 w3201 w3220] -> w1110
            tunnel: w1109 -> [w1182 w1201 w1220 w1243 w1303 w1386 w1445 w1509 w1541 w1589 w1655 w1675 w1711 w1724 w1762 w1790 w1823 w1848 w1874 w1903 w1928 w1965 w1986 w2017 w2038 w2057 w2076 w2095 w2130 w2175 w2200 w2231 w2252 w2271 w2290 w2309 w2351 w2411 w2428 w2462 w2498 w2526 w2547 w2574 w2598 w2621 w2648 w2672 w2691 w2712 w2760 w2784 w2808 _ w2853 w2873 w2894 w2915 w2936 w2960 w2996 w3016 w3043 w3063 w3088 w3107 w3126 w3145 w3164 w3183 w3202 w3221]
            tunnel: w1108 -> [w1181 w1200 w1219 w1242 w1302 w1385 w1444 w1508 w1540 w1588 w1654 w1674 w1710 w1723 w1761 w1789 w1822 w1847 w1873 w1902 w1927 w1964 w1985 w2016 w2037 w2056 w2075 w2094 w2129 w2174 w2199 w2230 w2251 w2270 w2289 w2308 w2350 w2410 w2427 w2461 w2497 w2525 w2546 w2573 w2597 w2620 w2647 w2671 w2690 w2711 w2759 w2783 w2809 _ w2850 w2883 w2904 w2925 w2946 w2968 w2995 w3015 w3042 w3062 w3087 w3106 w3125 w3144 w3163 w3182 w3201 w3220]
            tunnel: w1107 -> [_ _ _ _ _ _ _ _ _ _ _ _ _ _ _ _ _ _ _ _ _ _ _ _ _ _ _ _ _ _ _ _ _ _ _ _ _ _ _ _ _ _ _ _ _ _ _ _ _ _ _ _ _ _ _ w2871 w2892 w2913 w2934 w2958 _ _ _ _ _ _ _ _ _ _ _ _]
            tunnel: w1105 -> [_ _ _ _ _ _ _ _ _ _ _ _ _ _ _ _ w1815 _ w1858 w1889 w1917 w1952 w1979 w2009 _ _ _ _ w2113 w2158 w2195 w2224 _ _ _ _ _ _ _ _ _ _ _ _ _ _ _ _ _ _ _ _ _ _ _ _ _ _ _ _ _ _ _ _ _ _ _ _ _ _ _ _]
            tunnel: w1102 -> [_ _ _ _ _ _ _ _ _ _ _ _ _ _ _ _ _ _ _ _ _ _ _ _ _ _ _ _ _ _ _ _ _ _ _ _ _ _ _ _ _ _ _ _ _ _ _ _ _ _ _ _ _ _ _ _ _ _ _ _ _ _ w3030 _ _ _ _ _ _ _ _ _]
            tunnel: [w1180 w1199 w1218 w1241 w1301 w1384 w1443 w1507 w1539 w1587 w1653 w1670 w1694 w1720 w1763 w1788 w1821 w1846 w1872 w1901 w1926 w1963 w1984 w2015 w2036 w2055 w2074 w2093 w2128 w2173 w2198 w2229 w2250 w2269 w2288 w2307 w2346 w2409 w2426 w2460 w2482 w2524 w2545 w2572 w2596 w2619 w2646 w2670 w2689 w2710 w2757 w2770 w2807 w2828 w2852 w2870 w2891 w2912 w2933 w2955 w2975 w3004 w3024 w3051 w3071 w3096 w3115 w3134 w3153 w3172 w3191 w3210] -> w1096
            tunnel: w1097 -> [w1180 w1199 w1218 w1241 w1301 w1384 w1443 w1507 w1539 w1587 w1653 w1670 _ w1720 w1763 w1788 w1821 w1846 w1872 w1901 w1926 w1963 w1984 w2015 w2036 w2055 w2074 w2093 w2128 w2173 w2198 w2229 w2250 w2269 w2288 w2307 w2346 w2409 w2426 w2460 w2482 w2524 w2545 w2572 w2596 w2619 w2646 w2670 w2689 w2710 w2757 w2771 w2807 w2828 w2852 w2870 w2891 w2912 w2933 w2955 w2975 w3004 w3024 w3051 w3071 w3096 w3115 w3134 w3153 w3172 w3191 w3210]
            tunnel: w1095 -> [w1179 w1198 w1217 w1240 w1300 w1383 w1442 w1506 w1538 w1586 w1652 w1669 w1693 w1719 w1755 w1787 w1820 w1845 w1871 w1900 w1925 w1962 w1983 w2014 w2035 w2054 w2073 w2092 w2127 w2172 w2197 w2228 w2249 w2268 w2287 w2306 w2345 w2408 w2425 w2459 w2496 w2523 w2544 w2571 w2595 w2618 w2645 w2669 w2688 w2709 w2756 w2782 w2806 w2827 w2855 w2869 w2890 w2911 w2932 w2954 w2974 w3003 w3023 w3050 w3070 w3095 w3114 w3133 w3152 w3171 w3190 w3209]
            tunnel: w1094 -> [w1178 w1197 w1216 w1239 w1299 w1382 w1441 w1505 w1537 w1585 w1651 w1668 w1692 w1718 w1754 w1786 w1819 w1844 w1870 w1899 w1924 w1961 w1982 w2013 w2034 w2053 w2072 w2091 w2126 w2171 w2196 w2227 w2248 w2267 w2286 w2305 w2344 w2407 w2424 w2458 w2493 w2522 w2543 w2570 w2594 w2617 w2644 w2668 w2687 w2708 w2755 w2781 w2805 w2826 w2854 w2868 w2889 w2910 w2931 w2953 w2973 w3002 w3022 w3049 w3069 w3094 w3113 w3132 w3151 w3170 w3189 w3208]
            tunnel: [w1179 w1198 w1217 w1240 w1300 w1383 w1442 w1506 w1538 w1586 w1652 w1669 w1693 w1719 w1755 w1787 w1820 w1845 w1871 w1900 w1925 w1962 w1983 w2014 w2035 w2054 w2073 w2092 w2127 w2172 w2197 w2228 w2249 w2268 w2287 w2306 w2345 w2408 w2425 w2459 w2495 w2523 w2544 w2571 w2595 w2618 w2645 w2669 w2688 w2709 w2756 w2782 w2806 w2827 w2855 w2869 w2890 w2911 w2932 w2954 w2974 w3003 w3023 w3050 w3070 w3095 w3114 w3133 w3152 w3171 w3190 w3209] -> w1093
            tunnel: [w1178 w1197 w1216 w1239 w1299 w1382 w1441 w1505 w1537 w1585 w1651 w1668 w1692 w1718 w1754 w1786 w1819 w1844 w1870 w1899 w1924 w1961 w1982 w2013 w2034 w2053 w2072 w2091 w2126 w2171 w2196 w2227 w2248 w2267 w2286 w2305 w2344 w2407 w2424 w2458 w2494 w2522 w2543 w2570 w2594 w2617 w2644 w2668 w2687 w2708 w2755 w2781 w2805 w2826 w2854 w2868 w2889 w2910 w2931 w2953 w2973 w3002 w3022 w3049 w3069 w3094 w3113 w3132 w3151 w3170 w3189 w3208] -> w1092
            tunnel: w1091 -> [_ _ _ _ _ _ _ _ _ _ w1644 _ _ _ w1766 w1776 _ _ _ _ _ _ _ _ _ _ _ _ _ w2168 _ _ _ _ _ _ w2342 w2406 _ _ _ _ _ _ _ w2616 _ _ _ _ w2732 _ _ _ _ _ _ _ _ _ _ _ _ _ _ _ _ _ _ _ _ _]
            tunnel: w1090 -> [_ _ _ _ _ _ _ _ _ _ w1645 _ _ _ w1765 w1775 _ _ _ _ _ _ _ _ _ _ _ _ _ w2167 _ _ _ _ _ _ w2343 w2405 _ _ _ _ _ _ _ w2615 _ _ _ _ w2731 _ _ _ _ _ _ _ _ _ _ _ _ _ _ _ _ _ _ _ _ _]
            tunnel: w1088 -> [_ _ _ _ _ _ _ _ _ _ _ _ _ _ _ _ w1814 _ w1857 w1888 w1916 w1951 w1978 w2010 _ _ _ _ w2112 w2157 w2194 w2223 _ _ _ _ _ _ _ _ _ _ _ _ _ _ _ _ _ _ _ _ _ _ _ _ _ _ _ _ _ _ _ _ _ _ _ _ _ _ _ _]
            tunnel: w1087 -> [_ _ _ _ _ _ _ _ _ _ _ _ _ _ _ _ w1813 _ _ w1885 w1919 w1956 w1981 w2011 _ _ _ _ w2118 w2162 w2193 w2226 _ _ _ _ _ _ _ _ _ _ _ _ _ _ _ _ _ _ _ _ _ _ _ _ _ _ _ _ _ _ _ _ _ _ _ _ _ _ _ _]
            tunnel: w1086 -> [_ _ _ _ _ _ _ _ _ _ _ _ _ _ _ _ w1812 _ _ w1884 w1918 w1955 w1980 w2012 _ _ _ _ w2117 w2161 w2192 w2225 _ _ _ _ _ _ _ _ _ _ _ _ _ _ _ _ _ _ _ _ _ _ _ _ _ _ _ _ _ _ _ _ _ _ _ _ _ _ _ _]
            tunnel: [_ _ _ _ _ _ _ _ _ _ _ _ _ _ _ _ w1813 _ w1860 w1885 w1919 w1956 w1981 w2011 _ _ _ _ w2118 w2162 w2193 w2226 _ _ _ _ _ _ _ _ _ _ _ _ _ _ _ _ _ _ _ _ _ _ _ _ _ _ _ _ _ _ _ _ _ _ _ _ _ _ _ _] -> w1085
            tunnel: [_ _ _ _ _ _ _ _ _ _ _ _ _ _ _ _ w1812 _ w1859 w1884 w1918 w1955 w1980 w2012 _ _ _ _ w2117 w2161 w2192 w2225 _ _ _ _ _ _ _ _ _ _ _ _ _ _ _ _ _ _ _ _ _ _ _ _ _ _ _ _ _ _ _ _ _ _ _ _ _ _ _ _] -> w1084
            tunnel: [_ _ _ _ _ _ _ _ _ _ _ _ _ _ _ _ w1815 w1838 w1858 w1889 w1917 w1952 w1979 w2009 _ _ _ _ w2113 w2158 w2195 w2224 _ _ _ _ _ _ _ _ _ _ _ _ _ _ _ _ _ _ _ _ _ _ _ _ _ _ _ _ _ _ _ _ _ _ _ _ _ _ _ _] -> w1083
            tunnel: [_ _ _ _ _ _ _ _ _ _ _ _ _ _ _ _ w1814 w1839 w1857 w1888 w1916 w1951 w1978 w2010 _ _ _ _ w2112 w2157 w2194 w2223 _ _ _ _ _ _ _ _ _ _ _ _ _ _ _ _ _ _ _ _ _ _ _ _ _ _ _ _ _ _ _ _ _ _ _ _ _ _ _ _] -> w1082
            tunnel: [_ _ _ _ _ _ _ _ _ _ _ _ _ _ _ _ _ _ _ _ _ w1950 _ _ _ _ _ _ _ w2159 _ _ _ _ _ _ w2325 w2384 _ _ _ _ _ _ _ _ _ _ _ _ _ _ _ _ _ _ _ _ _ _ _ _ _ _ _ _ _ _ _ _ _ _] -> w1079
            tunnel: [_ _ _ _ _ _ _ _ _ _ _ _ _ _ _ _ _ _ _ _ _ w1949 _ _ _ _ _ _ _ w2160 _ _ _ _ _ _ w2324 w2385 _ _ _ _ _ _ _ _ _ _ _ _ _ _ _ _ _ _ _ _ _ _ _ _ _ _ _ _ _ _ _ _ _ _] -> w1081
            tunnel: [_ _ _ _ _ _ _ _ _ _ _ _ _ _ _ _ _ _ w1856 w1887 _ _ _ _ _ _ _ _ _ _ _ _ _ _ _ _ _ _ _ _ _ _ _ _ _ _ _ _ _ _ _ _ _ _ _ _ _ _ _ _ _ _ _ _ _ _ _ _ _ _ _ _] -> w1076
            tunnel: [_ _ _ _ _ _ _ _ _ _ _ _ _ _ _ _ _ _ _ TRUE ("Recording") _ _ _ _ _ _ _ _ _ _ _ _ _ _ _ _ _ _ _ _ _ _ _ _ _ _ _ _ _ _ _ _ _ _ _ _ _ _ _ _ _ _ _ _ _ _ _ _ _ _ _ _] -> w1073
            tunnel: [_ _ _ _ _ _ _ _ _ _ _ _ _ _ _ _ _ _ w1856 _ _ _ _ _ _ _ _ _ _ _ _ _ _ _ _ _ _ _ _ _ _ _ _ _ _ _ _ _ _ _ _ _ _ _ _ _ _ _ _ _ _ _ _ _ _ _ _ _ _ _ _ _] -> w1069
            tunnel: [_ _ _ _ _ _ _ _ _ _ _ TRUE _ _ _ _ _ _ _ _ _ _ _ _ _ _ _ _ _ _ _ _ _ _ _ _ _ _ _ _ _ _ _ _ _ _ _ _ _ _ _ _ _ _ _ _ _ _ _ _ _ _ _ _ _ _ _ _ _ _ _ _] -> w1066
            tunnel: [_ _ _ _ _ _ _ _ _ _ _ w1665 _ _ _ _ _ _ _ _ _ _ _ _ _ _ _ _ _ _ _ _ _ _ _ _ _ _ _ _ _ _ _ _ _ _ _ _ _ _ _ _ _ _ _ _ _ _ _ _ _ _ _ _ _ _ _ _ _ _ _ _] -> w1064
            tunnel: [_ _ _ _ _ _ _ _ _ _ _ _ _ TRUE _ _ _ _ _ _ _ _ _ _ _ _ _ _ _ _ _ _ _ _ _ _ _ _ _ _ _ _ _ _ _ _ _ _ _ _ _ _ _ _ _ _ _ _ _ _ _ _ _ _ _ _ _ _ _ _ _ _] -> w1063
            tunnel: [_ _ _ _ _ _ _ _ _ _ _ _ _ w1712 _ _ _ _ _ _ _ _ _ _ _ _ _ _ _ _ _ _ _ _ _ _ _ _ _ _ _ _ _ _ _ _ _ _ _ _ _ _ _ _ _ _ _ _ _ _ _ _ _ _ _ _ _ _ _ _ _ _] -> w1062
            tunnel: w1047 -> [_ _ _ _ _ _ _ _ _ _ _ _ _ _ _ _ w1801 _ _ _ w1912 w1948 w1977 w2008 _ _ _ _ w2111 w2156 w2191 w2222 _ _ _ _ w2328 w2379 _ _ _ _ _ _ _ _ _ _ _ _ _ _ _ _ _ _ _ _ _ _ _ _ _ _ _ _ _ _ _ _ _ _]
            tunnel: [_ _ _ _ _ _ _ _ _ _ _ _ _ _ _ _ w1801 _ _ w1883 w1912 w1948 w1977 w2008 _ _ _ _ w2111 w2156 w2191 w2222 _ _ _ _ w2328 w2379 _ _ _ _ _ _ _ _ _ _ _ _ _ _ _ _ _ _ _ _ _ _ _ _ _ _ _ _ _ _ _ _ _ _] -> w1046
            tunnel: w1045 -> [_ _ _ _ _ _ _ _ _ _ _ _ _ _ _ _ w1800 _ _ _ w1911 w1947 w1976 w2007 _ _ _ _ w2110 w2155 w2190 w2221 _ _ _ _ w2326 w2383 _ _ _ _ _ _ _ _ _ _ _ _ _ _ _ _ _ _ _ _ _ _ _ _ _ _ _ _ _ _ _ _ _ _]
            tunnel: [_ _ _ _ _ _ _ _ _ _ _ _ _ _ _ _ w1800 _ _ w1882 w1911 w1947 w1976 w2007 _ _ _ _ w2110 w2155 w2190 w2221 _ _ _ _ w2326 w2383 _ _ _ _ _ _ _ _ _ _ _ _ _ _ _ _ _ _ _ _ _ _ _ _ _ _ _ _ _ _ _ _ _ _] -> w1044
            frame "Start1", Default {
            }
            frame "Start2" {
            }
            frame "Start3" {
            }
            frame "saveSettings1" {
              n603 = call "myRIO_BRig_RT_dataExp_Audio_freq__L.vi"() -> ("output_Audio_freq__L"=w1264:i32)  [unwired: 11 in]
              n604 = call "myRIO_BRig_RT_dataExp_Audio_freq__R.vi"() -> ("output_Audio_freq__R"=w1263:i32)  [unwired: 11 in]
              n605 = call "myRIO_BRig_RT_dataExp_Audio_amp__L.vi"() -> ("output_Audio_amp__L"=w1262:i32)  [unwired: 11 in]
              n606 = call "myRIO_BRig_RT_dataExp_Audio_amp__R.vi"() -> ("output_Audio_amp__R"=w1260:i32)  [unwired: 11 in]
              n607 = call "myRIO_BRig_RT_dataExp_TPB_min__L.vi"() -> ("output_TPB_min__L"=w1272:i32)  [unwired: 11 in]
              n608 = call "myRIO_BRig_RT_dataExp_TPB_min__R.vi"() -> ("output_TPB_min__R"=w1270:i32)  [unwired: 11 in]
              n609 = call "myRIO_BRig_RT_dataExp_TPB_max__L.vi"() -> ("output_TPB_max__L"=w1268:i32)  [unwired: 11 in]
              n610 = call "myRIO_BRig_RT_dataExp_TPB_max__R.vi"() -> ("output_TPB_max__R"=w1266:i32)  [unwired: 11 in]
              n611 = call "myRIO_BRig_RT_dataExp_ItrialUntilReward.vi"() -> ("output_I_trialUntilReward"=w1285:i32)  [unwired: 11 in]
              n612 = call "myRIO_BRig_RT_dataExp_IblockUntilReward.vi"() -> ("output_I_blockUntilReward"=w1281:i32)  [unwired: 11 in]
              n613 = call "myRIO_BRig_RT_dataExp_CueCycles.vi"() -> ("output_CueCycles"=w1280:i32)  [unwired: 11 in]
              n614 = call "myRIO_BRig_RT_dataExp_ENL_min.vi"() -> ("output_ENL_min"=w1278:i32)  [unwired: 11 in]
              n615 = call "myRIO_BRig_RT_dataExp_ENL_max.vi"() -> ("output_ENL_max"=w1276:i32)  [unwired: 11 in]
              n616 = call "myRIO_BRig_RT_dataExp_ENL_penalty.vi"() -> ("output_ENL_penalty"=w1274:i32)  [unwired: 11 in]
              n617 = local read "Audio_Freq__L"() -> (w1238:u8)
              n618 = local read "Audio_Freq__R"() -> (w1236:u8)
              n619 = local read "Audio_Amp__L"() -> (w1261:u16)
              n620 = local read "TpB_Min_L"() -> (w1271:u16)
              n621 = local read "TpB_Min_R"() -> (w1269:u16)
              n622 = local read "TpB_Max_L"() -> (w1267:u16)
              n623 = local read "TpB_Max_R"() -> (w1265:u16)
              n624 = local read "Audio_Amp__R"() -> (w1259:u16)
              n625 = local read "TrialUntilReward"() -> (w1284:bool)
              n626 = local read "CueCycles"() -> (w1279:u16)
              n627 = local read "Tcycle_ENL_min"() -> (w1277:u16)
              n628 = local read "Tcycle_ENL_max"() -> (w1275:u16)
              n629 = local read "Tcycle_ENLPenalty"() -> (w1273:u16)
              n630 = To Unsigned Word Integer(number=w1236) -> (unsigned 16bit integer=w1235:u16)
              n631 = To Unsigned Word Integer(number=w1238) -> (unsigned 16bit integer=w1237:u16)
              n632 = Boolean To (0,1)(Boolean=w1284) -> (0, 1=w1283:i16)
              n633 = To Unsigned Word Integer(number=w1283) -> (unsigned 16bit integer=w1282:u16)
              n634 = local read "BUR_min"() -> (w1253:u16)
              n635 = local read "BUR_max"() -> (w1254:u16)
              n636 = Not Equal To 0?(x=w1253) -> (x != 0?=w1252:bool)
              n637 = Not Equal To 0?(x=w1254) -> (x != 0?=w1251:bool)
              n638 = And(x=w1252, y=w1251) -> (x .and. y?=w1250:bool)
              n639 = Boolean To (0,1)(Boolean=w1250) -> (0, 1=w1255:i16)
              n640 = To Unsigned Word Integer(number=w1255) -> (unsigned 16bit integer=w1249:u16)
              n641 = Replace Array Subset(array=w1287, new element #1=w1282, index #1=w1285, new element #2=w1249, index #2=w1281, new element #3=w1279, index #3=w1280, new element #4=w1277, index #4=w1278, new element #5=w1275, index #5=w1276, new element #6=w1273, index #6=w1274, new element #7=w1271, index #7=w1272, new element #8=w1269, index #8=w1270, new element #9=w1267, index #9=w1268, new element #10=w1265, index #10=w1266, new element #11=w1237, index #11=w1264, new element #12=w1235, index #12=w1263, new element #13=w1261, index #13=w1262, new element #14=w1259, index #14=w1260) -> (w1286:u16[])
            }
            frame "saveSettings2" {
              n642 = call "myRIO_BRig_RT_dataExp_Tcycle_RewardPost.vi"() -> ("output_Tcycle_RewardPost"=w1324:i32)  [unwired: 11 in]
              n643 = call "myRIO_BRig_RT_dataExp_Tcycle_Wrong.vi"() -> ("output_Tcycle_Wrong"=w1322:i32)  [unwired: 11 in]
              n644 = call "myRIO_BRig_RT_dataExp_Tcycle_Timeout.vi"() -> ("output_Tcycle_Timeout"=w1320:i32)  [unwired: 11 in]
              n645 = call "myRIO_BRig_RT_dataExp_Tcycle_Cue_min.vi"() -> ("output_Tcycle_Cue_min"=w1318:i32)  [unwired: 11 in]
              n646 = call "myRIO_BRig_RT_dataExp_Tcycle_Cue_max.vi"() -> ("output_Tcycle_Cue_max"=w1317:i32)  [unwired: 11 in]
              n647 = call "myRIO_BRig_RT_dataExp_Tcycle_CuePenalty.vi"() -> ("output_Tcycle_CuePenalty"=w1316:i32)  [unwired: 11 in]
              n648 = call "myRIO_BRig_RT_dataExp_SolenoidProbability_L.vi"() -> ("output_SolenoidProbability_L"=w1296:i32)  [unwired: 11 in]
              n649 = call "myRIO_BRig_RT_dataExp_SolenoidProbability_R.vi"() -> ("output_SolenoidProbability_R"=w1295:i32)  [unwired: 11 in]
              n650 = call "myRIO_BRig_RT_dataExp_nBlock.vi"() -> ("output_nBlock"=w1333:i32)  [unwired: 11 in]
              n651 = call "myRIO_BRig_RT_dataExp_nTrial.vi"() -> ("output_nTrial"=w1332:i32)  [unwired: 11 in]
              n652 = call "myRIO_BRig_RT_dataExp_runTime_seconds.vi"() -> ("output_RunTime_minutes"=w1331:i32)  [unwired: 11 in]
              n653 = call "myRIO_BRig_RT_dataExp_Tcycle_Selection.vi"() -> ("output_Tcycle_Selection"=w1330:i32)  [unwired: 11 in]
              n654 = call "myRIO_BRig_RT_dataExp_Tcycle_Reward__L.vi"() -> ("output_Tcycle_Reward__L"=w1328:i32)  [unwired: 11 in]
              n655 = call "myRIO_BRig_RT_dataExp_Tcycle_Reward__R.vi"() -> ("output_Tcycle_Reward__R"=w1326:i32)  [unwired: 11 in]
              n656 = local read "Tcycle_RewardPost"() -> (w1323:u16)
              n657 = local read "Tcycle_Wrong"() -> (w1321:u16)
              n658 = local read "Tcycle_Timeout"() -> (w1319:u16)
              n659 = local read "Tcycle_CuePenalty"() -> (w1309:u16)
              n660 = local read "Tcycle_Cue_max"() -> (w1297:u16)
              n661 = local read "Tcycle_Cue_min"() -> (w1298:u16)
              n662 = local read "Tcycle_Selection"() -> (w1329:u16)
              n663 = local read "Tcycle_Reward_L"() -> (w1327:u16)
              n664 = local read "Tcycle_Reward_R"() -> (w1325:u16)
              n665 = local read "SolenoidProbability_R"() -> (w1293:u16)
              n666 = local read "SolenoidProbability_L"() -> (w1294:u16)
              n667 = Replace Array Subset(array=w1335, new element #1=u16 0, index #1=w1333, new element #2=u16 0, index #2=w1332, new element #3=u16 0, index #3=w1331, new element #4=w1329, index #4=w1330, new element #5=w1327, index #5=w1328, new element #6=w1325, index #6=w1326, new element #7=w1323, index #7=w1324, new element #8=w1321, index #8=w1322, new element #9=w1319, index #9=w1320, new element #10=w1298, index #10=w1318, new element #11=w1297, index #11=w1317, new element #12=w1309, index #12=w1316, new element #13=w1294, index #13=w1296, new element #14=w1293, index #14=w1295) -> (w1334:u16[])
            }
            frame "saveSettings3" {
              w1345 = 100.0 ("y")
              n668 = call "myRIO_BRig_RT_dataExp_laser_Freq.vi"() -> ("output_laser_Freq"=w1378:i32)  [unwired: 11 in]
              n669 = call "myRIO_BRig_RT_dataExp_laser_Tpeak.vi"() -> ("output_laser_Tpeak"=w1373:i32)  [unwired: 11 in]
              n670 = call "myRIO_BRig_RT_dataExp_laser_Tshutter.vi"() -> ("output_laser_Tshutter"=w1368:i32)  [unwired: 11 in]
              n671 = call "myRIO_BRig_RT_dataExp_laser_f_millisec2count.vi"() -> ("output_laser_f_millisec2count"=w1363:i32)  [unwired: 11 in]
              n672 = call "myRIO_BRig_RT_dataExp_laser_Power_min.vi"() -> ("output_laser_Power_min"=w1358:i32)  [unwired: 11 in]
              n673 = call "myRIO_BRig_RT_dataExp_laser_Power_max.vi"() -> ("output_laser_Power_max"=w1351:i32)  [unwired: 11 in]
              n674 = call "myRIO_BRig_RT_dataExp_laser_Power_step.vi"() -> ("output_laser_Power_step"=w1350:i32)  [unwired: 11 in]
              n675 = call "myRIO_BRig_RT_dataExp_laser_duration.vi"() -> ("output_laser_duration"=w1353:i32)  [unwired: 11 in]
              n676 = call "myRIO_BRig_RT_dataExp_BUR_min.vi"() -> ("output_BUR_min"=w1400:i32)  [unwired: 11 in]
              n677 = call "myRIO_BRig_RT_dataExp_BUR_max.vi"() -> ("output_BUR_max"=w1398:i32)  [unwired: 11 in]
              n678 = call "myRIO_BRig_RT_dataExp_Audio_sp__L.vi"() -> ("output_Audio_sp__L"=w1395:i32)  [unwired: 11 in]
              n679 = call "myRIO_BRig_RT_dataExp_Audio_sp__R.vi"() -> ("output_Audio_sp__R"=w1394:i32)  [unwired: 11 in]
              n680 = local read "laser_Tshutter"() -> (w1365:dbl)
              n681 = local read "f_millisec2count"() -> (w1360:dbl)
              n682 = local read "laser_Tpeak"() -> (w1370:dbl)
              n683 = local read "laser_power_min"() -> (w1355:dbl)
              n684 = local read "laser_power_max"() -> (w1344:dbl)
              n685 = local read "laser_power_step"() -> (w1343:dbl)
              n686 = local read "laser_Freq"() -> (w1377:dbl)
              n687 = local read "sp_LeftSpout"() -> (w1393:u16)
              n688 = local read "BUR_max"() -> (w1397:u16)
              n689 = local read "sp_RightSpout"() -> (w1392:u16)
              n690 = local read "BUR_min"() -> (w1399:u16)
              n691 = Multiply(x=w1377, y=w1345) -> (x*y=w1376:dbl)
              n692 = Multiply(x=w1370, y=w1345) -> (x*y=w1372:dbl)
              n693 = Multiply(x=w1365, y=w1345) -> (x*y=w1367:dbl)
              n694 = Multiply(x=w1360, y=w1345) -> (x*y=w1362:dbl)
              n695 = Multiply(x=w1355, y=w1345) -> (x*y=w1357:dbl)
              n696 = Multiply(x=w1344, y=w1345) -> (x*y=w1349:dbl)
              n697 = Multiply(x=w1343, y=w1345) -> (x*y=w1347:dbl)
              n698 = Round To Nearest(number=w1376) -> (nearest integer value=w1375:dbl)
              n699 = Round To Nearest(number=w1372) -> (nearest integer value=w1371:dbl)
              n700 = Round To Nearest(number=w1367) -> (nearest integer value=w1366:dbl)
              n701 = Round To Nearest(number=w1362) -> (nearest integer value=w1361:dbl)
              n702 = Round To Nearest(number=w1357) -> (nearest integer value=w1356:dbl)
              n703 = Round To Nearest(number=w1349) -> (nearest integer value=w1348:dbl)
              n704 = Round To Nearest(number=w1347) -> (nearest integer value=w1346:dbl)
              n705 = To Unsigned Word Integer(number=w1375) -> (unsigned 16bit integer=w1374:u16)
              n706 = To Unsigned Word Integer(number=w1371) -> (unsigned 16bit integer=w1369:u16)
              n707 = To Unsigned Word Integer(number=w1366) -> (unsigned 16bit integer=w1364:u16)
              n708 = To Unsigned Word Integer(number=w1361) -> (unsigned 16bit integer=w1359:u16)
              n709 = To Unsigned Word Integer(number=w1356) -> (unsigned 16bit integer=w1354:u16)
              n710 = To Unsigned Word Integer(number=w1348) -> (unsigned 16bit integer=w1342:u16)
              n711 = To Unsigned Word Integer(number=w1346) -> (unsigned 16bit integer=w1341:u16)
              n712 = local read "laser_duration"() -> (w1352:u16)
              n713 = call "myRIO_BRig_RT_dataCurrent_LaserPulse_duration.vi"() -> ("output_LaserPulse_duration"=w1379:i32)  [unwired: 11 in]
              n714 = Replace Array Subset(array=w1401, new element #1=w1399, index #1=w1400, new element #2=w1397, index #2=w1398, new element #3=w1393, index #3=w1395, new element #4=w1392, index #4=w1394, new element #5=w1374, index #5=w1378, new element #6=w1369, index #6=w1373, new element #7=w1364, index #7=w1368, new element #8=w1359, index #8=w1363, new element #9=w1354, index #9=w1358, new element #10=w1342, index #10=w1351, new element #11=w1341, index #11=w1350, new element #12=w1352, index #12=w1353) -> (w1396:u16[])
              n715 = Replace Array Subset(array=w1381, new element=w1352, index=w1379) -> (w1380:u16[])
            }
            frame "saveSettings4_LC_ENL" {
              # "Selection First"
              # "Count"
              # "Tdelay"
              # "Probability"
              # "OnOff"
              # "Block"
              # "delayOpt"
              # "Count"
              # "Tdelay"
              # "Probability"
              # "OnOff"
              # "Block"
              # "ENL1 All"
              # "delayOpt"
              # "Count"
              # "Tdelay"
              # "Probability"
              # "OnOff"
              # "Block"
              # "ENL1 First"
              n716 = call "myRIO_BRig_RT_dataLC_ENL1_All_Block.vi"() -> ("output_ENL1_All_Block"=w1436:i32)  [unwired: 11 in]
              n717 = call "myRIO_BRig_RT_dataLC_ENL1_All_OnOff.vi"() -> ("output_ENL1_All_OnOff"=w1426:i32)  [unwired: 11 in]
              n718 = call "myRIO_BRig_RT_dataLC_ENL1_All_Probability.vi"() -> ("output_ENL1_All_Probability"=w1425:i32)  [unwired: 11 in]
              n719 = call "myRIO_BRig_RT_dataLC_ENL1_All_Tdelay.vi"() -> ("output_ENL1_All_Tdelay"=w1424:i32)  [unwired: 11 in]
              n720 = call "myRIO_BRig_RT_dataLC_ENL1_All_Count.vi"() -> ("output_ENL1_All_Count"=w1423:i32)  [unwired: 11 in]
              n721 = call "myRIO_BRig_RT_dataLC_ENL1_All_delayOpt.vi"() -> ("output_ENL1_All_delayOpt"=w1422:i32)  [unwired: 11 in]
              n722 = call "myRIO_BRig_RT_dataLC_ENL1_First_Block.vi"() -> ("output_ENL1_First_Block"=w1462:i32)  [unwired: 11 in]
              n723 = call "myRIO_BRig_RT_dataLC_ENL1_First_OnOff.vi"() -> ("output_ENL1_First_OnOff"=w1460:i32)  [unwired: 11 in]
              n724 = call "myRIO_BRig_RT_dataLC_ENL1_First_Probability.vi"() -> ("output_ENL1_First_Probability"=w1456:i32)  [unwired: 11 in]
              n725 = call "myRIO_BRig_RT_dataLC_ENL1_First_Tdelay.vi"() -> ("output_ENL1_First_Tdelay"=w1454:i32)  [unwired: 11 in]
              n726 = call "myRIO_BRig_RT_dataLC_ENL1_First_Count.vi"() -> ("output_ENL1_First_Count"=w1452:i32)  [unwired: 11 in]
              n727 = call "myRIO_BRig_RT_dataLC_ENL1_First_delayOpt.vi"() -> ("output_ENL1_First_delayOpt"=w1438:i32)  [unwired: 11 in]
              n728 = local read "LC_ENL1_First_delayOpt"() -> (w1439:bool)
              n729 = local read "LC_ENL1_First_Count"() -> (w1451:u16)
              n730 = call "myRIO_BRig_RT_dataLC_Selection_First_Block.vi"() -> ("output_Selection_First_Block"=w1420:i32)  [unwired: 11 in]
              n731 = call "myRIO_BRig_RT_dataLC_Selection_First_OnOff.vi"() -> ("output_Selection_First_OnOff"=w1419:i32)  [unwired: 11 in]
              n732 = call "myRIO_BRig_RT_dataLC_Selection_First_Probability.vi"() -> ("output_Selection_First_Probability"=w1418:i32)  [unwired: 11 in]
              n733 = call "myRIO_BRig_RT_dataLC_Selection_First_Tdelay.vi"() -> ("output_Selection_First_Tdelay"=w1417:i32)  [unwired: 11 in]
              n734 = call "myRIO_BRig_RT_dataLC_Selection_First_Count.vi"() -> ("output_Selection_First_Count"=w1416:i32)  [unwired: 11 in]
              n735 = local read "LC_ENL1_First_Probability"() -> (w1455:u16)
              n736 = local read "LC_ENL1_First_Block"() -> (w1461:u16)
              n737 = local read "LC_ENL1_First_Tdelay"() -> (w1453:u16)
              n738 = local read "LC_ENL1_First_OnOff"() -> (w1459:bool)
              n739 = local read "LC_ENL1_All_OnOff"() -> (w1432:bool)
              n740 = local read "LC_ENL1_All_Probability"() -> (w1430:u16)
              n741 = local read "LC_ENL1_All_delayOpt"() -> (w1428:bool)
              n742 = local read "LC_ENL1_All_Tdelay"() -> (w1421:u16)
              n743 = local read "LC_ENL1_All_Block"() -> (w1433:u16)
              n744 = local read "LC_ENL1_All_Count"() -> (w1429:u16)
              n745 = local read "LC_Sel_First_Probability"() -> (w1411:u16)
              n746 = local read "LC_Sel_First_Tdelay"() -> (w1410:u16)
              n747 = local read "LC_Sel_First_OnOff"() -> (w1414:bool)
              n748 = local read "LC_Sel_First_Count"() -> (w1409:u16)
              n749 = local read "LC_Sel_First_Block"() -> (w1413:u16)
              n750 = Boolean To (0,1)(Boolean=w1439) -> (0, 1=w1440:i16)
              n751 = Boolean To (0,1)(Boolean=w1459) -> (0, 1=w1458:i16)
              n752 = Boolean To (0,1)(Boolean=w1432) -> (0, 1=w1435:i16)
              n753 = To Unsigned Word Integer(number=w1440) -> (unsigned 16bit integer=w1437:u16)
              n754 = To Unsigned Word Integer(number=w1458) -> (unsigned 16bit integer=w1457:u16)
              n755 = Boolean To (0,1)(Boolean=w1428) -> (0, 1=w1434:i16)
              n756 = To Unsigned Word Integer(number=w1435) -> (unsigned 16bit integer=w1431:u16)
              n757 = Boolean To (0,1)(Boolean=w1414) -> (0, 1=w1415:i16)
              n758 = To Unsigned Word Integer(number=w1434) -> (unsigned 16bit integer=w1427:u16)
              n759 = To Unsigned Word Integer(number=w1415) -> (unsigned 16bit integer=w1412:u16)
              n760 = Replace Array Subset(array=w1463, new element #1=w1461, index #1=w1462, new element #2=w1457, index #2=w1460, new element #3=w1455, index #3=w1456, new element #4=w1453, index #4=w1454, new element #5=w1451, index #5=w1452, new element #6=w1437, index #6=w1438, new element #7=w1433, index #7=w1436, new element #8=w1431, index #8=w1426, new element #9=w1430, index #9=w1425, new element #10=w1421, index #10=w1424, new element #11=w1429, index #11=w1423, new element #12=w1427, index #12=w1422, new element #13=w1413, index #13=w1420, new element #14=w1412, index #14=w1419, new element #15=w1411, index #15=w1418, new element #16=w1410, index #16=w1417, new element #17=w1409, index #17=w1416) -> (w1464:u16[])
            }
            frame "saveSettings5_LC_Cue" {
              # "Selection All"
              # "Count"
              # "Tdelay"
              # "Probability"
              # "OnOff"
              # "Block"
              # "delayOpt"
              # "Count"
              # "Tdelay"
              # "Probability"
              # "OnOff"
              # "Block"
              # "Cue1 All"
              # "delayOpt"
              # "Count"
              # "Tdelay"
              # "Probability"
              # "OnOff"
              # "Block"
              # "Cue1 First"
              n761 = call "myRIO_BRig_RT_dataLC_Cue1_First_delayOpt.vi"() -> ("output_Cue1_First_delayOpt"=w1503:i32)  [unwired: 11 in]
              n762 = call "myRIO_BRig_RT_dataLC_Cue1_First_Block.vi"() -> ("output_Cue1_First_Block"=w1526:i32)  [unwired: 11 in]
              n763 = call "myRIO_BRig_RT_dataLC_Cue1_First_OnOff.vi"() -> ("output_Cue1_First_OnOff"=w1524:i32)  [unwired: 11 in]
              n764 = call "myRIO_BRig_RT_dataLC_Cue1_First_Probability.vi"() -> ("output_Cue1_First_Probability"=w1520:i32)  [unwired: 11 in]
              n765 = call "myRIO_BRig_RT_dataLC_Cue1_First_Tdelay.vi"() -> ("output_Cue1_First_Tdelay"=w1518:i32)  [unwired: 11 in]
              n766 = call "myRIO_BRig_RT_dataLC_Cue1_First_Count.vi"() -> ("output_Cue1_First_Count"=w1516:i32)  [unwired: 11 in]
              n767 = call "myRIO_BRig_RT_dataLC_Cue1_All_Block.vi"() -> ("output_Cue1_All_Block"=w1500:i32)  [unwired: 11 in]
              n768 = call "myRIO_BRig_RT_dataLC_Cue1_All_OnOff.vi"() -> ("output_Cue1_All_OnOff"=w1499:i32)  [unwired: 11 in]
              n769 = call "myRIO_BRig_RT_dataLC_Cue1_All_Probability.vi"() -> ("output_Cue1_All_Probability"=w1498:i32)  [unwired: 11 in]
              n770 = call "myRIO_BRig_RT_dataLC_Cue1_All_Tdelay.vi"() -> ("output_Cue1_All_Tdelay"=w1497:i32)  [unwired: 11 in]
              n771 = call "myRIO_BRig_RT_dataLC_Cue1_All_Count.vi"() -> ("output_Cue1_All_Count"=w1496:i32)  [unwired: 11 in]
              n772 = call "myRIO_BRig_RT_dataLC_Cue1_All_delayOpt.vi"() -> ("output_Cue1_All_delayOpt"=w1495:i32)  [unwired: 11 in]
              n773 = local read "LC_Cue1_First_delayOpt"() -> (w1502:bool)
              n774 = local read "LC_Cue1_First_Count"() -> (w1515:u16)
              n775 = local read "LC_Cue1_First_Probability"() -> (w1519:u16)
              n776 = local read "LC_Cue1_First_Block"() -> (w1525:u16)
              n777 = local read "LC_Cue1_First_Tdelay"() -> (w1517:u16)
              n778 = local read "LC_Cue1_First_OnOff"() -> (w1523:bool)
              n779 = call "myRIO_BRig_RT_dataLC_Selection_All_Block.vi"() -> ("output_Selection_All_Block"=w1484:i32)  [unwired: 11 in]
              n780 = call "myRIO_BRig_RT_dataLC_Selection_All_OnOff.vi"() -> ("output_Selection_All_OnOff"=w1483:i32)  [unwired: 11 in]
              n781 = call "myRIO_BRig_RT_dataLC_Selection_All_Probability.vi"() -> ("output_Selection_All_Probability"=w1482:i32)  [unwired: 11 in]
              n782 = call "myRIO_BRig_RT_dataLC_Selection_All_Tdelay.vi"() -> ("output_Selection_All_Tdelay"=w1481:i32)  [unwired: 11 in]
              n783 = call "myRIO_BRig_RT_dataLC_Selection_All_Count.vi"() -> ("output_Selection_All_Count"=w1474:i32)  [unwired: 11 in]
              n784 = local read "LC_Cue1_All_OnOff"() -> (w1491:bool)
              n785 = local read "LC_Cue1_All_delayOpt"() -> (w1492:bool)
              n786 = local read "LC_Cue1_All_Probability"() -> (w1488:u16)
              n787 = local read "LC_Cue1_All_Tdelay"() -> (w1487:u16)
              n788 = local read "LC_Cue1_All_Count"() -> (w1486:u16)
              n789 = local read "LC_Cue1_All_Block"() -> (w1490:u16)
              n790 = local read "LC_Sel_All_Probability"() -> (w1476:u16)
              n791 = local read "LC_Sel_All_Tdelay"() -> (w1475:u16)
              n792 = local read "LC_Sel_All_OnOff"() -> (w1478:bool)
              n793 = local read "LC_Sel_All_Count"() -> (w1473:u16)
              n794 = local read "LC_Sel_All_Block"() -> (w1480:u16)
              n795 = Boolean To (0,1)(Boolean=w1502) -> (0, 1=w1504:i16)
              n796 = Boolean To (0,1)(Boolean=w1523) -> (0, 1=w1522:i16)
              n797 = Boolean To (0,1)(Boolean=w1491) -> (0, 1=w1494:i16)
              n798 = To Unsigned Word Integer(number=w1504) -> (unsigned 16bit integer=w1501:u16)
              n799 = To Unsigned Word Integer(number=w1522) -> (unsigned 16bit integer=w1521:u16)
              n800 = To Unsigned Word Integer(number=w1494) -> (unsigned 16bit integer=w1489:u16)
              n801 = Boolean To (0,1)(Boolean=w1492) -> (0, 1=w1493:i16)
              n802 = Boolean To (0,1)(Boolean=w1478) -> (0, 1=w1479:i16)
              n803 = To Unsigned Word Integer(number=w1493) -> (unsigned 16bit integer=w1485:u16)
              n804 = To Unsigned Word Integer(number=w1479) -> (unsigned 16bit integer=w1477:u16)
              n805 = Replace Array Subset(array=w1527, new element #1=w1525, index #1=w1526, new element #2=w1521, index #2=w1524, new element #3=w1519, index #3=w1520, new element #4=w1517, index #4=w1518, new element #5=w1515, index #5=w1516, new element #6=w1501, index #6=w1503, new element #7=w1490, index #7=w1500, new element #8=w1489, index #8=w1499, new element #9=w1488, index #9=w1498, new element #10=w1487, index #10=w1497, new element #11=w1486, index #11=w1496, new element #12=w1485, index #12=w1495, new element #13=w1480, index #13=w1484, new element #14=w1477, index #14=w1483, new element #15=w1476, index #15=w1482, new element #16=w1475, index #16=w1481, new element #17=w1473, index #17=w1474) -> (w1528:u16[])
            }
            frame "saveSettings6_LC_Other" {
              # "Trial"
              # "Tdelay"
              # "Probability"
              # "OnOff"
              # "Block"
              # "Wrong"
              # "Trial"
              # "Tdelay"
              # "Probability"
              # "OnOff"
              # "Block"
              # "Reward"
              n806 = call "myRIO_BRig_RT_dataLC_Wrong_Block.vi"() -> ("output_Wrong_Block"=w1558:i32)  [unwired: 11 in]
              n807 = call "myRIO_BRig_RT_dataLC_Wrong_OnOff.vi"() -> ("output_Wrong_OnOff"=w1557:i32)  [unwired: 11 in]
              n808 = call "myRIO_BRig_RT_dataLC_Wrong_Probability.vi"() -> ("output_Wrong_Probability"=w1556:i32)  [unwired: 11 in]
              n809 = call "myRIO_BRig_RT_dataLC_Wrong_Tdelay.vi"() -> ("output_Wrong_Tdelay"=w1555:i32)  [unwired: 11 in]
              n810 = call "myRIO_BRig_RT_dataLC_Wrong_Trial.vi"() -> ("output_Wrong_Trial"=w1554:i32)  [unwired: 11 in]
              n811 = call "myRIO_BRig_RT_dataLC_Reward_Block.vi"() -> ("output_Reward_Block"=w1570:i32)  [unwired: 11 in]
              n812 = call "myRIO_BRig_RT_dataLC_Reward_OnOff.vi"() -> ("output_Reward_OnOff"=w1568:i32)  [unwired: 11 in]
              n813 = call "myRIO_BRig_RT_dataLC_Reward_Probability.vi"() -> ("output_Reward_Probability"=w1564:i32)  [unwired: 11 in]
              n814 = call "myRIO_BRig_RT_dataLC_Reward_Tdelay.vi"() -> ("output_Reward_Tdelay"=w1562:i32)  [unwired: 11 in]
              n815 = call "myRIO_BRig_RT_dataLC_Reward_Trial.vi"() -> ("output_Reward_Trial"=w1560:i32)  [unwired: 11 in]
              n816 = local read "LC_Wrong_OnOff"() -> (w1552:bool)
              n817 = local read "LC_Wrong_Probability"() -> (w1549:u16)
              n818 = local read "LC_Wrong_Block"() -> (w1551:u16)
              n819 = local read "LC_Wrong_Tdelay"() -> (w1548:u16)
              n820 = local read "LC_Wrong_Trial"() -> (w1547:u16)
              n821 = local read "LC_Reward_Probability"() -> (w1563:u16)
              n822 = local read "LC_Reward_Block"() -> (w1569:u16)
              n823 = local read "LC_Reward_Tdelay"() -> (w1561:u16)
              n824 = local read "LC_Reward_OnOff"() -> (w1567:bool)
              n825 = local read "LC_Reward_Trial"() -> (w1559:u16)
              n826 = Boolean To (0,1)(Boolean=w1552) -> (0, 1=w1553:i16)
              n827 = Boolean To (0,1)(Boolean=w1567) -> (0, 1=w1566:i16)
              n828 = To Unsigned Word Integer(number=w1553) -> (unsigned 16bit integer=w1550:u16)
              n829 = To Unsigned Word Integer(number=w1566) -> (unsigned 16bit integer=w1565:u16)
              n830 = Replace Array Subset(array=w1571, new element #1=w1569, index #1=w1570, new element #2=w1565, index #2=w1568, new element #3=w1563, index #3=w1564, new element #4=w1561, index #4=w1562, new element #5=w1559, index #5=w1560, new element #6=w1551, index #6=w1558, new element #7=w1550, index #7=w1557, new element #8=w1549, index #8=w1556, new element #9=w1548, index #9=w1555, new element #10=w1547, index #10=w1554) -> (w1572:u16[])
            }
            frame "setSettings_Audio" {
              # "amp_L"
              # "amp_R"
              # "freq_L"
              # "freq_R"
              n831 = call "myRIO_BRig_RT_dataExp_Audio_amp__L.vi"() -> ("output_Audio_amp__L"=w1597:i32)  [unwired: 11 in]
              n832 = call "myRIO_BRig_RT_dataExp_Audio_amp__R.vi"() -> ("output_Audio_amp__R"=w1596:i32)  [unwired: 11 in]
              n833 = call "myRIO_BRig_RT_dataExp_Audio_freq__L.vi"() -> ("output_Audio_freq__L"=w1595:i32)  [unwired: 11 in]
              n834 = call "myRIO_BRig_RT_dataExp_Audio_freq__R.vi"() -> ("output_Audio_freq__R"=w1594:i32)  [unwired: 11 in]
              n835 = Index Array(array=w1593, index #1=w1597, index #2=w1596, index #3=w1595, index #4=w1594) -> (element #1=w1592:u16, element #2=w1591:u16, element #3=w1584:u16, element #4=w1582:u16)
              n836 = To Unsigned Byte Integer(number=w1584) -> (unsigned 8bit integer=w1583:u8)
              n837 = To Unsigned Byte Integer(number=w1582) -> (unsigned 8bit integer=w1581:u8)
            }
            frame "setSettings_Laser" {
              (unwired) u32 0 ("tDelay_laser_rew")
              # "Wrong tDelay"
              # "Reward tDelay"
              n838 = call "myRIO_BRig_RT_dataLC_Reward_Tdelay.vi"() -> ("output_Reward_Tdelay"=w1624:i32)  [unwired: 11 in]
              n839 = call "myRIO_BRig_RT_dataLC_Wrong_Tdelay.vi"() -> ("output_Wrong_Tdelay"=w1625:i32)  [unwired: 11 in]
              n840 = Index Array(array=w1621, index #1=w1624, index #2=w1625) -> (element #1=w1623:u16, element #2=w1622:u16)
              n841 = call "myRIO_BRig_RT__calc_Tvalley.vi"("input_peakWidth"="laser_Tpeak", "input_freq"="laser_Freq") -> ("output_Tvalley"=w1631:dbl)  [unwired: 9 in]
              n842 = To Double Precision Float(number=w1623) -> (double precision float=w1618:dbl)
              n843 = To Double Precision Float(number=w1622) -> (double precision float=w1615:dbl)
              n844 = Multiply(x="f_millisec2count", y="laser_Tpeak") -> (x*y=w1640:dbl)
              n845 = Multiply(x="f_millisec2count", y=w1631) -> (x*y=w1637:dbl)
              n846 = Multiply(x="f_millisec2count", y="laser_Tshutter") -> (x*y=w1635:dbl)
              n847 = Round Toward +Infinity(x="laser_Tshutter") -> (ceil(x): smallest int >= x=w1626:dbl)
              n848 = Multiply(x="f_millisec2count", y=w1618) -> (x*y=w1619:dbl)
              n849 = Multiply(x="f_millisec2count", y=w1615) -> (x*y=w1616:dbl)
              n850 = To Unsigned Word Integer(number="f_millisec2count") -> (unsigned 16bit integer=w1606:u16)
              n851 = Round Toward +Infinity(x=w1640) -> (ceil(x): smallest int >= x=w1641:dbl)
              n852 = Round Toward +Infinity(x=w1637) -> (ceil(x): smallest int >= x=w1638:dbl)
              n853 = Round Toward +Infinity(x=w1635) -> (ceil(x): smallest int >= x=w1630:dbl)
              n854 = Round Toward +Infinity(x=w1619) -> (ceil(x): smallest int >= x=w1620:dbl)
              n855 = Round Toward +Infinity(x=w1616) -> (ceil(x): smallest int >= x=w1617:dbl)
              n856 = To Unsigned Long Integer(number=w1641) -> (unsigned 32bit integer=w1639:u32)
              n857 = To Unsigned Long Integer(number=w1638) -> (unsigned 32bit integer=w1636:u32)
              n858 = To Unsigned Long Integer(number=w1630) -> (unsigned 32bit integer=w1634:u32)
              n859 = To Unsigned Word Integer(number=w1626) -> (unsigned 16bit integer=w1629:u16)
              n860 = To Unsigned Long Integer(number=w1620) -> (unsigned 32bit integer=w1614:u32)
              n861 = To Unsigned Long Integer(number=w1617) -> (unsigned 32bit integer=w1613:u32)
              n862 = Add(x="laser_duration", y=w1629) -> (x+y=w1610:u16)
              n863 = To Double Precision Float(number=w1610) -> (double precision float=w1609:dbl)
              n864 = Multiply(x=w1609, y="f_millisec2count") -> (x*y=w1611:dbl)
              n865 = call "myRIO_BRig_RT_dataCurrent_LaserPulse_duration.vi"() -> ("output_LaserPulse_duration"=w1642:i32)  [unwired: 11 in]
              n866 = Round Toward +Infinity(x=w1611) -> (ceil(x): smallest int >= x=w1612:dbl)
              n867 = To Unsigned Long Integer(number=w1612) -> (unsigned 32bit integer=w1608:u32)
              n868 = xnode "Read/Write Control"("FPGA VI Reference In"=w1644, "error in"=w1645, "laser_Npeak"=w1639, "laser_Nvalley"=w1636, "laser_Nshutter"=w1634, "laser_selRew_Ndelay"=w1614, "laser_selWro_NDelay"=w1613, "laser_selRew_Ntotal"=w1608, "laser_selWro_Ntotal"=w1608, "k1__counter_per_ms"=w1606) -> ("error out"=→"error out":errorcluster)  [unwired: 1 out]
              n869 = Replace Array Subset(array=w1621, new element=w1610, index=w1642) -> (w1643:u16[])
            }
            frame "initBlock" {
              n870 = call "myRIO_Brig_RT__Case_Exp_State_initBlock.vi"("input_spout"=w1689, "input_dataExp"=w1687, "input_dataCurrent"=w1688) -> ("output_spout"=w1667:enum16{"Left", "Right"}, "output_state"=w1690:T2, "output_dataExp"=w1686:u16[], "output_dataCurrent"=w1672:u16[], "output_TpB_target"=→"TpB_target":u16)  [unwired: 4 in]
              "cSpout" <- w1667
              n871 = call "myRIO_BRig_RT_dataCurrent_iBlock.vi"() -> ("output_iBlock"=w1671:i32)  [unwired: 11 in]
              n872 = Index Array(array=w1672, index=w1671) -> (element=w1665:u16)
              "iBlock" <- w1665
            }
            frame "initBlock2" {
              n873 = local write "nRewards_cur"(u16 0 ("nRewards_cur")) -> ()
              n874 = call "myRIO_BRig_RT__Case_Exp_State_initBlock2.vi"("input_spout"=w1698, "input_dataBlock"=w1699, "input_dataCurrent"=w1697) -> ("idxDataBlock"=w1694:i32, "output_dataBlock"=w1696:u16[][])  [unwired: 7 in]
            }
            frame "initTrial" {
              n875 = call "myRIO_Brig_RT__Case_Exp_State_initTrial.vi"("input_spout"=w1717, "input_dataExp"=w1733, "input_dataCurrent"=w1734) -> ("output_state"=w1735:T2, "output_dataExp"=w1732:u16[], "output_dataCurrent"=w1722:u16[])  [unwired: 6 in]
              n876 = call "myRIO_BRig_RT_dataCurrent_iTrial.vi"() -> ("output_iTrial"=w1721:i32)  [unwired: 11 in]
              n877 = call "myRIO_BRig_RT_dataCurrent_SolenoidReward.vi"() -> ("output_SolenoidReward"=w1716:i32)  [unwired: 11 in]
              n878 = Index Array(array=w1722, index #1=w1721, index #2=w1716) -> (element #1=w1712:u16, element #2=w1715:u16)
              "iTrial" <- w1712
              n879 = Not Equal To 0?(x=w1715) -> (x != 0?=→"SolenoidReward":bool)
            }
            frame "initTrial2" {
              # "trialUntilReward"
              n880 = call "myRIO_BRig_RT__Case_Exp_subState_LC__initTrial.vi"("input_dataTrial"=w1742, "input_spout"=w1751, "input_dataCurrent"=w1740, "input_dataLC"=w1739) -> ("output_LC_Wrong"=w1752:bool, "output_LC_led_Wrong"=w1744:bool, "output_LC_Reward"=w1753:bool, "output_LC_led_Reward"=w1743:bool, "output_dataTrial"=w1741:u16[][])  [unwired: 2 in]
              n881 = Equal?(x=w1751, y=enum16{"Left", "Right"}."Right") -> (x = y?=w1749:bool)
              n882 = call "myRIO_BRig_RT_dataExp_ItrialUntilReward.vi"() -> ("output_I_trialUntilReward"=w1747:i32)  [unwired: 11 in]
              n883 = Index Array(array=w1748, index=w1747) -> (element=w1746:u16)
              n884 = Not Equal To 0?(x=w1746) -> (x != 0?=w1745:bool)
              n885 = xnode "Read/Write Control"("FPGA VI Reference In"=w1766, "error in"=w1765, "SelectionState"=FALSE, "laserResponse_reward"=w1753, "laserResponse_wrong"=w1752, "laserResponse_reward_LED"=w1743, "laserResponse_wrong_LED"=w1744, "Left(F)_or_Right(T)"=w1749, "ignoreWrong"=w1745) -> ("error out"=→"error_initTrial":errorcluster)  [unwired: 1 out]
            }
            frame "initTrial3" {
              n886 = call "myRIO_BRig_RT__Case_Exp_State_initTrial_dataTrial.vi"("input_spout"=w1781, "input_dataCurrent"=w1782, "input_dataExp"=w1780, "input_dataTrial"=w1784) -> ("output_dataTrial"=w1783:u16[][], "output_laserPower"=w1777:u16)  [unwired: 6 in]
              n887 = To Double Precision Float(number=w1777) -> (double precision float=w1779:dbl)
              n888 = Divide(x=w1779, y=100.0 ("x")) -> (x/y=w1773:dbl)
              "output_PortA" <- w1773
              n889 = call "myRIO__convert__Voltage_to_FPGAvalue.vi"("input_voltage"=w1773) -> ("output_PortC"=w1772:i16)  [unwired: 9 in, 1 out]
              n890 = xnode "Read/Write Control"("FPGA VI Reference In"=w1776, "error in"=w1775, "AnaOut_0"=w1772) -> ("error out"=→"error out 4":errorcluster)  [unwired: 1 out]
            }
            frame "initTrial4" {
              n891 = call "myRIO_BRig_RT_dataCurrent_idxDataTrial.vi"() -> ("output_idxDataTrial"=w1809:i32)  [unwired: 11 in]
              n892 = call "myRIO_BRig_RT_dataTrial_activeRecording.vi"() -> ("output_activeRecording"=w1806:i32)  [unwired: 11 in]
              n893 = Index Array(array=w1811, index=w1809) -> (element=w1808:u16)
              n894 = Boolean To (0,1)(Boolean="Recording") -> (0, 1=w1805:i16)
              n895 = To Long Integer(number=w1808) -> (32bit integer=w1807:i32)
              n896 = To Unsigned Word Integer(number=w1805) -> (unsigned 16bit integer=w1804:u16)
              n897 = Replace Array Subset(array=w1810, new element=w1804, index (row)=w1807, index (col)=w1806) -> (w1803:u16[][])
            }
            frame "initTrial_LC_ENL1" {
              n898 = call "myRIO_BRig_RT__Case_Exp_State_initTrial_LC_ENL1__v2.vi"("input_dataTrial"=w1835, "input_spout"=w1840, "input_dataBlock"=w1833, "input_dataLC"=w1841, "input_dataCurrent"=w1837) -> ("output_LC__ENL1"=w1839:bool, "output_LC_led__ENL1"=w1838:bool, "output_dataTrial"=w1834:u16[][], "output_dataCurrent"=w1836:u16[])  [unwired: 3 in]
            }
            frame "initTrial_LC_Cue1" {
              w1856 = TRUE ("Recording")
              n899 = call "myRIO_BRig_RT__Case_Exp_State_initTrial_LC_Cue1__v2.vi"("input_dataTrial"=w1863, "input_spout"=w1866, "input_dataBlock"=w1861, "input_dataLC"=w1867, "input_dataCurrent"=w1865) -> ("output_LC__Cue1"=w1859:bool, "output_LC_led__Cue1"=w1860:bool, "output_dataTrial"=w1862:u16[][], "output_dataCurrent"=w1864:u16[])  [unwired: 3 in]
            }
            frame "initTrial_LC_Sel" {
              n900 = call "myRIO_BRig_RT__Case_Exp_State_initTrial_LC_Sel__v2.vi"("input_dataTrial"=w1892, "input_spout"=w1895, "input_dataBlock"=w1890, "input_dataLC"=w1896, "input_dataCurrent"=w1894) -> ("output_LC__Sel"=w1882:bool, "output_LC_led__Sel"=w1883:bool, "output_dataTrial"=w1891:u16[][], "output_dataCurrent"=w1893:u16[])  [unwired: 3 in]
              n901 = local read "Recording"() -> (w1887:bool)
            }
            frame "ENL1_pre" {
              # "ENL1_n"
              # "Tcycle"
              # "counter"
              n902 = call "myRIO_BRig_RT_dataCurrent_Tcycle_generic.vi"() -> ("output_Tcycle_generic"=w1942:i32)  [unwired: 11 in]
              n903 = call "myRIO_BRig_RT_dataCurrent_count_generic.vi"() -> ("output_count_generic"=w1944:i32)  [unwired: 11 in]
              n904 = call "myRIO_BRig_RT_dataCurrent_ENL.vi"() -> ("output_ENL"=w1941:i32)  [unwired: 11 in]
              n905 = call "myRIO_BRig_RT_dataCurrent_ENL1_n.vi"() -> ("output_ENL1_n"=w1915:i32)  [unwired: 11 in]
              n906 = Index Array(array=w1935, index #1=w1941, index #2=w1915) -> (element #1=w1940:u16, element #2=w1914:u16)
              n907 = Increment(x=w1914) -> (x+1=w1913:u16)
              n908 = Replace Array Subset(array=w1935, new element #1=u16 0 ("new element/subarray"), index #1=w1944, new element #2=w1940, index #2=w1942, new element #3=w1913, index #3=w1915) -> (w1939:u16[])
              n909 = Select(t=myRIO_BRig_RT__Case_Exp_stateList."ENL1Penalty_pre" ("Enum"), s=w1923, f=myRIO_BRig_RT__Case_Exp_stateList."ENL1" ("Enum")) -> (s? t:f=w1920:T2)
            }
            frame "ENL1" {
              n910 = call "myRIO_BRig_RT__Case_Exp_State_ENL1__v2.vi"("input_LC"=w1951, "I_lick"=w1954, "input_LC_led"=w1952, "input_state"=w1960, "input_dataCurrent"=w1959) -> ("output_trigger_laser_led"=w1950:bool, "output_state"=w1957:T2, "output_dataCurrent"=w1958:u16[], "output_trigger_laser"=w1949:bool)  [unwired: 3 in]
            }
            frame "ENL1Penalty_pre" {
              # "Tcycle"
              # "counter"
              n911 = call "myRIO_BRig_RT_dataCurrent_Tcycle_generic.vi"() -> ("output_Tcycle_generic"=w2000:i32)  [unwired: 11 in]
              n912 = call "myRIO_BRig_RT_dataCurrent_count_generic.vi"() -> ("output_count_generic"=w2002:i32)  [unwired: 11 in]
              n913 = call "myRIO_BRig_RT_dataExp_ENL_penalty.vi"() -> ("output_ENL_penalty"=w1995:i32)  [unwired: 11 in]
              n914 = Index Array(array=w1996, index=w1995) -> (element=w1999:u16)
              n915 = Replace Array Subset(array=w1997, new element #1=u16 0 ("new element/subarray"), index #1=w2002, new element #2=w1999, index #2=w2000) -> (w1998:u16[])
            }
            frame "ENL1Penalty" {
              n916 = call "myRIO_BRig_RT__Case_Exp_State_ENL1Penalty.vi"("input_state"=w2025, "input_dataCurrent"=w2029) -> ("output_state"=w2026:T2, "output_dataCurrent"=w2028:u16[])  [unwired: 8 in]
            }
            frame "ENL2_pre" {
            }
            frame "ENL2" {
            }
            frame "ENL2Penalty_pre" {
            }
            frame "ENL2Penalty" {
            }
            frame "Cue1_pre" {
              # "Cue1_n"
              # "Tcycle_Cue1"
              # "0 = L, 1 = R, 2 = both"
              # "sp_R"
              # "sp_L"
              # "Tcycle"
              # "counter"
              n917 = Equal?(x=w2140, y=enum16{"Left", "Right"}."Left") -> (x = y?=w2139:bool)
              n918 = call "myRIO_BRig_RT_dataExp_Audio_sp__L.vi"() -> ("output_Audio_sp__L"=w2138:i32)  [unwired: 11 in]
              n919 = call "myRIO_BRig_RT_dataExp_Audio_sp__R.vi"() -> ("output_Audio_sp__R"=w2137:i32)  [unwired: 11 in]
              n920 = call "myRIO_BRig_RT_dataCurrent_Tcycle_generic.vi"() -> ("output_Tcycle_generic"=w2150:i32)  [unwired: 11 in]
              n921 = call "myRIO_BRig_RT_dataCurrent_count_generic.vi"() -> ("output_count_generic"=w2152:i32)  [unwired: 11 in]
              n922 = Select(t=w2138, s=w2139, f=w2137) -> (s? t:f=w2136:i32)
              n923 = call "myRIO_BRig_RT_dataCurrent_Cue1_n.vi"() -> ("output_Cue1_n"=w2114:i32)  [unwired: 11 in]
              n924 = call "myRIO_BRig_RT_dataCurrent_Tcycle_cue.vi"() -> ("output_Tcycle_cue"=w2123:i32)  [unwired: 11 in]
              n925 = Index Array(array=w2142, index=w2136) -> (element=w2134:u16)
              n926 = Index Array(array=w2124, index #1=w2123, index #2=w2114) -> (element #1=w2125:u16, element #2=w2116:u16)
              n927 = Increment(x=w2116) -> (x+1=w2115:u16)
              n928 = Not Equal To 0?(x=w2134) -> (x != 0?=w2132:bool)
              n929 = Not Equal?(x=w2134, y=u16 1) -> (x != y?=w2133:bool)
              n930 = Replace Array Subset(array=w2124, new element #1=u16 0 ("new element/subarray"), index #1=w2152, new element #2=w2125, index #2=w2150, new element #3=w2115, index #3=w2114) -> (w2149:u16[])
              n931 = Select(t=myRIO_BRig_RT__Case_Exp_stateList."Cue1Penalty_pre" ("Enum"), s=w2120, f=myRIO_BRig_RT__Case_Exp_stateList."Cue1" ("Enum")) -> (s? t:f=w2121:T2)
            }
            frame "Cue1" {
              n932 = call "myRIO_BRig_RT__Case_Exp_State_Cue1__v2.vi"("input_LC"=w2161, "I_lick"=w2164, "input_LC_led"=w2162, "input_state"=w2166, "input_dataCurrent"=w2184) -> ("output_trigger_laser_led"=w2159:bool, "output_state"=w2165:T2, "output_dataCurrent"=w2183:u16[], "output_trigger_laser"=w2160:bool)  [unwired: 3 in]
              n933 = Equal?(x=myRIO_BRig_RT__Case_Exp_stateList."Selection_pre", y=w2165) -> (x = y?=w2169:bool)
              n934 = xnode "Read/Write Control"("FPGA VI Reference In"=w2168, "error in"=w2167, "SelectionState"=w2169) -> ()  [unwired: 2 out]
            }
            frame "Cue1Penalty_pre" {
              # "Tcycle"
              # "counter"
              n935 = call "myRIO_BRig_RT_dataCurrent_Tcycle_generic.vi"() -> ("output_Tcycle_generic"=w2215:i32)  [unwired: 11 in]
              n936 = call "myRIO_BRig_RT_dataCurrent_count_generic.vi"() -> ("output_count_generic"=w2217:i32)  [unwired: 11 in]
              n937 = call "myRIO_BRig_RT_dataExp_Tcycle_CuePenalty.vi"() -> ("output_Tcycle_CuePenalty"=w2214:i32)  [unwired: 11 in]
              n938 = Index Array(array=w2209, index=w2214) -> (element=w2213:u16)
              n939 = Replace Array Subset(array=w2211, new element #1=u16 0 ("new element/subarray"), index #1=w2217, new element #2=w2213, index #2=w2215) -> (w2210:u16[])
            }
            frame "Cue1Penalty" {
              # "reset laserOccurred"
              n940 = call "myRIO_BRig_RT__Case_Exp_State_Cue1Penalty.vi"("input_state"=w2243, "input_dataCurrent"=w2244) -> ("output_state"=w2241:T2, "output_dataCurrent"=w2242:u16[])  [unwired: 8 in]
            }
            frame "Cue2_pre" {
              n941 = call "myRIO_BRig_RT__Case_Exp_subState_LC__Cue2.vi"("input_spout"=w2261, "input_dataCurrent"=w2262, "input_dataLC"=w2260) -> ()  [unwired: 6 in, 2 out]
            }
            frame "Cue2" {
            }
            frame "Cue2Penalty_pre" {
            }
            frame "Cue2Penalty" {
            }
            frame "Selection_pre" {
              # "Tcycle"
              # "counter"
              n942 = call "myRIO_BRig_RT_dataCurrent_Sel_laserTiming_start.vi"() -> ("output_Sel_laserTiming_start"=w2332:i32)  [unwired: 11 in]
              n943 = xnode "Read/Write Control"("FPGA VI Reference In"=w2342, "error in"=w2343) -> ("error out"=→"error_Selection_pre":errorcluster, "SelectReward"=w2336:bool, "SelectWrong"=w2337:bool)  [unwired: 1 out]
              n944 = call "myRIO_BRig_RT_dataExp_Tcycle_Selection.vi"() -> ("output_Tcycle_Selection"=w2362:i32)  [unwired: 11 in]
              n945 = call "myRIO_BRig_RT_dataCurrent_Tcycle_generic.vi"() -> ("output_Tcycle_generic"=w2363:i32)  [unwired: 11 in]
              n946 = call "myRIO_BRig_RT_dataCurrent_count_generic.vi"() -> ("output_count_generic"=w2365:i32)  [unwired: 11 in]
              n947 = Index Array(array=w2333, index=w2332) -> (element=w2331:u16)
              n948 = Index Array(array=w2359, index=w2362) -> (element=w2361:u16)
              n949 = Equal To 0?(x=w2331) -> (x = 0?=w2329:bool)
              n950 = Replace Array Subset(array=w2333, new element #1=u16 0 ("new element/subarray"), index #1=w2365, new element #2=w2361, index #2=w2363) -> (w2360:u16[])
              n951 = Or(x=w2336, y=w2337) -> (x .or. y?=w2327:bool)
              n952 = Not(x=w2327) -> (.not. x?=w2330:bool)
              n953 = Compound Arithmetic op=AND(w2330, w2329, w2328) -> (w2325:bool)
              n954 = And(x=w2325, y=w2326) -> (x .and. y?=w2324:bool)
              n955 = Select(t=myRIO_BRig_RT__Case_Exp_stateList."SelectReward_pre" ("Enum"), s=w2336, f=myRIO_BRig_RT__Case_Exp_stateList."SelectWrong_pre" ("Enum")) -> (s? t:f=w2341:T2)
              n956 = Select(t=w2341, s=w2327, f=myRIO_BRig_RT__Case_Exp_stateList."Selection" ("Enum")) -> (s? t:f=w2338:T2)
            }
            frame "Selection" {
              # "counter\nSelection"
              # "increment"
              # "get Tcycle"
              # "get count"
              n957 = call "myRIO_BRig_RT_dataCurrent_Tcycle_generic.vi"() -> ("output_Tcycle_generic"=w2399:i32)  [unwired: 11 in]
              n958 = call "myRIO_BRig_RT_dataCurrent_count_generic.vi"() -> ("output_count_generic"=w2395:i32)  [unwired: 11 in]
              n959 = call "myRIO_BRig_RT_dataCurrent_Sel_laserTiming_start.vi"() -> ("output_Sel_laserTiming_start"=w2387:i32)  [unwired: 11 in]
              n960 = call "myRIO_BRig_RT_dataCurrent_Sel_laserTiming_end.vi"() -> ("output_Sel_laserTiming_end"=w2386:i32)  [unwired: 11 in]
              n961 = call "myRIO_BRig_RT__increment_u16.vi"() -> ("output_increment__u16"=w2373:u16)  [unwired: 11 in]
              n962 = xnode "Read/Write Control"("FPGA VI Reference In"=w2406, "error in"=w2405) -> ("error out"=→"error_Selection":errorcluster, "SelectReward"=w2402:bool, "SelectWrong"=w2403:bool)  [unwired: 1 out]
              n963 = call "myRIO_BRig_RT_dataCurrent_Sel_laserTriggered.vi"() -> ("output_Sel_laserTriggered"=w2374:i32)  [unwired: 11 in]
              n964 = Index Array(array=w2400, index #1=w2399, index #2=w2395, index #3=w2387, index #4=w2386, index #5=w2374) -> (element #1=w2394:u16, element #2=w2372:u16, element #3=w2371:u16, element #4=w2377:u16, element #5=w2368:u16)
              n965 = Increment(x=w2368) -> (x+1=w2369:u16)
              n966 = Equal?(x=w2372, y=w2371) -> (x = y?=w2370:bool)
              n967 = Add(x=w2372, y=w2373) -> (x+y=w2378:u16)
              n968 = Greater Or Equal?(x=w2378, y=w2371) -> (x >= y?=w2375:bool)
              n969 = Less Or Equal?(x=w2378, y=w2377) -> (x <= y?=w2376:bool)
              n970 = Greater?(x=w2394, y=w2378) -> (0:w2380:bool)
              n971 = Select(t=w2369, s=w2370, f=w2368) -> (s? t:f=w2367:u16)
              n972 = Select(t=myRIO_BRig_RT__Case_Exp_stateList."SelectReward_pre" ("Enum"), s=w2402, f=myRIO_BRig_RT__Case_Exp_stateList."SelectWrong_pre" ("Enum")) -> (s? t:f=w2401:T2)
              n973 = Or(x=w2402, y=w2403) -> (x .or. y?=w2381:bool)
              n974 = Not(x=w2381) -> (.not. x?=w2382:bool)
              n975 = Select(t=w2398, s=w2380, f=myRIO_BRig_RT__Case_Exp_stateList."SelectTimeout_pre" ("Enum")) -> (s? t:f=w2389:T2)
              n976 = Compound Arithmetic op=AND(w2380, w2382, w2375, w2376, w2379) -> (w2384:bool)
              n977 = Select(t=w2378, s=w2380, f=w2394) -> (s? t:f=w2392:u16)
              n978 = Select(t=w2401, s=w2381, f=w2389) -> (s? t:f=w2404:T2)
              n979 = And(x=w2384, y=w2383) -> (x .and. y?=w2385:bool)
              n980 = call "myRIO_BRig_RT_dataCurrent_count_selection.vi"() -> ("output_count_generic"=w2393:i32)  [unwired: 11 in]
              n981 = Replace Array Subset(array=w2400, new element #1=w2392, index #1=w2395, new element #2=w2392, index #2=w2393, new element #3=w2367, index #3=w2374) -> (w2397:u16[])
            }
            frame "SelectReward_pre" {
              # "iState"
              # "Tcycle\nReward"
              # "nRewTrials"
              # "Tcycle\nGeneric"
              # "counter"
              n982 = call "myRIO_BRig_RT_dataCurrent_nRewTrials.vi"() -> ("output_nRewTrials"=w2438:i32)  [unwired: 11 in]
              n983 = Equal?(x=w2447, y=enum16{"Left", "Right"}."Left") -> (x = y?=w2448:bool)
              n984 = Index Array(array=w2439, index=w2438) -> (element=w2437:u16)
              n985 = call "myRIO_BRig_RT_dataExp_Tcycle_Reward__L.vi"() -> ("output_Tcycle_Reward__L"=w2451:i32)  [unwired: 11 in]
              n986 = call "myRIO_BRig_RT_dataExp_Tcycle_Reward__R.vi"() -> ("output_Tcycle_Reward__R"=w2452:i32)  [unwired: 11 in]
              n987 = Increment(x=w2437) -> (x+1=w2436:u16)
              n988 = Select(t=w2451, s=w2448, f=w2452) -> (s? t:f=w2450:i32)
              n989 = call "myRIO_BRig_RT__Case_Exp_subState_LC__Reward.vi"("input_spout"=w2447, "input_dataCurrent"=w2439, "input_dataLC"=w2446) -> ()  [unwired: 6 in, 2 out]
              n990 = call "myRIO_BRig_RT_dataCurrent_count_generic.vi"() -> ("output_count_generic"=w2441:i32)  [unwired: 11 in]
              n991 = call "myRIO_BRig_RT_dataCurrent_Tcycle_generic.vi"() -> ("output_Tcycle_generic"=w2442:i32)  [unwired: 11 in]
              n992 = Index Array(array=w2453, index=w2450) -> (element=w2443:u16)
              n993 = call "myRIO_BRig_RT_dataCurrent_iState.vi"() -> ("output_iState"=w2431:i32)  [unwired: 11 in]
              n994 = Replace Array Subset(array=w2439, new element #1=w2436, index #1=w2438, new element #2=u16 0 ("new element/subarray"), index #2=w2441, new element #3=w2443, index #3=w2442, new element #4=u16 1 ("new element/subarray"), index #4=w2431) -> (w2454:u16[])
            }
            frame "SelectReward" {
              n995 = call "myRIO_BRig_RT__Case_Exp_State_Reward.vi"("input_dataCurrent"=w2475, "input_state"=w2472, "input_spout"=w2470) -> ("output_dataCurrent"=w2474:u16[], "output_state"=w2473:T2, "output__L"=w2468:bool, "output__R"=w2469:bool)  [unwired: 9 in]
            }
            frame "SelectRewardPost_pre" {
              # "nRewards"
              # "nRewTrials"
              # "Tcycle"
              # "counter"
              n996 = call "myRIO_BRig_RT_dataBlock_nRewards__L.vi"() -> ("output_nRewards__L"=w2491:i32)  [unwired: 11 in]
              n997 = call "myRIO_BRig_RT_dataBlock_nRewards__R.vi"() -> ("output_nRewards__R"=w2490:i32)  [unwired: 11 in]
              n998 = call "myRIO_BRig_RT_dataCurrent_Tcycle_generic.vi"() -> ("output_Tcycle_generic"=w2510:i32)  [unwired: 11 in]
              n999 = call "myRIO_BRig_RT_dataCurrent_count_generic.vi"() -> ("output_count_generic"=w2512:i32)  [unwired: 11 in]
              n1000 = case shown="\"Left\", Default" w2484 {
                tunnel: w2496 -> [w2517 w2521]
                tunnel: [w2516 w2521] -> w2495
                tunnel: [w2518 w2519] -> w2494
                tunnel: w2493 -> [w2518 w2520]
                frame "Left", Default {
                  n1001 = Increment(x=w2517) -> (x+1=w2516:u16)
                }
                frame "Right" {
                  n1002 = Increment(x=w2520) -> (x+1=w2519:u16)
                }
              }
              "nRewards_Left" <- w2495
              "nRewards_Right" <- w2494
              n1003 = Equal?(x=w2484, y=enum16{"Left", "Right"}."Left") -> (x = y?=w2483:bool)
              n1004 = Select(t=w2491, s=w2483, f=w2490) -> (s? t:f=w2489:i32)
              n1005 = call "myRIO_BRig_RT_dataExp_Tcycle_RewardPost.vi"() -> ("output_Tcycle_RewardPost"=w2506:i32)  [unwired: 11 in]
              n1006 = call "myRIO_BRig_RT_dataCurrent_nRewTrials.vi"() -> ("output_nRewTrials"=w2492:i32)  [unwired: 11 in]
              n1007 = Index Array(array=w2507, index=w2506) -> (element=w2509:u16)
              n1008 = Index Array(array=w2486, index=w2492) -> (element=w2481:u16)
              n1009 = Replace Array Subset(array=w2486, new element #1=u16 0 ("new element/subarray"), index #1=w2512, new element #2=w2509, index #2=w2510) -> (w2508:u16[])
              n1010 = Replace Array Subset(array=w2488, new element=w2481, index (row)=w2482, index (col)=w2489) -> (w2487:u16[][])
              n1011 = local write "nRewards_cur"(w2481) -> ()
            }
            frame "SelectRewardPost" {
              n1012 = call "myRIO_BRig_RT__Case_Exp_State_RewardPost.vi"("input_state"=w2536, "input_dataCurrent"=w2539) -> ("output_state"=w2537:T2, "output_dataCurrent"=w2538:u16[])  [unwired: 8 in]
            }
            frame "SelectWrong_pre" {
              # "iState"
              # "Tcycle"
              # "counter"
              n1013 = call "myRIO_BRig_RT_dataCurrent_Tcycle_generic.vi"() -> ("output_Tcycle_generic"=w2564:i32)  [unwired: 11 in]
              n1014 = call "myRIO_BRig_RT_dataCurrent_count_generic.vi"() -> ("output_count_generic"=w2566:i32)  [unwired: 11 in]
              n1015 = call "myRIO_BRig_RT_dataExp_Tcycle_Wrong.vi"() -> ("output_Tcycle_Wrong"=w2562:i32)  [unwired: 11 in]
              n1016 = call "myRIO_BRig_RT__Case_Exp_subState_LC__Wrong.vi"("input_spout"=w2558, "input_dataCurrent"=w2559, "input_dataLC"=w2556) -> ()  [unwired: 6 in, 2 out]
              n1017 = Index Array(array=w2560, index=w2562) -> (element=w2563:u16)
              n1018 = call "myRIO_BRig_RT_dataCurrent_iState.vi"() -> ("output_iState"=w2550:i32)  [unwired: 11 in]
              n1019 = Replace Array Subset(array=w2559, new element #1=u16 0 ("new element/subarray"), index #1=w2566, new element #2=w2563, index #2=w2564, new element #3=u16 2 ("new element/subarray"), index #3=w2550) -> (w2561:u16[])
            }
            frame "SelectWrong" {
              n1020 = call "myRIO_BRig_RT__Case_Exp_State_Wrong.vi"("input_state"=w2580, "input_dataCurrent"=w2589) -> ("output_state"=w2577:T2, "output_dataCurrent"=w2588:u16[])  [unwired: 8 in]
              n1021 = Not Equal?(x=w2580, y=w2577) -> (x != y?=w2579:bool)
              n1022 = Select(t=myRIO_BRig_RT__Case_Exp_stateList."SelectWrong_post" ("Enum"), s=w2579, f=w2577) -> (s? t:f=w2576:T2)
            }
            frame "SelectWrong_post" {
            }
            frame "SelectTimeout_pre" {
              # "iState"
              # "Tcycle"
              # "counter"
              n1023 = xnode "Read/Write Control"("FPGA VI Reference In"=w2616, "error in"=w2615, "SelectionState"=FALSE) -> ("error out"=→"error out 3":errorcluster)  [unwired: 1 out]
              n1024 = call "myRIO_BRig_RT_dataCurrent_Tcycle_generic.vi"() -> ("output_Tcycle_generic"=w2638:i32)  [unwired: 11 in]
              n1025 = call "myRIO_BRig_RT_dataCurrent_count_generic.vi"() -> ("output_count_generic"=w2636:i32)  [unwired: 11 in]
              n1026 = call "myRIO_BRig_RT_dataExp_Tcycle_Timeout.vi"() -> ("output_Tcycle_Timeout"=w2640:i32)  [unwired: 11 in]
              n1027 = call "myRIO_BRig_RT__Case_Exp_subState_LC__Timeout.vi"("input_spout"=w2631, "input_dataCurrent"=w2632, "input_dataLC"=w2630) -> ()  [unwired: 6 in, 2 out]
              n1028 = Index Array(array=w2634, index=w2640) -> (element=w2639:u16)
              n1029 = call "myRIO_BRig_RT_dataCurrent_iState.vi"() -> ("output_iState"=w2624:i32)  [unwired: 11 in]
              n1030 = Replace Array Subset(array=w2632, new element #1=u16 0 ("new element/subarray"), index #1=w2636, new element #2=w2639, index #2=w2638, new element #3=u16 3 ("new element/subarray"), index #3=w2624) -> (w2635:u16[])
            }
            frame "SelectTimeout" {
              n1031 = call "myRIO_BRig_RT__Case_Exp_State_Timeout.vi"("input_dataLC"=w2659, "input_state"=w2650, "input_dataCurrent"=w2664) -> ("output_state"=w2651:T2, "output_dataCurrent"=w2663:u16[])  [unwired: 6 in, 1 out]
              n1032 = Not Equal?(x=w2650, y=w2651) -> (x != y?=w2654:bool)
              n1033 = Select(t=myRIO_BRig_RT__Case_Exp_stateList."SelectTimeout_post" ("Enum"), s=w2654, f=w2651) -> (s? t:f=w2652:T2)
            }
            frame "SelectTimeout_post" {
            }
            frame "endTrial1" {
              # "Update dataBlock"
              n1034 = call "myRIO_BRig_RT__Case_Exp_State_endTrial1.vi"("input_spout"=w2697, "input_dataBlock"=w2696, "input_dataCurrent"=w2694) -> ("output_dataBlock"=w2695:u16[][], "output_dataCurrent"=w2693:u16[])  [unwired: 7 in]
            }
            frame "endTrial2" {
              # "update dataTrial"
              n1035 = call "myRIO_BRig_RT__Case_Exp_State_endTrial2.vi"("input_spout"=w2716, "input_dataTrial"=w2720, "input_dataCurrent"=w2718) -> ("output_dataTrial"=w2719:u16[][], "output_dataCurrent"=w2717:u16[])  [unwired: 7 in]
            }
            frame "endTrial3" {
              w2746 = myRIO_BRig_RT__Case_Exp_stateList."endBlock" ("Enum")
              # "nRewTrials"
              # "iTrial"
              # "I_blockUntilReward"
              # "TPB"
              # "end block?"
              n1036 = local read "STOP_endTrial"() -> (w2744:bool)
              n1037 = local read "STOP_abort"() -> (w2743:bool)
              n1038 = xnode "Read/Write Control"("FPGA VI Reference In"=w2732, "error in"=w2731, "SelectionState"=FALSE) -> ("error out"=→"error out 2":errorcluster)  [unwired: 1 out]
              n1039 = local read "START"() -> (w2741:bool)
              n1040 = call "myRIO_BRig_RT_dataExp_IblockUntilReward.vi"() -> ("output_I_blockUntilReward"=w2753:i32)  [unwired: 11 in]
              n1041 = Index Array(array=w2737, index=w2753) -> (element=w2733:u16)
              n1042 = Not(x=w2741) -> (.not. x?=w2742:bool)
              n1043 = Not Equal To 0?(x=w2733) -> (x != 0?=w2751:bool)
              n1044 = Compound Arithmetic op=OR(w2744, w2742, w2743) -> (w2745:bool)
              n1045 = call "myRIO_BRig_RT_dataCurrent_nRewTrials.vi"() -> ("output_nRewTrials"=w2749:i32)  [unwired: 11 in]
              n1046 = call "myRIO_BRig_RT_dataCurrent_iTrial.vi"() -> ("output_iTrial"=w2750:i32)  [unwired: 11 in]
              n1047 = Select(t=w2749, s=w2751, f=w2750) -> (s? t:f=w2748:i32)
              n1048 = call "myRIO_BRig_RT_dataCurrent_TpB.vi"() -> ("output_TpB"=w2752:i32)  [unwired: 11 in]
              n1049 = Index Array(array=w2738, index #1=w2752, index #2=w2748) -> (element #1=w2739:u16, element #2=w2740:u16)
              n1050 = Less Or Equal?(x=w2739, y=w2740) -> (x <= y?=w2736:bool)
              n1051 = Select(t=w2746, s=w2736, f=myRIO_BRig_RT__Case_Exp_stateList."empty_endTrial1" ("Enum")) -> (s? t:f=w2747:T2)
              n1052 = Select(t=w2746, s=w2745, f=w2747) -> (s? t:f=w2734:T2)
            }
            frame "endBlock" {
              # "R"
              # "L"
              # "idxDataBlock"
              n1053 = Equal?(x=w2777, y=enum16{"Left", "Right"}."Left") -> (x = y?=w2776:bool)
              n1054 = call "myRIO_BRig_RT_dataCurrent_idxDataBlockL.vi"() -> ("output_idxDataBlock__L"=w2780:i32)  [unwired: 11 in]
              n1055 = call "myRIO_BRig_RT_dataCurrent_idxDataBlockR.vi"() -> ("output_idxDataBlock__R"=w2779:i32)  [unwired: 11 in]
              n1056 = Increment(x=w2771) -> (x+1=w2770:i32)
              n1057 = Select(t=w2780, s=w2776, f=w2779) -> (s? t:f=w2774:i32)
              n1058 = To Unsigned Word Integer(number=w2770) -> (unsigned 16bit integer=w2772:u16)
              n1059 = local read "START"() -> (w2800:bool)
              n1060 = local read "STOP_endBlock"() -> (w2795:bool)
              n1061 = local read "STOP_endTrial"() -> (w2798:bool)
              n1062 = local read "STOP_abort"() -> (w2797:bool)
              n1063 = Replace Array Subset(array=w2775, new element=w2772, index=w2774) -> (w2773:u16[])
              n1064 = Not(x=w2800) -> (.not. x?=w2799:bool)
              n1065 = Compound Arithmetic op=OR(w2799, w2795, w2798, w2797) -> (w2796:bool)
              n1066 = Select(t=myRIO_BRig_RT__Case_Exp_stateList."endExp" ("Enum"), s=w2796, f=myRIO_BRig_RT__Case_Exp_stateList."empty_endBlock1" ("Enum")) -> (s? t:f=w2804:T2)
            }
            frame "endExp" {
            }
            frame "commConnect" {
              n1067 = call "myRIO_BRig_RT_comm_webdav_connect.vi"("input_password"="Host Password", "input_username"="Host UserName") -> ("output_Iconnected"=w2825:bool, "output_hSession"=w2843:T6)  [unwired: 7 in, 1 out]
              "Connected To Host?" <- w2825
              n1068 = case shown="False" w2825 {
                frame False {
                  n1069 = One Button Dialog(message="Connection Failed!\nData not being saved!") -> ()  [unwired: 1 in, 1 out]
                }
                frame True {
                }
              }
            }
            frame "commUpload_pre" {
              n1070 = Select(t=myRIO_BRig_RT__Case_Exp_stateList."commUpload_dataBlock" ("Enum"), s=w2850, f=myRIO_BRig_RT__Case_Exp_stateList."endTrial3") -> (s? t:f=w2848:T2)
            }
            frame "commUpload_dataBlock" {
              n1071 = call "myRIO_BRig_RT_comm_webdav_uploadFile__data.vi"("input_fileName_prefix"=w2871, "input_fileName"="dataBlock" ("input_filename"), "input_hSession"=w2873) -> ()  [unwired: 8 in, 1 out]
            }
            frame "commUpload_dataCurrent" {
              n1072 = call "myRIO_BRig_RT_comm_webdav_uploadFile__data.vi"("input_fileName_prefix"=w2892, "input_fileName"="dataCurrent" ("input_filename"), "input_hSession"=w2894) -> ()  [unwired: 8 in, 1 out]
            }
            frame "commUpload_dataExp" {
              n1073 = call "myRIO_BRig_RT_comm_webdav_uploadFile__data.vi"("input_fileName_prefix"=w2913, "input_fileName"="dataExp" ("input_filename"), "input_hSession"=w2915) -> ()  [unwired: 8 in, 1 out]
            }
            frame "commUpload_dataLC" {
              n1074 = call "myRIO_BRig_RT_comm_webdav_uploadFile__data.vi"("input_fileName_prefix"=w2934, "input_fileName"="dataLC" ("input_filename"), "input_hSession"=w2936) -> ()  [unwired: 8 in, 1 out]
            }
            frame "commUpload_dataTrial" {
              n1075 = call "myRIO_BRig_RT_comm_webdav_uploadFile__data.vi"("input_fileName_prefix"=w2958, "input_fileName"="dataTrial" ("input_filename"), "input_hSession"=w2960) -> ()  [unwired: 8 in, 1 out]
            }
            frame "saveData_dataBlock" {
              # "idxDataBlockR"
              # "idxDataBlockL"
              n1076 = call "myRIO_BRig_RT_dataCurrent_idxDataBlockL.vi"() -> ("output_idxDataBlock__L"=w2984:i32)  [unwired: 11 in]
              n1077 = call "myRIO_BRig_RT_dataCurrent_idxDataBlockR.vi"() -> ("output_idxDataBlock__R"=w2985:i32)  [unwired: 11 in]
              n1078 = Index Array(array=w2986, index #1=w2984, index #2=w2985) -> (element #1=w2983:u16, element #2=w2982:u16)
              n1079 = Greater?(x=w2983, y=w2982) -> (0:w2981:bool)
              n1080 = Select(t=w2983, s=w2981, f=w2982) -> (s? t:f=w2979:u16)
              n1081 = Increment(x=w2979) -> (x+1=w2978:u16)
              n1082 = To Long Integer(number=w2978) -> (32bit integer=w2977:i32)
              n1083 = Array Subset(array=w2980, length (row)=w2977) -> (w2976:u16[][])  [unwired: 3 in]
              n1084 = call "myRIO_BRig_RT_comm_webdav_saveArrayToFile__2D_u16.vi"("Array"=w2976, "input_filename"="dataBlock") -> ()  [unwired: 10 in]
            }
            frame "saveData_dataCurrent" {
              n1085 = call "myRIO_BRig_RT_comm_webdav_saveArrayToFile__1D_u16.vi"("Array"=w3005, "input_filename"="dataCurrent") -> ()  [unwired: 10 in]
            }
            frame "saveData_dataExp" {
              # "runTime"
              n1086 = Get Date/Time In Seconds() -> (seconds since 1Jan1904=w3033:timestamp)
              n1087 = To Double Precision Float(number=w3033) -> (double precision float=w3032:dbl)
              n1088 = call "myRIO_BRig_RT_dataExp_runTime_seconds.vi"() -> ("output_RunTime_minutes"=w3031:i32)  [unwired: 11 in]
              n1089 = Subtract(x=w3032, y=w3030) -> (x-y=w3027:dbl)
              n1090 = To Unsigned Word Integer(number=w3027) -> (unsigned 16bit integer=w3026:u16)
              n1091 = Replace Array Subset(array=w3025, new element=w3026, index=w3031) -> (w3028:u16[])
              n1092 = call "myRIO_BRig_RT_comm_webdav_saveArrayToFile__1D_u16.vi"("Array"=w3028, "input_filename"="dataExp") -> ()  [unwired: 10 in]
            }
            frame "saveData_dataLC" {
              n1093 = call "myRIO_BRig_RT_comm_webdav_saveArrayToFile__1D_u16.vi"("Array"=w3052, "input_filename"="dataLC") -> ()  [unwired: 10 in]
            }
            frame "saveData_dataTrial" {
              # "idxTrial"
              n1094 = call "myRIO_BRig_RT_dataCurrent_idxDataTrial.vi"() -> ("output_idxDataTrial"=w3077:i32)  [unwired: 11 in]
              n1095 = Index Array(array=w3078, index=w3077) -> (element=w3074:u16)
              n1096 = Increment(x=w3074) -> (x+1=w3073:u16)
              n1097 = To Long Integer(number=w3073) -> (32bit integer=w3072:i32)
              n1098 = Array Subset(array=w3075, length (row)=w3072) -> (w3076:u16[][])  [unwired: 3 in]
              n1099 = call "myRIO_BRig_RT_comm_webdav_saveArrayToFile__2D_u16.vi"("Array"=w3076, "input_filename"="dataTrial") -> ()  [unwired: 10 in]
            }
            frame "empty_endBlock1" {
            }
            frame "empty_endBlock2" {
            }
            frame "empty_endTrial1" {
            }
            frame "empty_endTrial2" {
            }
            frame "empty_endTrial3" {
            }
            frame "empty_endTrial4" {
            }
            frame "empty_endTrial5" {
            }
          }
          n1100 = Select(t=w1073, s=w1076, f=w1074) -> (s? t:f=w1075:bool)
          n1101 = case shown="True" w1147 {
            tunnel: w1144 -> [w1169 w1177]
            tunnel: w1146 -> [_ w1173]
            tunnel: w1145 -> [_ w1172]
            tunnel: w1050 -> [_ w1171]
            tunnel: w1114 -> [_ w1170]
            tunnel: [w1169 w1176] -> w1143
            tunnel: w1142 -> [w1168 w1175]
            tunnel: [w1168 w1174] -> w1141
            frame False {
            }
            frame True {
              n1102 = call "myRIO_BRig_RT__Case_Exp__recordLick.vi"("intput_state__trialEnd"=w1170, "intput_state__trialStart"=w1171, "input_lick__R"=w1172, "input_lick__L"=w1173, "input_dataCurrent"=w1175, "input_dataLick"=w1177) -> ("output_dataCurrent"=w1174:u16[], "output_dataLick"=w1176:u16[][])  [unwired: 4 in]
            }
          }
          n1103 = Or(x=w1116, y=w1117) -> (x .or. y?=w1103:bool)
          n1104 = Or(x=w1120, y=w1100) -> (x .or. y?=w1089:bool)
          n1105 = Or(x=w1099, y=w1121) -> (x .or. y?=w1115:bool)
          n1106 = Or(x=w1119, y=w1118) -> (x .or. y?=w1104:bool)
          n1107 = Or(x=w1148, y="STOP_abort") -> (x .or. y?=w1150:bool)
          n1108 = Or(x=w1079, y=w1080) -> (x .or. y?=w1077:bool)
          n1109 = Or(x=w1081, y=w1080) -> (x .or. y?=w1078:bool)
          n1110 = Select(t=w1062, s=w1063, f=w1061) -> (s? t:f=w1052:u16)
          n1111 = Select(t=w1064, s=w1066, f=w1065) -> (s? t:f=w1053:u16)
          n1112 = Select(t=u16 0, s=w1069, f=w1068) -> (s? t:f=w1051:u16)
          n1113 = xnode "Read/Write Control"("FPGA VI Reference In"=w1091, "error in"=w1090, "A1_SR"=w1104, "A3_SL"=w1103, "A6_Act"=w1075, "audioTrigger_L"=w1089, "audioAmp_L"=w1130, "audioFreq_L_kHz"=w1098, "audioTrigger_R"=w1115, "audioAmp_R"=w1131, "audioFreq_R_kHz"=w1132, "laserledMTrig"=w1077, "laserMTrig"=w1078) -> ("FPGA VI Reference Out"=w1140:refnum<k20>, "error out"=w1139:errorcluster, "AnaIn_0"=w1049:i16, "AnaIn_1"=w1048:i16)
          n1114 = local write "tempAI0"(w1049) -> ()
          n1115 = call "myRIO_BRig_RT_dataAnalog_enterData__PortC.vi"("input_iState"=w1050, "input_AI0"=w1049, "input_iEvent"=w1051, "input_AI1"=w1048, "input_iTrial"=w1052, "input_iBlock"=w1053, "input_index"=w1054, "input_dataAnalog"=w1072) -> ("output_dataAnalog"=w1071:u16[][])  [unwired: 3 in]
          n1116 = call "myRIO_BRig_RT_TCP.vi"("input_hTCP"=w1059, "input_AI1"=w1048, "input_AI0"=w1049, "input_I_connected_TCP"=w1055, "input_index"=w1054, "input_iBlock"=w1053, "input_iTrial"=w1052, "input_error"=w1057, "input_iEvent"=w1051, "input_iState"=w1050) -> ("output_hTCP"=w1058:refnum<k5>, "output_error"=w1056:errorcluster)  [unwired: 4 in]
          n1117 = node-c288() -> ()  [unwired: 1 in, 1 out]
          n1118 = Increment(x=w1051) -> (x+1=w1060:u16)
          n1119 = Increment(x=w1054) -> (x+1=w1070:i32)
          "cState" <- w1050
        }
        n1120 = node-c288(w994) -> ()  [unwired: 1 out]
        n1121 = flat-sequence {
          tunnel: w990 -> [w1039]
          tunnel: w989 -> [w1038]
          tunnel: [w1037] -> w982
          tunnel: [w1036] -> w981
          tunnel: [w1042] -> w983
          tunnel: [w1043] -> w988
          tunnel: w982 -> [w1043]
          tunnel: w981 -> [w1042]
          frame #0 {
            w1033 = u8 0
            w1034 = u16 0 ("AudioLeft_phase_inc")
            w1035 = FALSE
            n1122 = xnode "Read/Write Control"("FPGA VI Reference In"=w1039, "error in"=w1038, "Counts_Reset"=TRUE, "audioTrigger_L"=w1035, "audioFreq_L_kHz"=w1033, "audioAmp_L"=w1034, "audioTrigger_R"=w1035, "audioFreq_R_kHz"=w1033, "audioAmp_R"=w1034, "A3_SL"=w1035, "A1_SR"=w1035, "A6_Act"=w1035) -> ("FPGA VI Reference Out"=w1037:refnum<k20>, "error out"=w1036:errorcluster)
          }
          frame #1 {
            w1041 = FALSE ("START")
            n1123 = local write "START"(w1041) -> ()
            n1124 = local write "STOP_endTrial"(w1041) -> ()
            n1125 = local write "STOP_endBlock"(w1041) -> ()
          }
        }
        n1126 = stacked-sequence {
          tunnel: w966 -> [w1013 _]
          tunnel: w964 -> [w1014 _]
          tunnel: w963 -> [_ w1019]
          tunnel: w962 -> [_ w1018]
          tunnel: w961 -> [_ w1017]
          tunnel: w960 -> [w1007 _]
          tunnel: w934 -> [w1004 _]
          tunnel: w933 -> [w1003 _]
          frame #0 {
            n1127 = call "myRIO_BRig_RT_dataCurrent_idxDataLick.vi"() -> ("output_idxDataLick"=w1008:i32)  [unwired: 11 in]
            n1128 = Index Array(array=w1007, index=w1008) -> (element=w1010:u16)
            n1129 = Array Subset(array=w1004, length (row)=w1003) -> (w1005:u16[][])  [unwired: 3 in]
            n1130 = Increment(x=w1010) -> (x+1=w1011:u16)
            n1131 = call "myRIO_BRig_RT_comm_webdav_saveArrayToFile__1D_u16.vi"("Array"=w1014, "input_filename"="dataMTrig") -> ()  [unwired: 10 in]
            n1132 = To Long Integer(number=w1011) -> (32bit integer=w1009:i32)
            n1133 = Array Subset(array=w1013, length (row)=w1009) -> (w1012:u16[][])  [unwired: 3 in]
            n1134 = call "myRIO_BRig_RT_comm_webdav_saveArrayToFile__2D_u16.vi"("Array"=w1012, "input_filename"="dataLick") -> ()  [unwired: 10 in]
            n1135 = call "myRIO_BRig_RT_comm_webdav_saveArrayToFile__2D_u16.vi"("Array"=w1005, "input_filename"="dataAnalog") -> ()  [unwired: 10 in]
          }
          frame #1 {
            n1136 = case shown="True" w1019 {
              tunnel: w1018 -> [_ w1021]
              tunnel: w1017 -> [_ w1020]
              frame False {
              }
              frame True {
                n1137 = stacked-sequence {
                  tunnel: w1021 -> [w1023 w1030 w1032]
                  tunnel: w1020 -> [w1024 w1029 _]
                  frame #0 {
                    n1138 = call "myRIO_BRig_RT_comm_webdav_uploadFile__announce.vi"("input_addText"=TRUE, "input_fileName_prefix"=w1024, "intput_fileName"="curExp_end", "intput_hSession"=w1023) -> ("output_Isuccess"=w1022:bool)  [unwired: 6 in, 1 out]
                    n1139 = case shown="True" w1022 {
                      frame False {
                        n1140 = One Button Dialog(message="!!! Warning !!! Your data is located at C:\\BehaviorRig\\commTransfer") -> ()  [unwired: 1 in, 1 out]
                      }
                      frame True {
                        n1141 = Wait (ms)(milliseconds to wait=u32 20) -> ()  [unwired: 1 out]
                      }
                    }
                  }
                  frame #1 {
                    n1142 = call "myRIO_BRig_RT__endExp_sendData.vi"("input_fileName_prefix"=w1029, "input_hSession"=w1030) -> ()  [unwired: 8 in, 2 out]
                  }
                  frame #2 {
                    n1143 = local write "Connected To Host?"(FALSE ("Connected To Host?")) -> ()
                    n1144 = call <vilib>:"Close Session.vi"("session handle"=w1032) -> ()  [unwired: 14 in, 1 out]
                  }
                }
              }
            }
          }
        }
      }
    }
    n1145 = local read "STOP_abort"() -> (w43:bool)
  }
  n1146 = case shown="True" w3 {
    tunnel: w2 -> [_ w3232]
    tunnel: w1 -> [_ w3231]
    frame False {
    }
    frame True {
      n1147 = call "myRIO__TCP_disconnect_forWrite.vi"("input_error"=w3231, "input_hTCP"=w3232) -> ()  [unwired: 9 in, 1 out]
    }
  }
  n1148 = xnode "Read/Write Control"("FPGA VI Reference In"=w15, "error in"=w14, "FPGA_Stop"=TRUE) -> ("FPGA VI Reference Out"=w20:refnum<k20>, "error out"=w21:errorcluster)
  n1149 = xnode "Close FPGA VI Reference"("FPGA VI Reference In"=w20, "error in"=w21) -> ("error out"=w19:errorcluster)
  n1150 = call <vilib>:"Reset myRIO.vi"("error in (no error)"=w19) -> ()  [unwired: 10 in, 1 out]
